vi "main.vi"() -> ()   [LabVIEW 2015]
uses:
  <userlib>/atmcd32d.llb/Error Code Enum typedef.ctl
  <vilib>/Utility/miscctls.llb/LVPointDoubleTypeDef.ctl
  <userlib>/atmcd32d.llb/OutputAmplifier_type typedef.ctl
  <vilib>/Xenics Infrared Solutions/Xeneth LabVIEW API/VIs/Controls/Camara.ctl
  <vilib>/Platform/TimedLoop/XDataNode/timing_clust.ctl
  <vilib>/Platform/TimedLoop/XDataNode/nitl_modes.ctl
  <vilib>/Platform/TimedLoop/XDataNode/wakeup.ctl
  <userlib>/atmcd32d.llb/HSSpeed_type typedef.ctl
  <userlib>/atmcd32d.llb/ReadMode_mode typedef.ctl
  <vilib>/Utility/file.llb/Read Delimited Spreadsheet (DBL).vi
  <vilib>/Utility/file.llb/Write Delimited Spreadsheet (DBL).vi
  <vilib>/Platform/TimedLoop/XDataNode/XDataNode.xnode
  <vilib>/Platform/TimedLoop/XDataNode/XDNodeRunTimeDep.lvlib
  <vilib>/Xenics Infrared Solutions/Xeneth LabVIEW API/Xeneth.lvlib
panel:
  in  "velleman-power":bool caption="Power Control"
  out "shutdown-complete":bool
  in  "shutdown":bool
  out "laser on":bool
  out "shutdown-active":bool
  in  "view settings":T1(tab)
  in  "abort-acquisition":bool caption="Abort"
  in  "measure":bool
  in  "NKT":bool
  in  "align-mode":bool caption="align mode"
  in  "continuos-save":bool
  in  "refresh display":bool=TRUE caption="refresh"
  in  "autoscale":bool=TRUE
  in  "background":bool=TRUE
  in  "Save current Spectrum":bool
  in  "File Name":string="spectrum"
  in  "BG shutter":T2(radio)=enum."with Open Shutter" caption="Shutter during background measurement"
  in  "select background":enum16{"skip", "single", "multiple"}(ring)=enum."single"
  out "Progress":u8(slide) scale=0.0..100.0
  out "ready":bool
  out "acquiring":bool
  out "background":bool
  out "measurement-finished":bool caption="finished"
  out "Acq Error":errorcluster
  out "next action":T3(ring)
  in  "Spectra":enum32{"Spectrum", "Image"}(tab)
  out "Data Plot":cluster{"wavelength array":sgl[], "array":i32[]}(graph)
  out "Detected Image":i32[][](graph)
  in  "Main Panel":T4(tab)=enum."init"
  in  "config":T5(tab)
  out "lightsource-set":bool
  out "NKT Output":T6 {"UV Wavelength (nm)" format="%.1f"; "Long Wavelength (nm)" format="%.1f"; "Short Wavelength (nm)" format="%.1f"; "Feedback Level" format="%.1f%%"; "Power Level" format="%.1f%%"; "Temp (°C)" format="%.1f"}
  in  "NKT Input":T7={"Emission"=FALSE, "Operation Mode"=FALSE, "Power Level"=5.0, "Feedback Level"=0.0, "Short Wavelength (nm)"=560.0, "Long Wavelength (nm)"=580.0, "UV Wavelength (nm)"=400.0} {"UV Wavelength (nm)" min=350.0 max=480.0 step=1.0 format="%.1f"; "Long Wavelength (nm)" min=400.0 max=850.0 step=0.5 format="%.1f"; "Short Wavelength (nm)" min=400.0 max=850.0 step=0.5 format="%.1f"; "Feedback Level" min=0.0 max=90.0 step=0.1 format="%.1f%%"; "Power Level" min=5.0 max=100.0 step=0.1 format="%.1f%%"}
  out "velleman-power-status":bool
  out "WL Power (nm)":i32 caption="Wavelength (nm)"
  out "Power (µW)":dbl format="%.6f"
  in  "Perform Auto Zero":bool
  in  "lightsource-bp":u16(ring) items=["(6,4)"=590, "(9,1)"=690, "(8,3)"=660, "(6,5)"=570, "(7,5)"=650, "--"=0]
  out "wavelength-limits":T8
  out "spectrograph-status":T9
  out "spectrograph-output":T10={"Slit Width (µm)"=50.0, "Grating"=3, "Central Wavelength (nm)"=1000.0, "Filter"=4, "Shutter"=0} caption="Spectrograph Output" {"Shutter" items=["Closed", "Open"]; "Slit Width (µm)" min=10.0 max=2500.0 step=0.1 format="%.1f"; "Grating" items=["500 blz 300l/mm"=1, "1200 blz 300l/mm"=2, "1250 blz 150l/mm"=3]; "Filter" items=["Empty"=5, "Longpass 900 nm"=4, "Longpass 715 nm"=3, "Longpass 475 nm"=2, "Longpass 320 nm"=1]; "Central Wavelength (nm)" min=200.0 max=2000.0 step=0.1 format="%.2f"}
  in  "spectrograph-input":T10={"Slit Width (µm)"=250.0, "Grating"=2, "Central Wavelength (nm)"=950.0, "Filter"=5, "Shutter"=1} caption="Spectrograph Input" {"Shutter" items=["Close", "Open"]; "Slit Width (µm)" min=10.0 max=2500.0 step=0.1 format="%.1f"; "Grating" items=["500 blz 300l/mm"=1, "1200 blz 300l/mm"=2, "1250 blz 150l/mm"=3]; "Filter" items=["Longpass 320 nm"=1, "Longpass 475 nm"=2, "Longpass 715 nm"=3, "Longpass 900 nm"=4, "Empty"=5]; "Central Wavelength (nm)" min=0.0 max=2000.0 step=0.1 format="%.1f"}
  out "spectrograph-reset-status":T11
  in  "spectrograph-reset-input":cluster{"grating":bool, "slit":bool}={"grating"=TRUE, "slit"=FALSE} caption="Spectrograph Reset Actions"
  in  "Exposure Time":dbl=0.20000000298023224 min=0.009999999776482582 step=0.009999999776482582 format="%.2f"
  out "Exposure Time Read":sgl format="%.2g"
  out "exposure time":bool
  out "detector":bool
  in  "Detector Select":u16(ring) caption="Camera" items=["Newton", "iDus", "Clara", "Xeva"]
  out "Current Detector":string
  in  "camera-settings":enum32{"Andor", "Xenics", "Andor-settings"}(tab)
  out "DLL error code":u32
  in  "iDus Type":T12
  in  "center":u16=102
  in  "height":u16=50 min=1 max=256
  in  "pre-amp 2":u8 caption="pre-amp" max=2 step=1
  in  "HBinning":u16(ring)=1 items=["1x"=1, "2x"=2, "4x"=4, "8x"=8, "16x"=16]
  out "binning":bool
  in  "HSSpeed 2":u8 max=0 step=1
  out "pre-amp 3":bool
  out "pre-amp":dbl caption="x"
  out "HSSpeed 3":bool
  out "HSSpeed":dbl caption="Mhz"
  out "ADchannel 2":bool
  in  "ADchannel":u8 max=0 step=1
  out "xeva-parameters":T13 {"time" format="%#.2f"}
  out "Cooling Read":cluster{"iDus":i32, "Newton":i32, "Clara":i32}={"iDus"=25, "Newton"=25, "Clara"=25}
  in  "detector-warmup":bool=TRUE
  in  "readout mode 2":u16(ring) items=["Full Vertical Binning", "Image", "Vertical Binning"]
  out "readout mode":bool
  out "nanostage moving":bool caption="moving"
  in  "z-stepsize":dbl=0.25 format="%.3f"
  in  "xy stepsize":dbl=0.1 format="%.3f"
  in  "x-axis":dbl=150.0 min=0.0 max=300.0 step=0.1 format="%.3f"
  in  "y-axis":dbl=150.0 min=0.0 max=300.0 step=0.1 format="%.3f"
  in  "z-axis":dbl=150.0 min=0.0 max=300.0 step=0.25 format="%.3f"
  in  "switch U/D":bool=TRUE
  in  "switch L/R":bool=TRUE
  out "stage-error":bool=TRUE
  out "click cursor position":T14
  out "getValues":cluster{"postion":dbl[], "status":bool[]} {"postion" format="%05.1f"}
  in  "stage-autozero":bool=TRUE caption="autozero on init"
  in  "laser-freeze":bool caption="glue scaling\nto image"
  in  "image-laser-position":T15={"laser-x-position"=520, "laser-y-position"=696}
  in  "magnification":dbl=83.3333333 caption="x" min=1.0 max=200.0 step=0.0001
  out "pixel scaling":bool
  out "Pixel Scaling":T16
  in  "laser-offset":bool caption="laser-is-zero"
  in  "magnification":bool
  in  "timed-shutdown":bool caption="shutdown"
  in  "timed-counter-stop":u32=1
  out "timed-counter":u32
  in  "timed-type":enum16{"spectrum", "AutoStage", "PLE"}(ring) caption="measurment type"
  out "waiting":u8(slide) scale=0.0..100.0
  in  "timed-start":bool caption="start"
  out "timed-timestamp":timestamp
  in  "timed-wait":dbl caption="wait / s"
  in  "cycle-save-coordinates":bool caption="save"
  in  "cycle-load-coordinates":bool caption="load"
  out "Coordinate Graph":dbl[][](graph)
  out "cycle-time":i32 caption="time/min"
  in  "cycle-iterator":i32 caption="iterator"
  out "cycle-num":i32 caption="total"
  out "Slide":u8(slide) scale=0.0..100.0
  in  "Cycle Cluster":T17={"cycle-x-mod"=151, "cycle-x-range-min"=0.0, "cycle-x-range-max"=300.0, "cycle-x-step"=4.0, "cycle-y-mod"=1, "cycle-y-range-min"=0.0, "cycle-y-range-max"=300.0, "cycle-y-step"=2.0, "cycle-z-mod"=0, "cycle-z-range-min"=150.0, "cycle-z-range-max"=0.0, "cycle-z-step"=0.0}
  in  "autostage-start":bool caption="start"
  in  "cycle-save-data":bool=TRUE caption="save"
  out "coordinates":dbl[][](array[numeric])
  in  "stage-timed-type":enum16{"spectrum", "PLE"}(ring) caption="measurment type"
  out "excitation":dbl[][](array[numeric])
  in  "PLE VIS/UV Panel":enum32{"SuperK Varia (VIS)"}(tab)
  in  "PLE Wavelength":T18={"WL Stepsize (nm)"=10, "WL Bandpass (nm)"=25, "Max WL VIS (nm)"=750, "Min WL VIS (nm)"=550} {"Min WL VIS (nm)" min=450 max=699 step=1; "Max WL VIS (nm)" min=501 max=850 step=1; "WL Bandpass (nm)" items=["5"=5, "10"=10, "25"=25, "50"=50, "75"=75, "100"=100]; "WL Stepsize (nm)" items=["5"=5, "10"=10, "25"=25, "50"=50, "75"=75, "100"=100]}
  out "PLE Acquisition\nfinished?":bool
  in  "Start PLE Scan":bool
  in  "PLE File Name":string="map" caption="File Name"
  out "Present Scan":string
  in  "STOP PLE":bool
  out "Acquisition Status PLE":T19=enum."DRV_NOT_INITIALIZED" caption="Acquisition Status"
  out "Elapsed Time (s)":dbl caption="elapsed time [s]" format="%.2f"
  out "Progress":dbl format="%.1f%%"
  out "Number of Scans":i32
  out "PLE-Map":i32[][](graph)
  out "PLE loop count":i32
  out "xeva init":bool caption="xeva"
  out "ANDOR init":bool caption="ANDOR"
  out "velleman init":bool caption="velleman"
  out "cameras init":bool caption="cameras"
  out "nanostage init":bool caption="nanostage"
  out "lightsource":bool
  out "powermeter init":bool caption="powermeter"
  out "spectrograph":bool
  in  "init xeva":bool caption="xeva"
  in  "init cameras":bool caption="cameras"
  in  "init spectrograph":bool caption="spectrograph"
  in  "init powermeter":bool caption="powermeter"
  in  "init nanostage":bool caption="nanostage"
  in  "init lightsource":bool caption="lightsource"
  in  "Cooling Set":T20={"iDus"=FALSE, "idus-temp"=-90, "Newton"=FALSE, "newton-temp"=-70, "Clara"=FALSE, "clara-temp"=-55, "Xeva"=FALSE, "xeva-temp"=-70} {"xeva-temp" min=-70 max=20 step=5; "clara-temp" min=-55 max=20 step=5; "newton-temp" min=-90 max=20 step=5; "idus-temp" min=-90 max=20 step=5}
  out "general-camera-status":T21
  in  "Tab Control":T22(tab)
  out "xeva-camref":T23
  in  "lightsource-visa":refnum<visa-resource-name>="COM3"
  in  "powermeter visa":refnum<visa-resource-name>="USB0::0x1313::0x8079::P1000487::INSTR"
  out "CCD Handle":i32
  out "InGaAs Handle":i32
  out "All conn. axes":string[](array[string])
  out "Handle":cluster{"iDus":i32, "Newton":i32, "Clara":i32} caption="Handle Cluster"
  out "Background Array":i32[](array[numeric])
  out "Raw Signal Array":i32[](array[numeric])
  out "Background Array PLE":i32[](array[numeric])
  out "Raw Signal Array PLE":i32[](array[numeric])
  out "Power during measurement":dbl format="%#_13g"
  out "y-scale array":sgl[](array[numeric])
  out "x-scale array":sgl[](array[numeric])
  out "stage error message":string
  out "error out":errorcluster
  out "xenics-status-cluster":T24
  out "andor-status-cluster":T25={"Newton Init"=FALSE, "Newton Cooling"=FALSE, "Newton Parameters "=FALSE, "iDus Init"=FALSE, "iDus Cooling"=FALSE, "iDus Parameters"=FALSE, "Clara Init"=FALSE, "Clara Cooling"=FALSE, "Clara Parameters"=FALSE, "Newton Cooler StatusCode"=enum."DRV_TEMPERATURE_NOT_SUPPORTED", "iDus Cooler StatusCode"=enum."DRV_TEMPERATURE_NOT_SUPPORTED", "Clara Cooler StatusCode"=enum."DRV_TEMPERATURE_NOT_SUPPORTED"} caption="Cooling Status"
  # "Powermeter Status"
  # "spectrograph reset"
  # "Cycle"
  # "step\n[µm]"
  # "cycle mod"
  # "range\n[µm]"
  # "x-axis"
  # "y-axis"
  # "z-axis"
  # "Central Wavelength (nm)"
  # "Init"
  # "Cooling"
  # "Parameters"
  # "Newton"
  # "iDus"
  # "Clara"
  # "Xeva"
  # "Init"
  # "Cooling"
  # "Parameters"
  # "Xeva"
  # "Init"
  # "Cooling"
  # "Parameters"
  # "Newton"
  # "iDus"
  # "Clara"
  # "Clara"
  # "iDus"
  # "Newton"
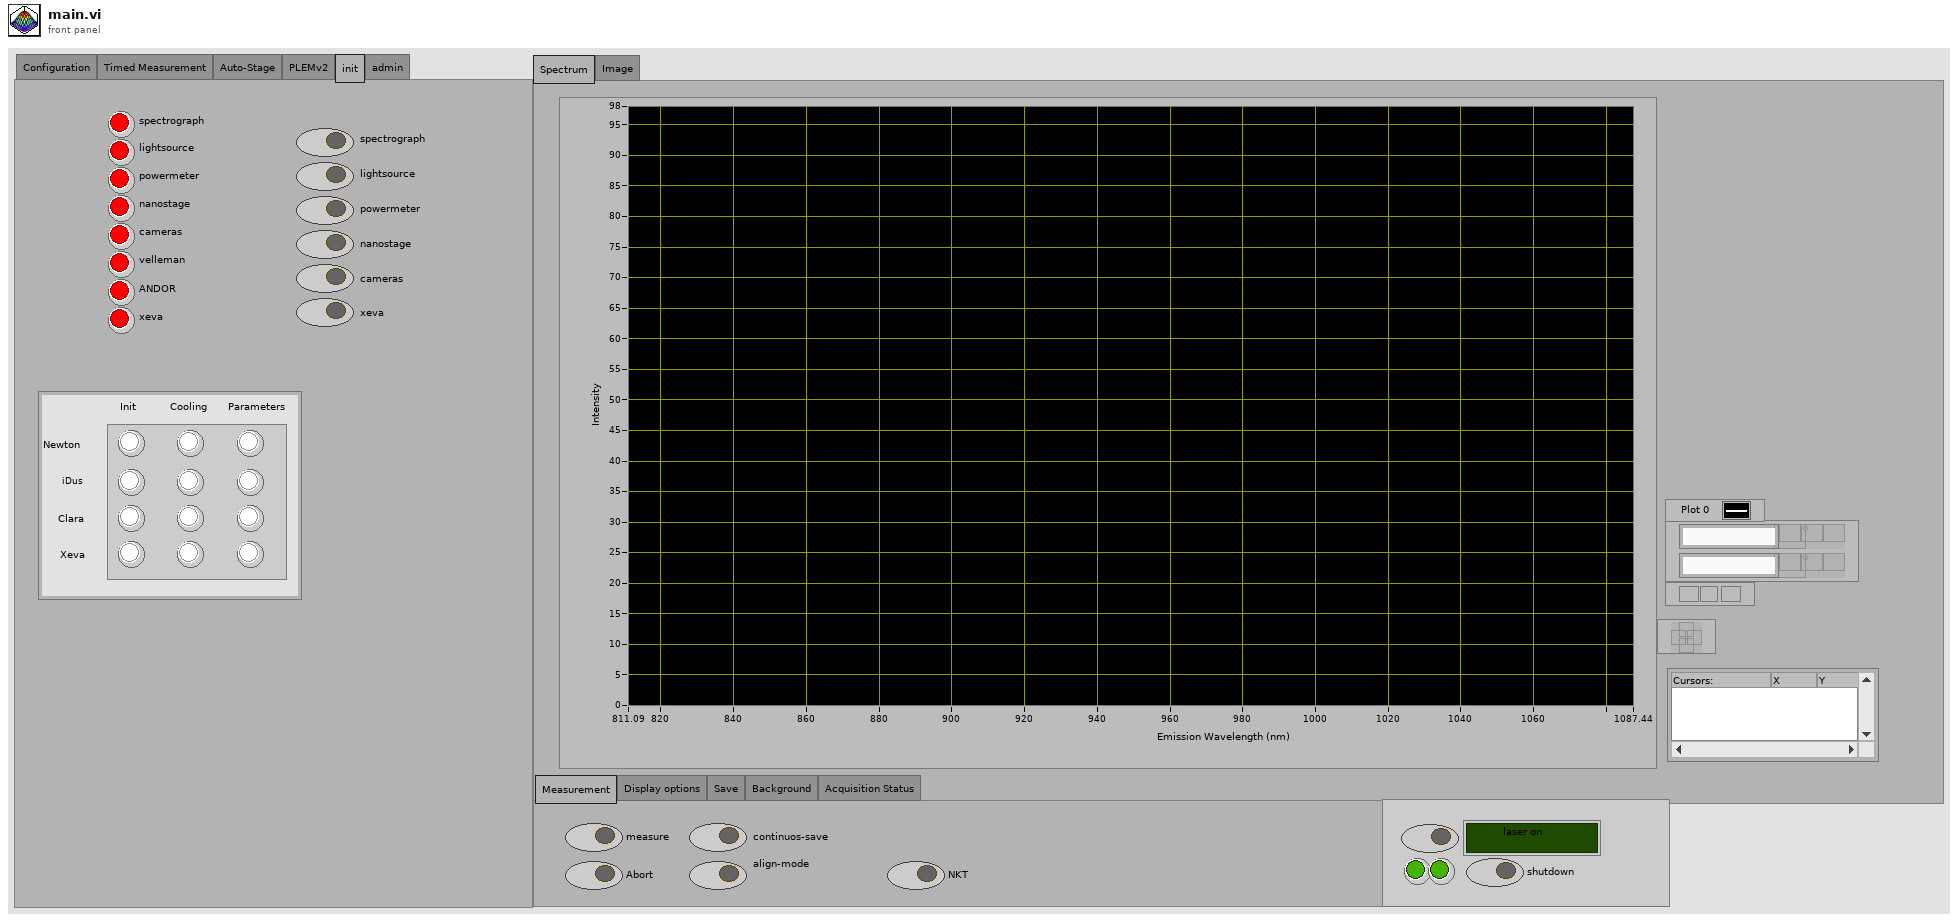
[diagram p1: front panel]
types:
  T1 = enum32{"Measurement", "Display options", "Save", "Background", "Acquisition Status"}
  T2 = enum32{"with Closed Shutter", "with Open Shutter"}
  T3 = enum16{"noop", "set background", "set measurement", "start acquisition", "abort", "get Data", "check progress", "restart acquisition", "start", "acquisition finished", "measurement finished", "wait to continue"}
  T4 = enum32{"Configuration", "Timed Measurement", "Auto-Stage", "PLEMv2", "init", "admin"}
  T5 = enum32{"Lightsource", "Spectrograph", "Camera", "Nanostage", "image"}
  T6 = cluster{"Emission":bool, "Operation Mode":string, "Power Level":dbl, "Feedback Level":dbl, "Short Wavelength (nm)":dbl, "Long Wavelength (nm)":dbl, "UV Wavelength (nm)":dbl, "Temp (°C)":dbl}
  T7 = cluster{"Emission":bool, "Operation Mode":bool, "Power Level":dbl, "Feedback Level":dbl, "Short Wavelength (nm)":dbl, "Long Wavelength (nm)":dbl, "UV Wavelength (nm)":dbl}
  T8 = cluster{"wl-start":dbl, "wl-step":dbl, "wl-end":dbl}
  T9 = cluster{"Slit":bool, "Diffraction Grating":bool, "Central Wavelength":bool, "Filter":bool, "Shutter":bool}
  T10 = cluster{"Slit Width (µm)":dbl, "Grating":u16, "Central Wavelength (nm)":dbl, "Filter":u16, "Shutter":u16}
  T11 = cluster{"Wavelength Reset OK":bool, "Slit Reset OK":bool}
  T12 = typedef "OutputAmplifier_type typedef.ctl" = enum16{"Standard EMCCD gain register", "Conventional CCD register"}
  T13 = cluster{"width":u32, "height":u32, "time":dbl, "temperature":dbl, "temperature-setpoint":dbl}
  T14 = typedef "LVPointDoubleTypeDef.ctl" = cluster{"X":dbl, "Y":dbl}
  T15 = cluster{"laser-x-position":u16, "laser-y-position":u16}
  T16 = cluster{"first x":sgl, "size x":u16, "deltax":dbl, "first y":sgl, "size y":u16, "deltay":dbl, "unit":string}
  T17 = cluster{"cycle-x-mod":i32, "cycle-x-range-min":dbl, "cycle-x-range-max":dbl, "cycle-x-step":dbl, "cycle-y-mod":i32, "cycle-y-range-min":dbl, "cycle-y-range-max":dbl, "cycle-y-step":dbl, "cycle-z-mod":i32, "cycle-z-range-min":dbl, "cycle-z-range-max":dbl, "cycle-z-step":dbl}
  T18 = cluster{"WL Stepsize (nm)":i32, "WL Bandpass (nm)":u16, "Max WL VIS (nm)":i32, "Min WL VIS (nm)":i32}
  T19 = typedef "Error Code Enum typedef.ctl" = enum32{"N/A (0)", "DRV_ERROR_CODES", "DRV_SUCCESS", "DRV_VXDNOTINSTALLED", "DRV_ERROR_SCAN", "DRV_ERROR_CHECK_SUM", "DRV_ERROR_FILELOAD", "DRV_UNKNOWN_FUNC", "DRV_ERROR_VXD_INIT", "DRV_ERROR_ADDRESS", "DRV_ERROR_PAGELOCK", "DRV_ERROR_PAGEUNLOCK", "DRV_ERROR_BOARDTEST", "DRV_ERROR_ACK", "DRV_ERROR_UP_FIFO", "DRV_ERROR_PATTERN", "N/A (16)", "DRV_ACQUISITION_ERRORS", "DRV_ACQ_BUFFER", "DRV_ACQ_DOWNFIFO_FULL", "DRV_PROC_UNKONWN_INSTRUCTION", "DRV_ILLEGAL_OP_CODE", "DRV_KINETIC_TIME_NOT_MET", "DRV_ACCUM_TIME_NOT_MET", "DRV_NO_NEW_DATA", "N/A (25)", "DRV_SPOOLERROR", "N/A (27)", "N/A (28)", "N/A (29)", "N/A (30)", "N/A (31)", "N/A (32)", "DRV_TEMPERATURE_CODES", "DRV_TEMPERATURE_OFF", "DRV_TEMPERATURE_NOT_STABILIZED", "DRV_TEMPERATURE_STABILIZED", "DRV_TEMPERATURE_NOT_REACHED", "DRV_TEMPERATURE_OUT_RANGE", "DRV_TEMPERATURE_NOT_SUPPORTED", "DRV_TEMPERATURE_DRIFT", "N/A (41)", "N/A (42)", "N/A (43)", "N/A (44)", "N/A (45)", "N/A (46)", "N/A (47)", "N/A (48)", "DRV_GENERAL_ERRORS", "DRV_INVALID_AUX", "DRV_COF_NOTLOADED", "DRV_FPGAPROG", "DRV_FLEXERROR", "DRV_GPIBERROR", "N/A (55)", "N/A (56)", "N/A (57)", "N/A (58)", "N/A (59)", "N/A (60)", "N/A (61)", "N/A (62)", "N/A (63)", "DRV_DATATYPE", "DRV_DRIVER_ERRORS", "DRV_P1INVALID", "DRV_P2INVALID", "DRV_P3INVALID", "DRV_P4INVALID", "DRV_INIERROR", "DRV_COFERROR", "DRV_ACQUIRING", "DRV_IDLE", "DRV_TEMPCYCLE", "DRV_NOT_INITIALIZED", "DRV_P5INVALID", "DRV_P6INVALID", "DRV_INVALID_MODE", "DRV_INVALID_FILTER", "DRV_I2CERRORS", "DRV_I2CDEVNOTFOUND", "DRV_I2CTIMEOUT", "DRV_P7INVALID", "N/A (84)", "N/A (85)", "N/A (86)", "N/A (87)", "N/A (88)", "N/A (89)", "DRV_IOCERROR", "DRV_VRMVERSIONERROR"}
  T20 = cluster{"iDus":bool, "idus-temp":i32, "Newton":bool, "newton-temp":i32, "Clara":bool, "clara-temp":i32, "Xeva":bool, "xeva-temp":i32}
  T21 = cluster{"Newton Init":bool, "Newton Cooling":bool, "Newton Parameters ":bool, "iDus Init":bool, "iDus Cooling":bool, "iDus Parameters":bool, "Clara Init":bool, "Clara Cooling":bool, "Clara Parameters":bool, "Xeva-init":bool, "xeva-cooling":bool, "xeva-parameters":bool}
  T22 = enum32{"ref/visa", "variables", "data", "status"}
  T23 = typedef "Xeneth.lvlib/Camara.ctl" = refnum<k1>
  T24 = cluster{"Xeva-init":bool, "xeva-cooling":bool, "xeva-parameters":bool, "xeva-error":string}
  T25 = cluster{"Newton Init":bool, "Newton Cooling":bool, "Newton Parameters ":bool, "iDus Init":bool, "iDus Cooling":bool, "iDus Parameters":bool, "Clara Init":bool, "Clara Cooling":bool, "Clara Parameters":bool, "Newton Cooler StatusCode":T19, "iDus Cooler StatusCode":T19, "Clara Cooler StatusCode":T19}
  T26 = typedef "XDNodeRunTimeDep.lvlib/timing_clust.ctl" = cluster{"Expected End [f-1]":u64, "Actual End [f-1]":u64, "Finished Late? [f-1]":bool, "Expected End [i-1]":u64, "Actual End [i-1]":u64, "Finished Late? [i-1]":bool, "Expected Start [i]":u64, "Actual Start [i]":u64, "Expected Start [f]":u64, "Actual Start [f]":u64, "Source Name":string, "Structure Name":string, "Period":i64, "Deadline":i64, "Offset":i64, "Start":i64, "Priority":i32, "Timeout":i32, "Mode":T27, "Wakeup Reason":T28, "Error":errorcluster, "Source Type":string, "Secondary Source Type":string, "Global End Time":u64, "Global Start Time":u64, "Frame Duration":u64, "Iteration Duration":u64, "Assigned CPU":i32, "I/O Scan Engine Mode":u32}
  T27 = typedef "XDNodeRunTimeDep.lvlib/nitl_modes.ctl" = enum32{"No Change", "Process missed periods, maintain original phase", "Discard missed periods, maintain original phase", "Process missed periods, ignore original phase", "Discard missed periods, ignore original phase"}
  T28 = typedef "XDNodeRunTimeDep.lvlib/wakeup.ctl" = enum32{"Normal", "Aborted", "Asynchronous wakeup", "Timing source error", "Timed loop error", "Timeout"}
  T29 = cluster{"Wavelength Reset":bool, "Slit Reset":bool}
  T30 = typedef "HSSpeed_type typedef.ctl" = enum16{"EM Amp", "Conventional Amp"}
  T31 = enum8{"Enabled", "Disabled", "Disabled and Grayed Out"}
  T32 = typedef "ReadMode_mode typedef.ctl" = enum16{"Full Vertical Binning", "Multi-Track", "Random-Track", "Single-Track", "Image"}
  T33 = cluster{"Slit Width (µm)":dbl, "Diffraction Grating":u16, "Central Wavelength (nm)":dbl, "Filter":u16, "Shutter":u16}
  T34 = cluster{"Slit":bool, "Diffraction Grating":bool, "Filter":bool, "Central Wavelength":bool, "Shutter":bool}
  T35 = cluster{"Emission On/Off external":bool, "Feedback Level external":dbl, "Power/Feedback Mode external":bool, "Power Level external":dbl}
  T36 = cluster{"Emission On/Off external":bool, "Feedback Level external":bool, "Power/Feedback Mode external":bool, "Power Level external":bool}
  T37 = cluster{"Slit Width (µm)":bool, "Grating":bool, "Central Wavelength (nm)":bool, "Filter":bool, "Shutter":bool}
  T38 = cluster{bool, bool, bool, "Filter":bool, "Shutter":bool}
  T39 = enum32{"Lightsource", "Spectrograph", "Detectors", "Nanostage", "image"}
  T40 = cluster{"Newton Init":bool, "Newton Cooling":bool, "Newton Parameters ":bool, "iDus Init":bool, "iDus Cooling":bool, "iDus Parameters":bool, "Clara Init":bool, "Clara Cooling":bool, "Clara Parameters":bool, "Newton Cooler StatusCode":bool, "iDus Cooler StatusCode":bool, "Clara Cooler StatusCode":bool}
  T41 = cluster{"Xeva-init":bool, "xeva-cooling":bool, "xeva-parameters":bool, "xeva-error":bool}
  T42 = typedef "LVPoint32TypeDef.ctl" = cluster{"Horizontal":i32, "Vertical":i32}
  T43 = cluster{"acquiring out":bool, "Progress":u8, "background":bool, "timer":u32, "finished":bool}
  T44 = enum16{"noop", "set background", "set measurement", "start acquisition", "abort", "get Data", "check progress", "restart acquisition", "start", "finished"}
  T45 = cluster{"detector":u16, "HBinning":u16, "readout mode":u16, "ready":bool, "Exposure Time Read":sgl, "select background":enum16{"skip", "single", "multiple"}, "xeva-camref":T23}
  T46 = enum16{"noop", "set background", "set measurement", "start acquisition", "abort", "get Data", "check progress", "restart acquisition", "start"}
  T47 = enum16{"noop", "set background", "set measurement", "start acquisition", "abort", "get Data", "check progress", "restart acquisition", "start", "acquisition finished", "start next measurement", "wait to continue"}
  T48 = cluster{"laser-x-position":bool, "laser-y-position":bool}
  T49 = cluster{"x-axis":dbl, "y-axis":dbl, "z-axis":dbl}
  T50 = cluster{"x-axis":bool, "y-axis":bool, "z-axis":bool}
  T51 = cluster{"Emission":bool, "Operation Mode":bool, "Power Level":bool, "Feedback Level":bool, "Short Wavelength (nm)":bool, "Long Wavelength (nm)":bool, "UV Wavelength (nm)":bool}
  T52 = cluster{"x-scale array":sgl[], "Raw Signal Array":i32[]}
  T53 = cluster{"cycle-x-mod":bool, "cycle-x-range-min":bool, "cycle-x-range-max":bool, "cycle-x-step":bool, "cycle-y-mod":bool, "cycle-y-range-min":bool, "cycle-y-range-max":bool, "cycle-y-step":bool, "cycle-z-mod":bool, "cycle-z-range-min":bool, "cycle-z-range-max":bool, "cycle-z-step":bool}
  T54 = cluster{"image-laser-position":cluster{"laser-x-position":u16, "laser-y-position":u16}, "magnification":dbl}
  T55 = cluster{"x-axis":dbl, "y-axis":dbl, "z-axis":dbl, "switch U/D":bool, "switch L/R":bool}
  T56 = cluster{"Current Detector":string, "readout mode":u16, "Hbinning":u16, "Exposure Time":sgl, "Cooling Read":cluster{"iDus":i32, "Newton":i32, "Clara":i32}, "pre-amp":dbl, "HSSpeed":dbl}
  T57 = cluster{"BG shutter":enum32{"with Closed Shutter", "with Open Shutter"}, "select background":enum16{"skip", "single", "multiple"}}
  T58 = cluster{"Loop Indicator":i32, "Number of Scans":i32, "True Step Size (nm) ":i32, "Wavelength Bandpass (nm)":i32, "Min Central Wavelength (nm)":i32}
  T59 = cluster{"Calibration Mode":bool, "File Name":string, "User Name":string, "Aborted?":bool, "NKT System":enum32{"SuperK Varia (VIS)", "Extend-UV"}}
  T60 = cluster{"Min WL VIS (nm)":i32, "Max WL VIS (nm)":i32, "WL Bandpass (nm)":i32, "WL Stepsize (nm)":i32}
  T61 = cluster{"Min Central Wavelength (nm)":i32, "Wavelength Bandpass (nm)":i32, "True Step Size (nm) ":i32, "Number of Scans":i32}
  T62 = cluster{"wavelength array":sgl[], "Data To Plot Array":i32[], "Raw Signal Array PLE":i32[], "Background Array PLE":i32[]}
  T63 = cluster{"WL Stepsize (nm)":i32, "Max WL VIS (nm)":i32, "Max WL VIS (nm)":i32, "Min WL VIS (nm)":i32}
  T64 = cluster{"WL Stepsize (nm)":bool, bool, "Max WL VIS (nm)":bool, "Min WL VIS (nm)":bool}
  T65 = cluster{"Emission":bool, "Operation Mode":string, "Power Level":dbl, "Feedback Level":dbl, "Short Wavelength (nm)":i32, "Long Wavelength (nm)":i32, "UV Wavelength (nm)":i32, "Temp (°C)":dbl}
  T66 = cluster{"Min Central Wavelength (nm)":i32, "Wavelength Bandpass (nm)":i32, "True Step Size (nm) ":i32, "Number of Scans":i32, i32}
  T67 = cluster{"Min Central Wavelength (nm)":i32, "Wavelength Bandpass (nm)":i32, "True Step Size (nm) ":i32, "Number of Scans":i32, "Loop Indicator":i32}
  T68 = cluster{"UV Wavelength (nm)":i32, "Short Wavelength (nm)":dbl, "Long Wavelength (nm)":dbl}
  T69 = cluster{"x-scale array":sgl[], "Background Array PLE":i32[]}
  T70 = cluster{"wavelength array":sgl[], "Data To Plot Array":i32[]}
  T71 = cluster{"Y Scale.Flipped":bool, "color table":u32[], dbl, dbl, dbl, dbl, sgl, sgl, sgl, dbl, "new picture":picture}
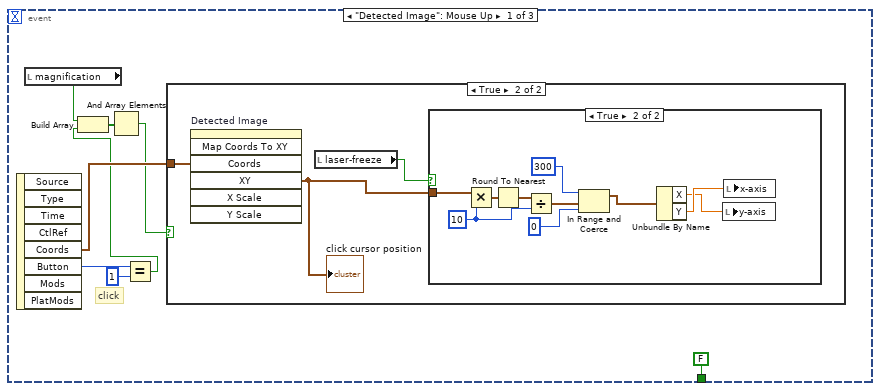
[diagram p2: hidden frame]
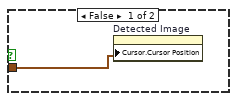
[diagram p4: hidden frame]
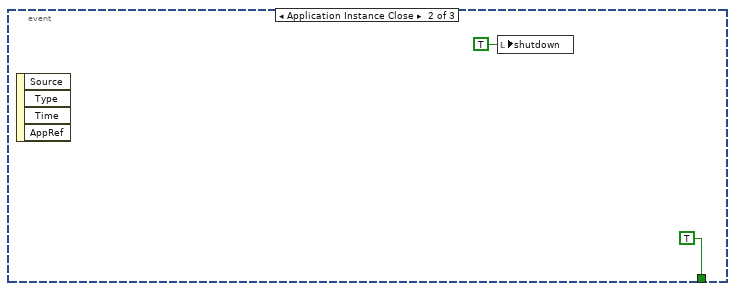
[diagram p5: hidden frame]
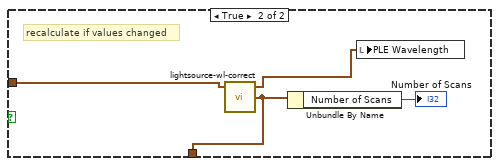
[diagram p7: hidden frame]
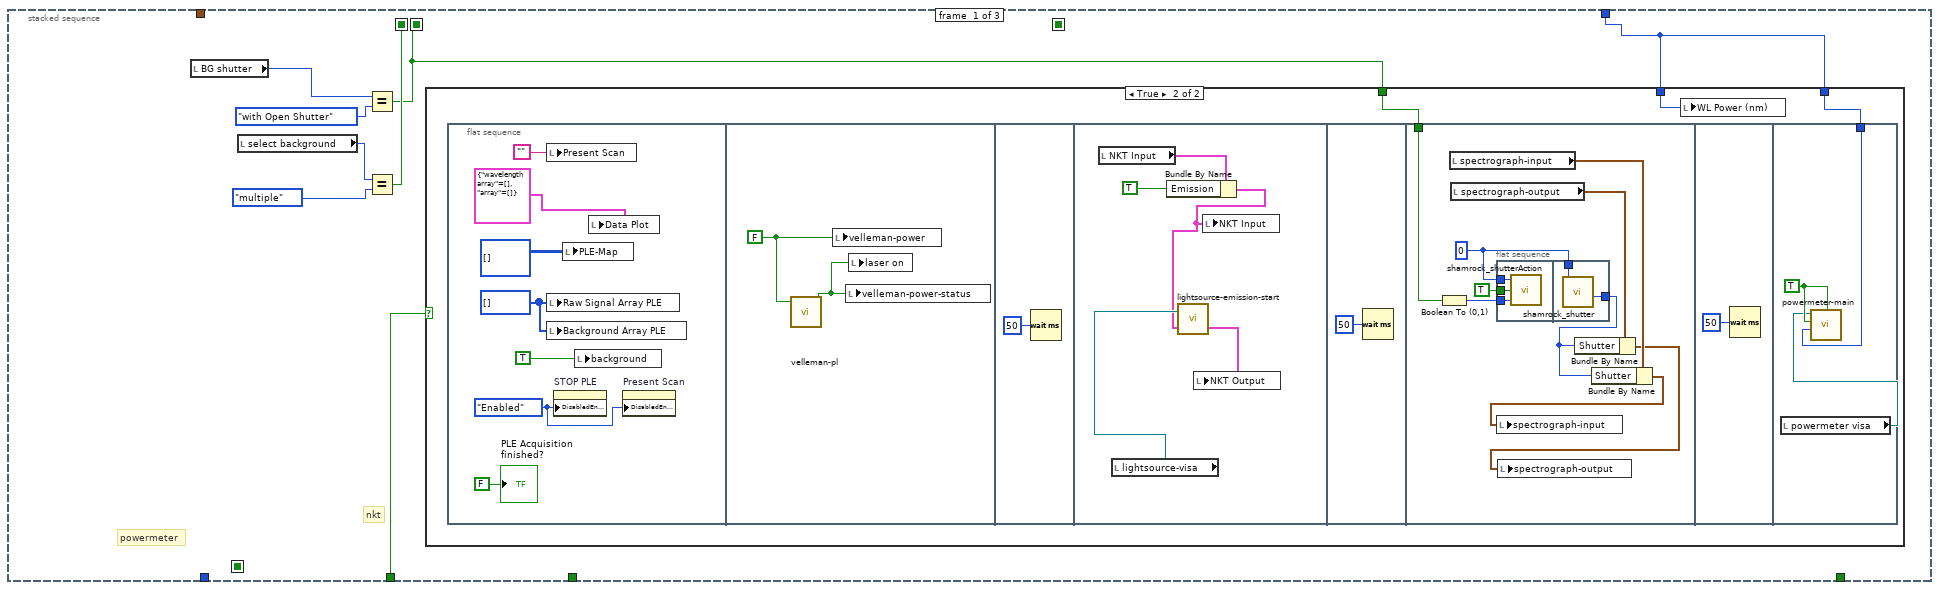
[diagram p9: hidden frame]
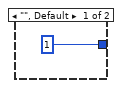
[diagram p11: hidden frame]
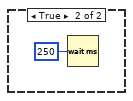
[diagram p12: hidden frame]
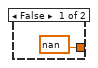
[diagram p13: hidden frame]
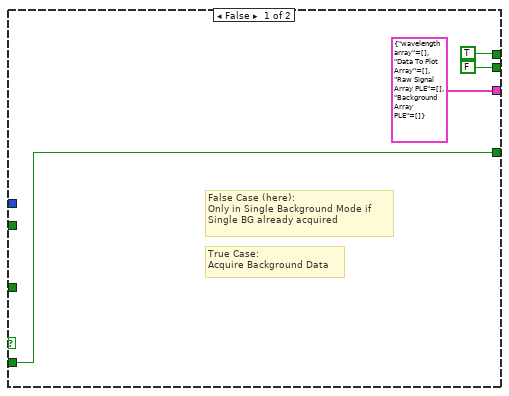
[diagram p14: hidden frame]
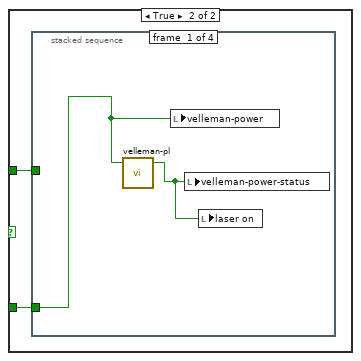
[diagram p16: hidden frame]
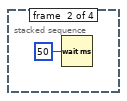
[diagram p17: hidden frame]
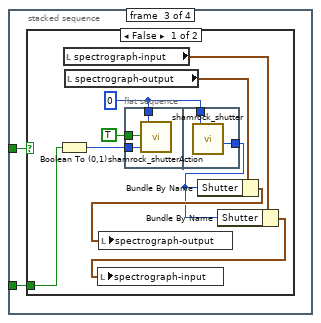
[diagram p18: hidden frame]
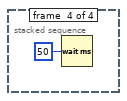
[diagram p20: hidden frame]
diagram:
  # "Events\n* move cursor\n* app close"
  # "Device Control\n* Init\n* Set Parameters\n* Close"
  # "GUI\n* Controls\n* Data Display\n* Events"
  # "Measurement:\n* Data Acquisition\n* Measurement Programs\n* PLE Program"
  n1 = node-c288() -> (w12:T26)  [unwired: 4 in]
  n2 = node-c288(i64 100 ("Period")) -> (w16:T26)  [unwired: 3 in]
  n3 = flat-sequence {
    frame #0 {
      w21 = FALSE ("detectors")
      n4 = local write "cameras init"(w21) -> ()
      n5 = local write "nanostage init"(w21) -> ()
      n6 = local write "powermeter init"(w21) -> ()
      n7 = local write "lightsource"(w21) -> ()
      n8 = local write "spectrograph"(w21) -> ()
      n9 = local write "velleman init"(w21) -> ()
      n10 = local write "xeva init"(w21) -> ()
    }
    frame #1 {
      n11 = node-c288() -> (w23:T26)  [unwired: 4 in]
      n12 = timed-loop {
        timing: w23 -> [_]
        timing-out: [_] -> w22
        stop <- w24 continue-if-true
        # "main loop"
        n13 = flat-sequence {
          tunnel: [w972] -> w24
          frame #0 {
            # "Init All Devices"
            n14 = local read "spectrograph"() -> (w51:bool)
            n15 = local read "nanostage init"() -> (w44:bool)
            n16 = Not(x=w51) -> (.not. x?=w50:bool)
            n17 = Not(x=w44) -> (.not. x?=w45:bool)
            n18 = And(x="init nanostage", y=w45) -> (x .and. y?=w47:bool)
            n19 = And(x="init spectrograph", y=w50) -> (x .and. y?=w48:bool)
            n20 = case shown="False" w47 {
              frame False {
              }
              frame True {
                n21 = while {
                  tunnel: [w133] -> w97
                  tunnel: [w132] -> w98
                  stop <- w128 continue-if-true
                  # "init nanostage\nloop until init has no error"
                  n22 = flat-sequence {
                    tunnel: [w136] -> w131
                    tunnel: [w135] -> w130
                    tunnel: [w139] -> w132
                    tunnel: [w138] -> w133
                    tunnel: w131 -> [w138]
                    tunnel: w130 -> [w139]
                    tunnel: [w137] -> w126
                    frame #0 {
                      n23 = call "nanostage-init.vi"("Perform autozero?"="stage-autozero") -> ("error out"=w136:errorcluster, "All conn. axes"=w135:string[])  [unwired: 3 in]
                    }
                    frame #1 {
                      n24 = Unbundle By Name(w138) -> ("status"=w137:bool)
                      n25 = local write "stage-error"(w137) -> ()
                    }
                  }
                  n26 = local read "init nanostage"() -> (w127:bool)
                  n27 = Build Array(w126, w127) -> (w129:bool[])
                  n28 = And Array Elements(Boolean array=w129) -> (logical AND=w128:bool)
                }
                "All conn. axes" <- w98
                n29 = case shown="No Error" w97 {
                  selector: w97 -> [_ w123]
                  tunnel: w98 -> [w99 w122]
                  frame No Error {
                    n30 = stacked-sequence {
                      tunnel: w99 -> [w101 w111 _]
                      frame #0 {
                        # "set voltages to zero (servo mode is turned off)"
                        n31 = case shown="False" FALSE {
                          selector: FALSE -> [_ w102]
                          tunnel: w101 -> [_ w105]
                          frame False {
                          }
                          frame True {
                            n32 = call "nanostage-reset.vi"("reset stage"=w102, "All conn. axes"=w105) -> ("error out"=w104:errorcluster, "Error Description"=w103:string)  [unwired: 2 in]
                            n33 = case shown="Error" w104 {
                              tunnel: w103 -> [_ w106]
                              frame No Error {
                              }
                              frame Error {
                                n34 = local write "stage error message"(w106) -> ()
                              }
                            }
                          }
                        }
                      }
                      frame #1 {
                        # "init to last position"
                        n35 = call "nanostage-readonly.vi"("Axes to move"=w111) -> ("error out"=w110:errorcluster, "position-z"=w107:dbl, "position-y"=w108:dbl, "position-x"=w109:dbl)  [unwired: 3 in]
                        n36 = case shown="No Error" w110 {
                          tunnel: w109 -> [w118 _]
                          tunnel: w108 -> [w116 _]
                          tunnel: w107 -> [w115 _]
                          frame No Error {
                            n37 = local read "switch U/D"() -> (w119:bool)
                            n38 = local read "switch L/R"() -> (w117:bool)
                            n39 = call "utility-flip-stage.vi"("axis in"=w116, "flip"=w117) -> ("axis out"=w113:dbl)
                            n40 = call "utility-flip-stage.vi"("axis in"=w118, "flip"=w119) -> ("axis out"=w114:dbl)
                            n41 = local write "config"(T5."Nanostage" ("config")) -> ()
                            n42 = local write "z-axis"(w115) -> ()
                            n43 = local write "x-axis"(w114) -> ()
                            n44 = local write "y-axis"(w113) -> ()
                          }
                          frame Error {
                          }
                        }
                      }
                      frame #2 {
                        n45 = local write "nanostage init"(TRUE ("nanostage init")) -> ()
                      }
                    }
                  }
                  frame Error {
                    n46 = call "nanostage-health.vi"("error in"=w123, "All conn. axes"=w122) -> ("error"=w124:bool, "error message"=→"stage error message":string)
                    n47 = Not(x=w124) -> (.not. x?=→"nanostage init":bool)
                    n48 = local write "stage-error"(w124) -> ()
                  }
                }
              }
            }
            n49 = case shown="True" w48 {
              frame False {
              }
              frame True {
                n50 = flat-sequence {
                  tunnel: [w76] -> w75
                  tunnel: w75 -> [w86]
                  tunnel: [w85] -> w73
                  tunnel: [w88] -> w74
                  tunnel: w73 -> [w88]
                  tunnel: w74 -> [w91]
                  frame #0 {
                    # "Initializiation \nShamrock \nSpectrograph"
                    n51 = call <userlib>:"shamrock_initialize.vi"() -> ()  [unwired: 1 in, 3 out]
                  }
                  frame #1 {
                    w78 = "SR1278"  # Serial Number of Shamrock spectrograph
                    w79 = 0  # Device No
                    n52 = call <userlib>:"shamrock_info.vi"("Device No"=w79) -> ("Serial Number"=w77:string)  [unwired: 5 out]
                    n53 = Equal?(x=w78, y=w77) -> (x = y?=w76:bool)
                  }
                  frame #2 {
                    # "maybe this frame can be deleted"
                    n54 = local read "spectrograph-reset-input"() -> (w83:cluster{"grating":bool, "slit":bool})
                    n55 = local read "spectrograph-input"() -> (w84:T10)
                    n56 = call "spectrometer-config.vi"("Spectrograph Input Cluster"=w84, "Initialization Successful?"=w86, "Spectrograph Reset Cluster"=w83) -> ("Reset Control Cluster"=w80:T29, "Spectrograph Output Cluster"=w82:T33, "Configuration Successful?"=w85:bool, "Output Control Cluster"=w81:T34)  [unwired: 1 in]
                    n57 = local write "spectrograph-reset-status"(w80) -> ()
                    n58 = local write "spectrograph-status"(w81) -> ()
                    n59 = local write "spectrograph-output"(w82) -> ()
                  }
                  frame #3 {
                    n60 = local write "pixel scaling"(FALSE ("pixel scaling")) -> ()
                    n61 = local write "spectrograph-reset-input"(T29 {"Wavelength Reset"=FALSE, "Slit Reset"=FALSE} ("Spectrograph Reset Cluster")) -> ()
                    n62 = local write "config"(T5."Spectrograph" ("config")) -> ()
                    "spectrograph" <- w88
                  }
                  frame #4 {
                    n63 = case shown="True" w91 {
                      frame False {
                      }
                      frame True {
                        # "ANDOR\nSystem\nactive"
                        "ANDOR init" <- TRUE ("ANDOR")
                      }
                    }
                  }
                }
              }
            }
            n64 = local read "powermeter init"() -> (w43:bool)
            n65 = local read "lightsource"() -> (w38:bool)
            n66 = local read "cameras init"() -> (w34:bool)
            n67 = local read "xeva init"() -> (w30:bool)
            n68 = Not(x=w34) -> (.not. x?=w35:bool)
            n69 = Not(x=w30) -> (.not. x?=w31:bool)
            n70 = Not(x=w38) -> (.not. x?=w37:bool)
            n71 = And(x="init cameras", y=w35) -> (x .and. y?=w32:bool)
            n72 = Not(x=w43) -> (.not. x?=w42:bool)
            n73 = case shown="True" w32 {
              frame False {
              }
              frame True {
                n74 = flat-sequence {
                  tunnel: [w67] -> w61
                  tunnel: w61 -> [w69]
                  frame #0 {
                    n75 = call "detector-init.vi"("Cooling Set"="Cooling Set") -> ("Status"=→"andor-status-cluster":T25, "cameras initialized"=w67:bool, "Handle Cluster"=w66:cluster{"iDus":i32, "Newton":i32, "Clara":i32}, "Detector Output Values"=→"Cooling Read":cluster{"iDus":i32, "Newton":i32, "Clara":i32})  [unwired: 1 in]
                    "cameras init" <- w67
                    "Handle" <- w66
                    n76 = Unbundle By Name(w66) -> ("iDus"=→"InGaAs Handle":i32, "Newton"=→"CCD Handle":i32)
                  }
                  frame #1 {
                    n77 = case shown="True" w69 {
                      frame False {
                      }
                      frame True {
                        # "ANDOR\nSystem\nactive"
                        n78 = local write "ANDOR init"(TRUE ("ANDOR")) -> ()
                        n79 = local write "config"(T5."Camera" ("config")) -> ()
                      }
                    }
                  }
                  frame #2 {
                    n80 = local write "exposure time"(FALSE ("exposure time")) -> ()
                  }
                }
              }
            }
            n81 = And(x="init xeva", y=w31) -> (x .and. y?=w28:bool)
            n82 = And(x="init powermeter", y=w42) -> (x .and. y?=w40:bool)
            n83 = And(x="init lightsource", y=w37) -> (x .and. y?=w39:bool)
            n84 = case shown="True" w28 {
              frame False {
              }
              frame True {
                n85 = call "xeva-init.vi"() -> ("error out"=w54:errorcluster, "initialized"=w53:bool, "xeva-camref"=w52:T23)  [unwired: 3 in]
                n86 = case shown="No Error" w54 {
                  tunnel: w53 -> [w58 _]
                  tunnel: w52 -> [w59 _]
                  frame No Error {
                    w55 = u16 1 items=["Full Vertical Binning", "Image", "Vertical Binning"] ("readout mode 2")
                    # "combine them wiht andor settings\nfrom first fram in set camera (andro)"
                    n87 = local read "Cooling Set"() -> (w60:T20)
                    n88 = call "xeva-setcooling.vi"("Cooling Set"=w60, "xeva init"=w58, "xeva-camref"=w59) -> ("xenics-status-cluster"=→"xenics-status-cluster":T24)  [unwired: 7 in, 1 out]
                    n89 = local write "exposure time"(FALSE ("exposure time")) -> ()
                    n90 = local write "readout mode 2"(w55) -> ()
                    "xeva init" <- w58
                    "xeva-camref" <- w59
                  }
                  frame Error {
                  }
                }
              }
            }
            n91 = case shown="True" w40 {
              frame False {
              }
              frame True {
                (unwired) refnum<visa-resource-name> "USB0::0x1313::0x8079::P1000487::INSTR" ("powermeter visa in")
                n92 = call "powermeter-init.vi"("VISA in"="powermeter visa") -> ("Powermeter initialization ok?"=w95:bool, "error out"=w94:errorcluster)  [unwired: 1 out]
                n93 = case shown="No Error" w94 {
                  tunnel: w95 -> [w96 _]
                  frame No Error {
                    "powermeter init" <- w96
                  }
                  frame Error {
                  }
                }
              }
            }
            n94 = case shown="True" w39 {
              frame False {
              }
              frame True {
                n95 = flat-sequence {
                  frame #0 {
                    # "init and set velleman"
                    n96 = call "velleman-init.vi"("Power Control"="velleman-power") -> ("isActive"=→"velleman init":bool, "Power Control 2"=→"velleman-power-status":bool)  [unwired: 3 in, 2 out]
                  }
                  frame #1 {
                    # "init lightsource"
                    n97 = call "lightsource-init.vi"("VISA in"="lightsource-visa") -> ("error out"=w145:errorcluster, "initialized"=w144:bool)  [unwired: 2 in, 1 out]
                    n98 = case shown="No Error" w145 {
                      tunnel: w144 -> [w147 _]
                      frame No Error {
                        n99 = local write "config"(T5."Lightsource" ("config")) -> ()
                        "lightsource" <- w147
                      }
                      frame Error {
                      }
                    }
                  }
                }
              }
            }
          }
          frame #1 {
            # "Set/Get Parameters"
            n100 = stacked-sequence {
              frame #0 {
                # "Set Parameters (LightSource)"
                n101 = flat-sequence {
                  tunnel: [w154] -> w151
                  tunnel: [w153] -> w150
                  tunnel: w151 -> [w181]
                  tunnel: w150 -> [w182]
                  tunnel: [w181] -> w149
                  tunnel: [w180] -> w148
                  tunnel: w149 -> [w196]
                  tunnel: w148 -> [w195]
                  frame #0 {
                    n102 = local read "lightsource"() -> (w152:bool)
                    n103 = case shown="False" w152 {
                      tunnel: [FALSE ("Emission On?") w165] -> w154
                      tunnel: [570 w159] -> w153
                      frame False {
                      }
                      frame True {
                        n104 = local read "lightsource-visa"() -> (w157:refnum<visa-resource-name>)
                        n105 = call "lightsource-write.vi"("VISA in"=w157, "set parameters"=TRUE ("Init NKT?"), "NKT Input"="NKT Input") -> ("NKT Output"=w166:T6, "External Control Cluster"=w176:T35)  [unwired: 3 in, 1 out]
                        "NKT Output" <- w166
                        n106 = feedback #1() -> (w177:T35)  [unwired: 1 in]
                        n107 = feedback-in #1(w176) -> ()
                        n108 = Unbundle By Name(w176) -> ("Emission On/Off external"=w175:bool, "Power/Feedback Mode external"=w174:bool, "Power Level external"=w173:dbl, "Feedback Level external"=w172:dbl)
                        n109 = Not Equal?(x=w176, y=w177) -> (x != y?=w171:T36)
                        n110 = Cluster To Array(cluster=w171) -> (array=w170:bool[])
                        n111 = Or Array Elements(Boolean array=w170) -> (logical OR=w169:bool)
                        n112 = Unbundle By Name(w166) -> ("Emission"=w165:bool, "Short Wavelength (nm)"=w162:dbl, "Long Wavelength (nm)"=w161:dbl)
                        n113 = Bundle By Name(cluster="NKT Input", "Emission"=w175, "Operation Mode"=w174, "Power Level"=w173, "Feedback Level"=w172) -> (w168:T7)
                        n114 = Add(x=w162, y=w161) -> (x+y=w163:dbl)
                        n115 = case shown="True" w169 {
                          tunnel: w168 -> [_ w178]
                          frame False {
                          }
                          frame True {
                            n116 = local write "NKT Input"(w178) -> ()
                          }
                        }
                        n117 = Divide(x=w163, y=2) -> (x/y=w160:dbl)
                        n118 = To Long Integer(number=w160) -> (32bit integer=w159:i32)
                      }
                    }
                  }
                  frame #1 {
                    n119 = local read "powermeter init"() -> (w179:bool)
                    n120 = case shown="False" w179 {
                      tunnel: w182 -> [_ w184]
                      tunnel: [TRUE ("Power Control 2") w187] -> w180
                      frame False {
                      }
                      frame True {
                        n121 = local read "powermeter visa"() -> (w185:refnum<visa-resource-name>)
                        n122 = local read "velleman-power"() -> (w190:bool)
                        n123 = local read "velleman init"() -> (w186:bool)
                        n124 = feedback #2() -> (w193:i32)  [unwired: 1 in]
                        n125 = feedback-in #2(w184) -> ()
                        n126 = Not Equal?(x=w193, y=w184) -> (x != y?=w191:bool)
                        n127 = call "powermeter-main.vi"("Perform Powermeter Auto Zero?"="Perform Auto Zero", "input-wavelength"=w184, "Set Wavelength?"=w191, "VISA in"=w185) -> ("output-wavelength"=→"WL Power (nm)":i32, "power (µW)"=→"Power (µW)":dbl)  [unwired: 1 in, 1 out]
                        n128 = call "velleman-pl.vi"("Power Control"=w190, "isActive"=w186) -> ("Power Control 2"=w187:bool)  [unwired: 5 in, 2 out]
                        n129 = local write "velleman-power-status"(w187) -> ()
                      }
                    }
                  }
                  frame #2 {
                    n130 = local write "Perform Auto Zero"(FALSE ("Perform Auto Zero")) -> ()
                    n131 = And(x=w196, y=w195) -> (x .and. y?=→"laser on":bool)
                  }
                }
              }
              frame #1 {
                # "Set Parameters (Spectrograph)"
                n132 = local read "spectrograph"() -> (w198:bool)
                n133 = case shown="False" w198 {
                  frame False {
                  }
                  frame True {
                    # "Write & Read Shamrock and Detector Settings"
                    n134 = local read "spectrograph-status"() -> (w209:T9)
                    n135 = local read "spectrograph-reset-status"() -> (w205:T11)
                    n136 = feedback #3("spectrograph-input") -> (w215:T10)
                    n137 = feedback-in #3("spectrograph-input") -> ()
                    n138 = Not Equal?(x="spectrograph-input", y=w215) -> (x != y?=w208:T37)
                    n139 = Cluster To Array(cluster=w208) -> (array=w210:bool[])
                    n140 = Implies(1:"spectrograph-reset-input", 2:w205) -> (0:w206:cluster{bool, bool})
                    n141 = Implies(1:w208, 2:w209) -> (0:w207:T38)
                    n142 = Not(x=w206) -> (.not. x?=w202:cluster{bool, bool})
                    "spectrograph-reset-status" <- w202
                    n143 = Not(x=w207) -> (.not. x?=w203:T38)
                    "spectrograph-status" <- w203
                    n144 = call "spectrometer-control.vi"("Value Indicators Input"=w203, "Values changed"=w210, "Spectrograph Reset Input"="spectrograph-reset-input", "Reset Indicators after Init/Loop"=w202, "Spectrograph Value Input"="spectrograph-input") -> ("Reset Indicators"=w213:T11, "Value Indicators Output"=w204:T9, "Spectrograph Value Output"=→"spectrograph-output":T33, "Spectrograph Reset Output"=w214:T29)  [unwired: 2 in]
                    n145 = Cluster To Array(cluster="spectrograph-reset-input") -> (array=w212:bool[])
                    n146 = local write "spectrograph-reset-status"(w213) -> ()
                    n147 = Or Array Elements(Boolean array=w212) -> (logical OR=w211:bool)
                    n148 = local write "spectrograph-status"(w204) -> ()
                    n149 = case shown="False" w211 {
                      tunnel: w214 -> [_ w216]
                      frame False {
                      }
                      frame True {
                        n150 = local write "spectrograph-reset-input"(w216) -> ()
                      }
                    }
                  }
                }
              }
              frame #2 {
                # "Set Parameters (Nanostage)"
                n151 = local read "nanostage init"() -> (w217:bool)
                n152 = case shown="True" w217 {
                  frame False {
                  }
                  frame True {
                    n153 = flat-sequence {
                      tunnel: ["z-axis"] -> w229
                      tunnel: ["y-axis"] -> w228
                      tunnel: ["x-axis"] -> w227
                      tunnel: [w239] -> w223
                      tunnel: w229 -> [w239]
                      tunnel: [w233] -> w224
                      tunnel: w228 -> [w234]
                      tunnel: [w236] -> w225
                      tunnel: w227 -> [w237]
                      tunnel: w225 -> [w247]
                      tunnel: w224 -> [w246]
                      tunnel: w223 -> [w245]
                      tunnel: [w244] -> w222
                      tunnel: [w242] -> w220
                      tunnel: [w241] -> w219
                      tunnel: w222 -> [w249]
                      tunnel: [w249] -> w221
                      tunnel: w220 -> [w248]
                      tunnel: w219 -> [w250]
                      tunnel: w221 -> [w259]
                      tunnel: [w255] -> w218
                      tunnel: [w268] -> w226
                      tunnel: w218 -> [w268]
                      tunnel: w226 -> [w286]
                      frame #0 {
                      }
                      frame #1 {
                        # "check if lef/right and top/bottom\nbuttons should have inverse behaviour"
                        n154 = call "utility-flip-stage.vi"("axis in"=w237, "flip"="switch U/D") -> ("axis out"=w236:dbl)
                        n155 = call "utility-flip-stage.vi"("axis in"=w234, "flip"="switch L/R") -> ("axis out"=w233:dbl)
                      }
                      frame #2 {
                        n156 = local read "All conn. axes"() -> (w242:string[])
                        n157 = Build Array(w247, w246, w245) -> (w240:dbl[])
                        n158 = call "nanostage-set.vi"("setValues"=w240, "Axes to move"=w242) -> ("error out"=w241:errorcluster, "moving"=→"nanostage moving":bool, "getValues"=w244:cluster{"postion":dbl[], "status":bool[]})  [unwired: 1 in]
                      }
                      frame #3 {
                        n159 = case shown="No Error" w250 {
                          selector: w250 -> [_ w254]
                          tunnel: w248 -> [_ w253]
                          frame No Error {
                          }
                          frame Error {
                            n160 = call "nanostage-health.vi"("error in"=w254, "All conn. axes"=w253) -> ("error"=→"stage-error":bool, "error message"=w252:string)
                            n161 = local write "stage error message"(w252) -> ()
                          }
                        }
                      }
                      frame #4 {
                        # "Round Values"
                        n162 = Unbundle By Name(w259) -> ("postion"=w258:dbl[], "status"=w261:bool[])
                        n163 = case shown="True" TRUE {
                          tunnel: w258 -> [w262 w264]
                          tunnel: [w262 w263] -> w257
                          frame False {
                          }
                          frame True {
                            w265 = 10
                            n164 = Multiply(x=w264, y=w265) -> (x*y=w267:dbl[])
                            n165 = Round To Nearest(number=w267) -> (nearest integer value=w266:dbl[])
                            n166 = Divide(x=w266, y=w265) -> (x/y=w263:dbl[])
                          }
                        }
                        n167 = Bundle By Name(cluster=cluster{"postion":dbl[], "status":bool[]} {"postion"=[], "status"=[]} ("input cluster"), "postion"=w257, "status"=w261) -> (w255:cluster{"postion":dbl[], "status":bool[]})
                      }
                      frame #5 {
                        # "show stage position on graph"
                        n168 = local read "laser-freeze"() -> (w269:bool)
                        n169 = local read "switch L/R"() -> (w273:bool)
                        n170 = local read "switch U/D"() -> (w274:bool)
                        n171 = Unbundle By Name(w268) -> ("postion"=w277:dbl[])
                        n172 = Index Array(array=w277, index #1=0 ("index"), index #2=1 ("index")) -> (element #1=w275:dbl, element #2=w272:dbl)
                        n173 = call "utility-flip-stage.vi"("axis in"=w275, "flip"=w274) -> ("axis out"=w271:dbl)
                        n174 = call "utility-flip-stage.vi"("axis in"=w272, "flip"=w273) -> ("axis out"=w270:dbl)
                        n175 = case shown="False" w269 {
                          tunnel: w270 -> [_ w283]
                          tunnel: w271 -> [_ w282]
                          tunnel: [cluster{"y-axis":dbl, "x-axis":dbl} {"y-axis"=0.0, "x-axis"=0.0} w281] -> w276
                          frame False {
                          }
                          frame True {
                            n176 = Bundle("axis out"=w283, "axis out"=w282) -> (w281:cluster{"axis out":dbl, "axis out":dbl})  [unwired: 1 in]
                          }
                        }
                        n177 = stacked-sequence {
                          tunnel: w276 -> [_ w285]
                          frame #0 {
                            n178 = property on="Detected Image" class="IntGraph (strict)"("Active Cursor"=u32 1) -> ()  [unwired: 2 in, 2 out]
                          }
                          frame #1 {
                            n179 = property on="Detected Image" class="IntGraph (strict)"("Cursor.Cursor Position"=w285) -> ()  [unwired: 2 in, 2 out]
                          }
                        }
                      }
                      frame #6 {
                        n180 = property on="z-axis" class="DigNum (strict)"("Increment"="z-stepsize") -> ()  [unwired: 2 in, 2 out]
                        n181 = property on="x-axis" class="DigNum (strict)"("Increment"="xy stepsize") -> ()  [unwired: 2 in, 2 out]
                        n182 = property on="y-axis" class="DigNum (strict)"("Increment"="xy stepsize") -> ()  [unwired: 2 in, 2 out]
                        "getValues" <- w286
                      }
                    }
                  }
                }
              }
              frame #3 {
                n183 = local read "cameras init"() -> (w289:bool)
                n184 = case shown="True" w289 {
                  frame False {
                  }
                  frame True {
                    # "Set Parameters (Camera)"
                    n185 = local read "Detector Select"() -> (w291:u16)
                    n186 = call "detector-andor-xenics-switch.vi"("Detector"=w291) -> ("Manufacturer"=w290:enum16{"Andor", "Xenics", "unknown"})
                    n187 = case shown="\"Andor\"" w290 {
                      frame Default {
                      }
                      frame "Andor" {
                        n188 = stacked-sequence {
                          frame #0 {
                            # "Init Camera"
                            n189 = local read "detector"() -> (w292:bool)
                            n190 = case shown="True" w292 {
                              frame False {
                                n191 = flat-sequence {
                                tunnel: [w295] -> w293
                                tunnel: w293 -> [w316]
                                frame #0 {
                                n192 = local read "Detector Select"() -> (w299:u16)
                                n193 = local read "andor-status-cluster"() -> (w294:T25)
                                n194 = local read "Handle"() -> (w298:cluster{"iDus":i32, "Newton":i32, "Clara":i32})
                                n195 = call "detector-select.vi"("Detector Select"=w299, "Cooling Status"=w294, "Handle"=w298) -> ("Current Detector"=w296:string, "Detector Status"=w297:bool)  [unwired: 1 out]
                                "detector" <- w297
                                n196 = case shown="True" w297 {
                                tunnel: w296 -> [_ w301]
                                tunnel: ["" ("Current Detector") w301] -> w295
                                frame False {
                                }
                                frame True {
                                }
                                }
                                "Current Detector" <- w295
                                }
                                frame #1 {
                                n197 = case shown="\"Clara\"" w316 {
                                tunnel: [w347 T31."Disabled and Grayed Out" ("Disabled") w367 w373] -> w303
                                tunnel: [w347 w358 w367 w374] -> w320
                                tunnel: [1 ("number") w365 1 ("number") w379] -> w319
                                tunnel: [w351 w364 1 ("number") 1 ("number")] -> w313
                                tunnel: [w350 w361 1 ("number") w378] -> w312
                                tunnel: [w348 T31."Enabled" ("Disabled") w367 T31."Disabled and Grayed Out" ("Disabled")] -> w309
                                tunnel: [1.0 ("Data Entry Limits:Maximum") 1024.0 ("Data Entry Limits:Maximum") 1.0 ("Data Entry Limits:Maximum") 256.0 ("Data Entry Limits:Maximum")] -> w308
                                tunnel: [w348 w358 w367 w374] -> w304
                                tunnel: [w347 T31."Enabled" ("Disabled") w367 w373] -> w302
                                frame "InGaAs", "iDus" {
                                w348 = T31."Enabled" ("Disabled")
                                w347 = T31."Disabled and Grayed Out" ("Disabled")
                                # "1 = High Dynamic Range (Conventional CCD register)"
                                # "0 = High Sensitivity (Standard EMCCD gain register)"
                                n198 = call <userlib>:"GetNumberHSSpeeds.vi"("type"=HSSpeed_type_typedef."Conventional Amp", "channel"=0) -> ("error out"=w346:errorcluster, "number"=w351:i32)  [unwired: 1 in, 1 out]
                                n199 = call <userlib>:"GetNumberADChannels.vi"("error in (no error)"=w346) -> ("error out"=w344:errorcluster, "number"=w350:i32)  [unwired: 2 in, 1 out]
                                n200 = call <userlib>:"SetOutputAmplifier.vi"("error in (no error)"=w344, "type"="iDus Type") -> ("DLL error code"=→"DLL error code":u32)  [unwired: 1 out]
                                }
                                frame "Clara" {
                                w358 = T31."Enabled" ("Disabled")
                                n201 = call <userlib>:"GetNumberPreAmpGains.vi"() -> ("error out"=w356:errorcluster, "number"=w365:i32)  [unwired: 3 in, 1 out]
                                n202 = call <userlib>:"GetNumberHSSpeeds.vi"("error in (no error)"=w356, "type"=HSSpeed_type_typedef."Conventional Amp", "channel"=0) -> ("error out"=w355:errorcluster, "number"=w364:i32)  [unwired: 1 out]
                                n203 = call <userlib>:"GetNumberADChannels.vi"("error in (no error)"=w355) -> ("number"=w361:i32)  [unwired: 2 in, 2 out]
                                }
                                frame "", Default {
                                w367 = T31."Disabled and Grayed Out" ("Disabled")
                                }
                                frame "CCD", "Newton" {
                                w374 = T31."Enabled" ("Disabled")
                                w373 = T31."Enabled" ("Disabled")
                                n204 = call <userlib>:"GetNumberPreAmpGains.vi"() -> ("error out"=w372:errorcluster, "number"=w379:i32)  [unwired: 3 in, 1 out]
                                n205 = call <userlib>:"GetNumberADChannels.vi"("error in (no error)"=w372) -> ("number"=w378:i32)  [unwired: 2 in, 2 out]
                                }
                                }
                                n206 = property on="pre-amp 2" class="DigNum (strict)"("DisabledEnum"=w320) -> ()  [unwired: 2 in, 2 out]
                                n207 = property on="HBinning" class="Ring (strict)"("DisabledEnum"=w302) -> ()  [unwired: 2 in, 2 out]
                                n208 = Decrement(x=w319) -> (x-1=w306:i32)
                                n209 = property on="height" class="DigNum (strict)"("DisabledEnum"=w303) -> ()  [unwired: 2 in, 2 out]
                                n210 = Decrement(x=w313) -> (x-1=w307:i32)
                                n211 = Decrement(x=w312) -> (x-1=w305:i32)
                                n212 = property on="Exposure Time" class="DigNum (strict)"("DisabledEnum"=w304) -> ()  [unwired: 2 in, 2 out]
                                n213 = property on="ADchannel" class="DigNum (strict)"("DisabledEnum"=w304) -> ()  [unwired: 2 in, 2 out]
                                n214 = property on="readout mode 2" class="Ring (strict)"("DisabledEnum"=w304) -> ()  [unwired: 2 in, 2 out]
                                n215 = property on="HSSpeed 2" class="DigNum (strict)"("Maximum"=w307) -> ()  [unwired: 2 in, 2 out]
                                n216 = property on="height" class="DigNum (strict)"("Maximum"=w308) -> ()  [unwired: 2 in, 2 out]
                                n217 = property on="pre-amp 2" class="DigNum (strict)"("Maximum"=w306) -> ()  [unwired: 2 in, 2 out]
                                n218 = property on="ADchannel" class="DigNum (strict)"("Maximum"=w305) -> ()  [unwired: 2 in, 2 out]
                                n219 = property on="binning" class="Bool (strict)"("DisabledEnum"=w302) -> ()  [unwired: 2 in, 2 out]
                                n220 = property on="HSSpeed 2" class="DigNum (strict)"("DisabledEnum"=w309) -> ()  [unwired: 2 in, 2 out]
                                n221 = local write "ADchannel"(w305) -> ()
                                n222 = local write "pre-amp 2"(w306) -> ()
                                n223 = local write "HSSpeed 2"(w307) -> ()
                                n224 = case shown="\"Clara\"" w316 {
                                tunnel: [TRUE ("readout mode") FALSE ("readout mode") TRUE ("readout mode") w340] -> w318
                                tunnel: [TRUE ("readout mode") TRUE ("readout mode") TRUE ("readout mode") w340] -> w317
                                tunnel: [TRUE ("readout mode") w330 TRUE ("readout mode") w340] -> w315
                                tunnel: [w323 w331 w336 w342] -> w314
                                tunnel: [FALSE ("readout mode") w330 TRUE ("readout mode") w341] -> w311
                                tunnel: [FALSE ("readout mode") w330 TRUE ("readout mode") w341] -> w310
                                frame "InGaAs", "iDus" {
                                w323 = u16 0 items=["Full Vertical Binning", "Image", "Vertical Binning"] ("readout mode")
                                }
                                frame "Clara" {
                                w331 = u16 1 items=["Full Vertical Binning", "Image", "Vertical Binning"] ("readout mode")
                                w330 = FALSE ("readout mode")
                                n225 = local read "spectrograph-input"() -> (w329:T10)
                                n226 = Bundle By Name(cluster=w329, "Shutter"=u16 0) -> (w328:T10)
                                n227 = local write "spectrograph-input"(w328) -> ()
                                }
                                frame "", Default {
                                w336 = u16 0 items=["Full Vertical Binning", "Image", "Vertical Binning"] ("readout mode")
                                }
                                frame "CCD", "Newton" {
                                w341 = TRUE ("readout mode")
                                w342 = u16 0 items=["Full Vertical Binning", "Image", "Vertical Binning"] ("readout mode")
                                w340 = FALSE ("readout mode")
                                }
                                }
                                n228 = local write "readout mode 2"(w314) -> ()
                                n229 = local write "readout mode"(w318) -> ()
                                n230 = local write "pre-amp 3"(w315) -> ()
                                n231 = local write "ADchannel 2"(w311) -> ()
                                n232 = local write "HSSpeed 3"(w310) -> ()
                                n233 = local write "binning"(w317) -> ()
                                }
                                }
                              }
                              frame True {
                              }
                            }
                          }
                          frame #1 {
                            n234 = stacked-sequence {
                              frame #0 {
                                n235 = local read "exposure time"() -> (w380:bool)
                                n236 = case shown="True" w380 {
                                frame False {
                                n237 = local read "Exposure Time"() -> (w383:dbl)
                                n238 = call "detector-exposuretime-set.vi"("Input Exposure Time"=w383) -> ("exp time ok"=w382:bool, "Output Expsure Time"=w381:sgl)  [unwired: 1 in]
                                "exposure time" <- w382
                                n239 = case shown="False" w382 {
                                tunnel: w381 -> [_ w384]
                                frame False {
                                }
                                frame True {
                                "Exposure Time Read" <- w384
                                }
                                }
                                }
                                frame True {
                                }
                                }
                              }
                            }
                          }
                          frame #2 {
                            n240 = flat-sequence {
                              frame #0 {
                                n241 = local read "binning"() -> (w385:bool)
                                n242 = case shown="True" w385 {
                                frame False {
                                n243 = local read "Current Detector"() -> (w386:string)
                                n244 = local read "HBinning"() -> (w387:u16)
                                n245 = case shown="\"CCD\", \"Clara\", \"Newton\"" w386 {
                                tunnel: [TRUE w391] -> w388
                                tunnel: w387 -> [_ w394]
                                frame "", Default {
                                }
                                frame "CCD", "Clara", "Newton" {
                                n246 = local read "readout mode 2"() -> (w393:u16)
                                n247 = case shown="2" w393 {
                                tunnel: w394 -> [w401 w404 w411]
                                tunnel: [w400 w409 w413] -> w390
                                tunnel: [w399 w408 w412] -> w392
                                frame 0, Default {
                                # "FVB"
                                n248 = call <userlib>:"SetFVBHBin.vi"("bin"=w401) -> ("error out"=w400:errorcluster, "DLL error code"=w399:u32)  [unwired: 1 in]
                                }
                                frame 1 {
                                w407 = 1 ("vstart")
                                # "Image"
                                n249 = call <userlib>:"GetDetector.vi"() -> ("error out"=w406:errorcluster, "ypixels"=w410:i32, "xpixels"=w405:i32)  [unwired: 4 in, 1 out]
                                n250 = Divide(x=w405, y=w404) -> (x/y=w403:dbl)
                                n251 = To Long Integer(number=w403) -> (32bit integer=w402:i32)
                                n252 = call <userlib>:"SetImage.vi"("hbin"=w404, "vbin"=w407, "hstart"=w407, "hend"=w402, "vstart"=w407, "vend"=w410, "error in (no error)"=w406) -> ("DLL error code"=w408:u32, "error out"=w409:errorcluster)  [unwired: 19 in]
                                }
                                frame 2 {
                                n253 = case shown="2, Default" w411 {
                                tunnel: [w416 w424] -> w413
                                tunnel: [w414 w423] -> w412
                                tunnel: w411 -> [_ w422]
                                frame 1 {
                                n254 = call <userlib>:"SetReadMode.vi"("mode"=ReadMode_mode_typedef."Single-Track") -> ("error out"=w416:errorcluster, "DLL error code"=w414:u32)  [unwired: 1 in]
                                n255 = local write "readout mode"(FALSE ("readout mode")) -> ()
                                }
                                frame 2, Default {
                                # "probably unnecessary here to set binning for image\ndelete when in conflict with readout mode"
                                n256 = local read "center"() -> (w433:u16)
                                n257 = local read "height"() -> (w421:u16)
                                n258 = call <userlib>:"SetReadMode.vi"("mode"=ReadMode_mode_typedef."Image") -> ("error out"=w419:errorcluster)  [unwired: 1 in, 1 out]
                                n259 = Divide(x=w421, y=u16 2) -> (x/y=w427:dbl)
                                n260 = To Unsigned Word Integer(number=w427) -> (unsigned 16bit integer=w426:u16)
                                n261 = Subtract(x=w421, y=w426) -> (x-y=w428:u16)
                                n262 = call <userlib>:"GetDetector.vi"("error in (no error)"=w419) -> ("error out"=w431:errorcluster, "xpixels"=w429:i32)  [unwired: 3 in, 2 out]
                                n263 = Add(x=w428, y=w433) -> (x+y=w434:u16)
                                n264 = Subtract(x=w433, y=w426) -> (x-y=w425:u16)
                                n265 = Divide(x=w429, y=w422) -> (x/y=w436:dbl)
                                n266 = local write "readout mode"(TRUE ("readout mode")) -> ()
                                n267 = To Long Integer(number=w436) -> (32bit integer=w430:i32)
                                n268 = call <userlib>:"SetImage.vi"("hbin"=w422, "vbin"=w421, "hstart"=1 ("vstart"), "hend"=w430, "vstart"=w425, "vend"=w434, "error in (no error)"=w431) -> ("DLL error code"=w423:u32, "error out"=w424:errorcluster)  [unwired: 19 in]
                                }
                                }
                                }
                                }
                                n269 = case shown="No Error" w390 {
                                tunnel: w392 -> [w396 _]
                                tunnel: [w395 FALSE] -> w391
                                frame No Error {
                                n270 = Equal?(x=w396, y=20002) -> (x = y?=w395:bool)
                                }
                                frame Error {
                                }
                                }
                                }
                                }
                                "binning" <- w388
                                }
                                frame True {
                                }
                                }
                              }
                            }
                          }
                          frame #3 {
                            n271 = flat-sequence {
                              frame #0 {
                                n272 = local read "ADchannel 2"() -> (w437:bool)
                                n273 = case shown="True" w437 {
                                frame False {
                                n274 = local read "ADchannel"() -> (w446:u8)
                                n275 = flat-sequence {
                                tunnel: w446 -> [w447]
                                tunnel: [w448] -> w445
                                tunnel: [w447] -> w441
                                tunnel: w445 -> [w450]
                                tunnel: [w451] -> w444
                                tunnel: [w449] -> w442
                                tunnel: w441 -> [w449]
                                tunnel: w444 -> [w454]
                                tunnel: [w453] -> w443
                                tunnel: w442 -> [w453]
                                tunnel: w443 -> [w458]
                                tunnel: [w456] -> w440
                                tunnel: [w455] -> w439
                                tunnel: w440 -> [w469]
                                tunnel: w439 -> [w468]
                                tunnel: [w467] -> w438
                                tunnel: w438 -> [w473]
                                frame #0 {
                                n276 = call <userlib>:"SetADChannel.vi"("channel"=w447) -> ("error out"=w448:errorcluster)  [unwired: 1 in, 1 out]
                                }
                                frame #1 {
                                n277 = Unbundle By Name(w450) -> ("status"=w452:bool)
                                n278 = Not(x=w452) -> (.not. x?=w451:bool)
                                }
                                frame #2 {
                                "ADchannel 2" <- w454
                                }
                                frame #3 {
                                # "the following frames\nactually handle HSSpeed"
                                n279 = local read "Current Detector"() -> (w457:string)
                                n280 = case shown="\"\", \"CCD\", \"Newton\", Default" w457 {
                                tunnel: w458 -> [w461 _]
                                tunnel: [w460 0] -> w455
                                tunnel: [w459 errorcluster {"status"=FALSE, "code"=0, "source"="Newton has no HSSpeed"} ("error out")] -> w456
                                frame "Clara", "InGaAs", "iDus" {
                                n281 = call <userlib>:"GetNumberHSSpeeds.vi"("type"=HSSpeed_type_typedef."Conventional Amp", "channel"=w461) -> ("error out"=w459:errorcluster, "number"=w463:i32)  [unwired: 1 in, 1 out]
                                n282 = Decrement(x=w463) -> (x-1=w460:i32)
                                }
                                frame "", "CCD", "Newton", Default {
                                n283 = local write "HSSpeed"(0.0 ("HSSpeed")) -> ()
                                }
                                }
                                }
                                frame #4 {
                                n284 = case shown="No Error" w469 {
                                tunnel: w468 -> [w470 _]
                                tunnel: [w470 0] -> w467
                                frame No Error {
                                w471 = FALSE ("HSSpeed")
                                n285 = local write "HSSpeed 3"(w471) -> ()
                                n286 = local write "pre-amp 3"(w471) -> ()
                                }
                                frame Error {
                                }
                                }
                                }
                                frame #5 {
                                n287 = property on="HSSpeed 2" class="DigNum (strict)"("Maximum"=w473) -> ()  [unwired: 2 in, 2 out]
                                }
                                }
                                }
                                frame True {
                                }
                                }
                              }
                            }
                          }
                          frame #4 {
                            n288 = flat-sequence {
                              frame #0 {
                                n289 = local read "pre-amp 3"() -> (w474:bool)
                                n290 = case shown="True" w474 {
                                frame False {
                                n291 = local read "pre-amp 2"() -> (w479:u8)
                                n292 = flat-sequence {
                                tunnel: w479 -> [w480]
                                tunnel: [w481] -> w478
                                tunnel: [w480] -> w475
                                tunnel: w478 -> [w484]
                                tunnel: [w483] -> w477
                                tunnel: w475 -> [w482]
                                tunnel: w477 -> [w487]
                                tunnel: [w486] -> w476
                                frame #0 {
                                n293 = call <userlib>:"SetPreAmpGain.vi"("index"=w480) -> ("error out"=w481:errorcluster)  [unwired: 1 in, 1 out]
                                }
                                frame #1 {
                                n294 = call <userlib>:"GetPreAmpGain.vi"("error in (no error)"=w484, "index"=w482) -> ("error out"=w483:errorcluster, "gain"=→"pre-amp":sgl)  [unwired: 1 in, 1 out]
                                }
                                frame #2 {
                                n295 = Unbundle By Name(w487) -> ("status"=w488:bool)
                                n296 = Not(x=w488) -> (.not. x?=w486:bool)
                                }
                                }
                                "pre-amp 3" <- w476
                                }
                                frame True {
                                }
                                }
                              }
                            }
                          }
                          frame #5 {
                            n297 = flat-sequence {
                              frame #0 {
                                n298 = local read "HSSpeed 3"() -> (w489:bool)
                                n299 = case shown="True" w489 {
                                frame False {
                                n300 = local read "Current Detector"() -> (w491:string)
                                n301 = case shown="\"\", Default" w491 {
                                tunnel: [TRUE w497] -> w492
                                tunnel: [sgl 0.0 ("speed") w495] -> w490
                                frame "CCD", "Newton" {
                                }
                                frame "", Default {
                                n302 = flat-sequence {
                                tunnel: [HSSpeed_type_typedef."Conventional Amp" ("type")] -> w502
                                tunnel: [w506] -> w501
                                tunnel: [w505] -> w500
                                tunnel: w502 -> [w504]
                                tunnel: [w504] -> w499
                                tunnel: w501 -> [w511]
                                tunnel: [w512] -> w498
                                tunnel: w500 -> [w510]
                                tunnel: w499 -> [w509]
                                tunnel: [w507] -> w496
                                tunnel: w498 -> [w515]
                                tunnel: [w514] -> w497
                                tunnel: w496 -> [w513]
                                tunnel: [w513] -> w495
                                frame #0 {
                                # "@Clara\nconventional=extended NIR"
                                }
                                frame #1 {
                                n303 = local read "HSSpeed 2"() -> (w505:u8)
                                n304 = call <userlib>:"SetHSSpeed.vi"("index"=w505, "type"=w504) -> ("error out"=w506:errorcluster)  [unwired: 2 in, 1 out]
                                }
                                frame #2 {
                                n305 = local read "ADchannel"() -> (w508:u8)
                                n306 = call <userlib>:"GetHSSpeed.vi"("error in (no error)"=w511, "index"=w510, "type"=w509, "channel"=w508) -> ("error out"=w512:errorcluster, "speed"=w507:sgl)  [unwired: 1 in, 1 out]
                                }
                                frame #3 {
                                n307 = Unbundle By Name(w515) -> ("status"=w516:bool)
                                n308 = Not(x=w516) -> (.not. x?=w514:bool)
                                }
                                }
                                }
                                }
                                "HSSpeed 3" <- w492
                                "HSSpeed" <- w490
                                }
                                frame True {
                                }
                                }
                              }
                            }
                          }
                          frame #6 {
                            # "detector-specific tasks"
                            n309 = local read "Current Detector"() -> (w518:string)
                            n310 = local read "Cooling Read"() -> (w517:cluster{"iDus":i32, "Newton":i32, "Clara":i32})
                            n311 = local read "andor-status-cluster"() -> (w519:T25)
                            n312 = case shown="\"Clara\"" w518 {
                              tunnel: w517 -> [w523 w536 _ w565]
                              tunnel: w519 -> [w522 w535 _ w563]
                              frame "InGaAs", "iDus" {
                                n313 = call <userlib>:"GetTemperature.vi"() -> ("error out"=w520:errorcluster, "status"=w521:T19, "temperature"=w524:i32)  [unwired: 4 in, 1 out]
                                n314 = case shown="No Error" w520 {
                                tunnel: w524 -> [w530 _]
                                tunnel: w523 -> [w529 _]
                                tunnel: w522 -> [w528 _]
                                tunnel: w521 -> [w527 _]
                                frame No Error {
                                n315 = Bundle By Name(cluster=w528, "iDus Cooler StatusCode"=w527) -> (w526:T25)
                                n316 = Bundle By Name(cluster=w529, "iDus"=w530) -> (w525:cluster{"iDus":i32, "Newton":i32, "Clara":i32})
                                n317 = local write "andor-status-cluster"(w526) -> ()
                                n318 = local write "Cooling Read"(w525) -> ()
                                }
                                frame Error {
                                }
                                }
                              }
                              frame "Clara" {
                                n319 = local read "readout mode"() -> (w531:bool)
                                n320 = call <userlib>:"GetTemperature.vi"() -> ("status"=w534:T19, "temperature"=w537:i32)  [unwired: 4 in, 2 out]
                                n321 = case shown="True" w531 {
                                frame False {
                                n322 = flat-sequence {
                                tunnel: [w540] -> w538
                                tunnel: w538 -> [w557]
                                frame #0 {
                                n323 = local read "readout mode 2"() -> (w539:u16)
                                n324 = case shown="1, Default" w539 {
                                tunnel: [w541 w547] -> w540
                                frame 0 {
                                n325 = stacked-sequence {
                                seq-local: [w542 _] -> [_ w545]
                                tunnel: [_ w544] -> w541
                                frame #0 {
                                n326 = call <userlib>:"SetReadMode.vi"("mode"=ReadMode_mode_typedef."Full Vertical Binning") -> ("error out"=w542:errorcluster)  [unwired: 1 in, 1 out]
                                }
                                frame #1 {
                                n327 = call <userlib>:"SetFVBHBin.vi"("error in (no error)"=w545, "bin"=1) -> ("error out"=w544:errorcluster)  [unwired: 1 out]
                                }
                                }
                                }
                                frame 1, Default {
                                n328 = stacked-sequence {
                                seq-local: [w548 _] -> [_ w550]
                                tunnel: [_ w551] -> w547
                                frame #0 {
                                n329 = call <userlib>:"SetReadMode.vi"("mode"=ReadMode_mode_typedef."Image") -> ("error out"=w548:errorcluster)  [unwired: 1 in, 1 out]
                                }
                                frame #1 {
                                w553 = 1 ("hbin")
                                n330 = call <userlib>:"GetDetector.vi"("error in (no error)"=w550) -> ("error out"=w552:errorcluster, "ypixels"=w555:i32, "xpixels"=w554:i32)  [unwired: 3 in, 1 out]
                                n331 = call <userlib>:"SetImage.vi"("hbin"=w553, "vbin"=w553, "hstart"=w553, "hend"=w554, "vstart"=w553, "vend"=w555, "error in (no error)"=w552) -> ("error out"=w551:errorcluster)  [unwired: 19 in, 1 out]
                                }
                                }
                                }
                                }
                                }
                                frame #1 {
                                n332 = Unbundle By Name(w557) -> ("status"=w558:bool)
                                n333 = Not(x=w558) -> (.not. x?=w556:bool)
                                n334 = local write "readout mode"(w556) -> ()
                                }
                                }
                                }
                                frame True {
                                }
                                }
                                n335 = Bundle By Name(cluster=w535, "Clara Cooler StatusCode"=w534) -> (w533:T25)
                                n336 = Bundle By Name(cluster=w536, "Clara"=w537) -> (w532:cluster{"iDus":i32, "Newton":i32, "Clara":i32})
                                n337 = local write "andor-status-cluster"(w533) -> ()
                                n338 = local write "Cooling Read"(w532) -> ()
                              }
                              frame "", Default {
                              }
                              frame "CCD", "Newton" {
                                n339 = local read "readout mode 2"() -> (w560:u16)
                                n340 = local read "readout mode"() -> (w559:bool)
                                n341 = call <userlib>:"GetTemperature.vi"() -> ("status"=w562:T19, "temperature"=w566:i32)  [unwired: 4 in, 2 out]
                                n342 = case shown="False" w559 {
                                tunnel: w560 -> [w572 _]
                                frame False {
                                n343 = case shown="1" w572 {
                                tunnel: [w577 w588 w605] -> w571
                                tunnel: [T31."Disabled and Grayed Out" ("Disabled") T31."Disabled and Grayed Out" ("Disabled") T31."Enabled" ("Disabled")] -> w568
                                tunnel: [enum32{"Spectrum", "Image"}."Spectrum" ("Spectra") enum32{"Spectrum", "Image"}."Image" ("Spectra") enum32{"Spectrum", "Image"}."Spectrum" ("Spectra")] -> w567
                                frame 0, Default {
                                (unwired) T39."Spectrograph" ("PLE VIS/UV Panel 2")
                                n344 = stacked-sequence {
                                seq-local: [w578 _ _] -> [_ w581 _]
                                seq-local: [_ w580 _] -> [_ _ w583]
                                tunnel: [_ _ w584] -> w577
                                frame #0 {
                                n345 = call <userlib>:"SetReadMode.vi"("mode"=ReadMode_mode_typedef."Full Vertical Binning") -> ("error out"=w578:errorcluster)  [unwired: 1 in, 1 out]
                                }
                                frame #1 {
                                n346 = call <userlib>:"SetFVBHBin.vi"("error in (no error)"=w581, "bin"=1) -> ("error out"=w580:errorcluster)  [unwired: 1 out]
                                }
                                frame #2 {
                                n347 = call <userlib>:"SetVSSpeed.vi"("error in (no error)"=w583, "index"=1) -> ("error out"=w584:errorcluster)  [unwired: 1 out]
                                }
                                }
                                }
                                frame 1 {
                                n348 = stacked-sequence {
                                seq-local: [w589 _ _ _] -> [_ _ w593 _]
                                seq-local: [_ _ w591 _] -> [_ _ _ w598]
                                tunnel: [_ _ _ w597] -> w588
                                frame #0 {
                                n349 = call <userlib>:"SetReadMode.vi"("mode"=ReadMode_mode_typedef."Image") -> ("error out"=w589:errorcluster)  [unwired: 1 in, 1 out]
                                }
                                frame #1 {
                                }
                                frame #2 {
                                n350 = call <userlib>:"GetNumberVSSpeeds.vi"("error in (no error)"=w593) -> ("error out"=w592:errorcluster, "number"=w594:i32)  [unwired: 2 in, 1 out]
                                n351 = Subtract(x=w594, y=1) -> (x-y=w596:i32)
                                n352 = call <userlib>:"SetVSSpeed.vi"("error in (no error)"=w592, "index"=w596) -> ("error out"=w591:errorcluster)  [unwired: 1 out]
                                }
                                frame #3 {
                                w600 = 1 ("hbin")
                                n353 = call <userlib>:"GetDetector.vi"("error in (no error)"=w598) -> ("error out"=w599:errorcluster, "ypixels"=w602:i32, "xpixels"=w601:i32)  [unwired: 3 in, 1 out]
                                n354 = call <userlib>:"SetImage.vi"("hbin"=w600, "vbin"=w600, "hstart"=w600, "hend"=w601, "vstart"=w600, "vend"=w602, "error in (no error)"=w599) -> ("error out"=w597:errorcluster)  [unwired: 19 in, 1 out]
                                }
                                }
                                }
                                frame 2 {
                                (unwired) T39."Spectrograph" ("PLE VIS/UV Panel 2")
                                # "single track"
                                n355 = stacked-sequence {
                                seq-local: [w606 _] -> [_ w610]
                                tunnel: [_ w611] -> w605
                                frame #0 {
                                n356 = call <userlib>:"SetReadMode.vi"("mode"=ReadMode_mode_typedef."Single-Track") -> ("error out"=w606:errorcluster)  [unwired: 1 in, 1 out]
                                }
                                frame #1 {
                                n357 = local read "center"() -> (w608:u16)
                                n358 = local read "height"() -> (w609:u16)
                                n359 = call <userlib>:"SetSingleTrack.vi"("error in (no error)"=w610, "height"=w609, "centre"=w608) -> ("error out"=w611:errorcluster)  [unwired: 1 in, 1 out]
                                }
                                }
                                }
                                }
                                n360 = Unbundle By Name(w571) -> ("status"=w570:bool)
                                n361 = Not(x=w570) -> (.not. x?=w569:bool)
                                "readout mode" <- w569
                                n362 = case shown="True" w569 {
                                tunnel: w568 -> [_ w574]
                                tunnel: w567 -> [_ w573]
                                frame False {
                                }
                                frame True {
                                (unwired) FALSE
                                n363 = property on="height" class="DigNum (strict)"("DisabledEnum"=w574) -> ()  [unwired: 2 in, 2 out]
                                n364 = local write "Spectra"(w573) -> ()
                                }
                                }
                                }
                                frame True {
                                }
                                }
                                n365 = Bundle By Name(cluster=w563, "Newton Cooler StatusCode"=w562) -> (w561:T25)
                                n366 = Bundle By Name(cluster=w565, "Newton"=w566) -> (w564:cluster{"iDus":i32, "Newton":i32, "Clara":i32})
                                n367 = local write "andor-status-cluster"(w561) -> ()
                                n368 = local write "Cooling Read"(w564) -> ()
                              }
                            }
                          }
                          frame #7 {
                            # "Get Parameters: pixel scaling (Camera: x-Axis) Wavelength vs Image magnification"
                            n369 = local read "pixel scaling"() -> (w612:bool)
                            n370 = case shown="False" w612 {
                              frame False {
                                n371 = flat-sequence {
                                frame #0 {
                                n372 = local read "Current Detector"() -> (w627:string)
                                n373 = local read "HBinning"() -> (w618:u16)
                                n374 = call <userlib>:"GetDetector.vi"() -> ("ypixels"=w624:i32, "xpixels"=w628:i32)  [unwired: 4 in, 2 out]
                                n375 = call <userlib>:"GetPixelSize.vi"() -> ("ysize"=w625:sgl, "xsize"=w629:sgl)  [unwired: 4 in, 2 out]
                                n376 = case shown="\"CCD\", \"InGaAs\", \"Newton\", \"iDus\", Default" w627 {
                                tunnel: [w633 w709] -> w621
                                tunnel: [w631 w704] -> w622
                                tunnel: [w632 w710] -> w623
                                tunnel: [w642 "nm"] -> w620
                                tunnel: w629 -> [w643 w721]
                                tunnel: w628 -> [w631 w706]
                                tunnel: w618 -> [_ w719]
                                tunnel: [w641 w716] -> w615
                                tunnel: w625 -> [w640 w703]
                                tunnel: [w639 w717] -> w614
                                tunnel: w624 -> [w630 w714]
                                tunnel: [w630 w715] -> w613
                                tunnel: [w634 w713] -> w617
                                frame "Clara" {
                                w636 = 0 ("xpixels")
                                n377 = case shown="False" "laser-offset" {
                                tunnel: w636 -> [w646 w651]
                                tunnel: [w646 w652] -> w637
                                tunnel: w636 -> [w645 w650]
                                tunnel: [w645 w653] -> w635
                                frame False {
                                }
                                frame True {
                                n378 = local read "image-laser-position"() -> (w649:T15)
                                n379 = Unbundle By Name(w649) -> ("laser-x-position"=w647:u16, "laser-y-position"=w648:u16)
                                n380 = Subtract(x=w651, y=w647) -> (x-y=w652:i32)
                                n381 = Subtract(x=w650, y=w648) -> (x-y=w653:i32)
                                }
                                }
                                n382 = case shown="False" "magnification" {
                                tunnel: w643 -> [_ w664]
                                tunnel: [sgl 1.0 ("xsize") w669] -> w632
                                tunnel: [sgl 0.0 ("x*y") w672] -> w633
                                tunnel: ["px" "µm"] -> w642
                                tunnel: [sgl 0.0 ("x*y") w671] -> w641
                                tunnel: [sgl 1.0 ("ysize") w667] -> w639
                                tunnel: w640 -> [_ w673]
                                tunnel: w637 -> [_ w666]
                                tunnel: w635 -> [_ w665]
                                frame False {
                                }
                                frame True {
                                n383 = local read "nanostage init"() -> (w662:bool)
                                n384 = Not(x="laser-freeze") -> (.not. x?=w659:bool)
                                n385 = Divide(x=w664, y="magnification") -> (x/y=w670:dbl)
                                n386 = Divide(x=w673, y="magnification") -> (x/y=w668:dbl)
                                n387 = And(x=w659, y=w662) -> (x .and. y?=w661:bool)
                                n388 = case shown="True" w661 {
                                tunnel: [w675 w693] -> w672
                                tunnel: [w676 w694] -> w671
                                tunnel: w670 -> [w680 w690]
                                tunnel: [w680 w686] -> w669
                                tunnel: w668 -> [w679 w687]
                                tunnel: [w679 w681] -> w667
                                tunnel: w666 -> [w678 w685]
                                tunnel: w665 -> [w677 w683]
                                frame False {
                                n389 = Multiply(x=w680, y=w678) -> (x*y=w675:dbl)
                                n390 = Multiply(x=w679, y=w677) -> (x*y=w676:dbl)
                                }
                                frame True {
                                n391 = local read "switch L/R"() -> (w691:bool)
                                n392 = local read "switch U/D"() -> (w688:bool)
                                n393 = case shown="True" w691 {
                                tunnel: w690 -> [w698 w700]
                                tunnel: [w699 w700] -> w686
                                frame False {
                                n394 = Negate(x=w698) -> (-x=w699:dbl)
                                }
                                frame True {
                                }
                                }
                                n395 = case shown="False" w688 {
                                tunnel: [w695 w697] -> w681
                                tunnel: w687 -> [w695 w696]
                                frame False {
                                }
                                frame True {
                                n396 = Negate(x=w696) -> (-x=w697:dbl)
                                }
                                }
                                n397 = Multiply(x=w686, y=w685) -> (x*y=w684:dbl)
                                n398 = local read "y-axis"() -> (w689:dbl)
                                n399 = local read "x-axis"() -> (w692:dbl)
                                n400 = Multiply(x=w681, y=w683) -> (x*y=w682:dbl)
                                n401 = Add(x=w684, y=w689) -> (x+y=w693:dbl)
                                n402 = Add(x=w682, y=w692) -> (x+y=w694:dbl)
                                }
                                }
                                }
                                }
                                n403 = call "camera-build-pixel-array.vi"("size"=w631, "step"=w632, "start"=w633) -> ("construction"=w634:dbl[])
                                }
                                frame "CCD", "InGaAs", "Newton", "iDus", Default {
                                n404 = local read "readout mode 2"() -> (w718:u16)
                                n405 = case shown="False" FALSE {
                                tunnel: w703 -> [_ w726]
                                tunnel: [sgl 1.0 ("ysize") w726] -> w702
                                frame False {
                                # "y-pixel-size to 1 for all detector"
                                }
                                frame True {
                                }
                                }
                                n406 = case shown="0, Default" w718 {
                                tunnel: w702 -> [w731 w734 w737]
                                tunnel: w714 -> [w730 w732 _]
                                tunnel: [w729 w734 w738] -> w717
                                tunnel: [sgl 0.0 ("x*y") sgl 0.0 ("x*y") sgl 0.0 ("x*y")] -> w716
                                tunnel: [u16 1 ("x*y") w732 w735] -> w715
                                frame 0, Default {
                                # "deltay"
                                # "firsty"
                                # "sizey"
                                # "FVB"
                                n407 = Multiply(x=w731, y=w730) -> (x*y=w729:sgl)
                                }
                                frame 1 {
                                # "image mode"
                                }
                                frame 2 {
                                # "vert binning"
                                n408 = local read "height"() -> (w735:u16)
                                n409 = Multiply(x=w737, y=w735) -> (x*y=w738:sgl)
                                }
                                }
                                n410 = Multiply(x=w721, y=w719) -> (x*y=w720:sgl)
                                n411 = Divide(x=w706, y=w719) -> (x/y=w705:dbl)
                                n412 = Round Toward +Infinity(x=w705) -> (ceil(x): smallest int >= x=w707:dbl)
                                n413 = To Unsigned Word Integer(number=w707) -> (unsigned 16bit integer=w704:u16)
                                n414 = call "output-wavelength.vi"("set pixel width"=w720, "Set Number Pixels"=w704) -> ("wavelength array"=w713:sgl[], "Wavelength Last Pixel"=w708:sgl, "Wavelength First Pixel"=w709:sgl)  [unwired: 4 in, 2 out]
                                n415 = Subtract(x=w708, y=w709) -> (x-y=w722:sgl)
                                n416 = Decrement(x=w704) -> (x-1=w723:u16)
                                n417 = Divide(x=w722, y=w723) -> (x/y=w710:sgl)
                                n418 = local read "wavelength-limits"() -> (w711:T8)
                                n419 = Bundle By Name(cluster=w711, "wl-start"=w709, "wl-step"=w710, "wl-end"=w708) -> (→"wavelength-limits":T8)
                                }
                                }
                                "x-scale array" <- w617
                                n420 = local read "Pixel Scaling"() -> (w626:T16)
                                n421 = Bundle By Name(cluster=w626, "deltax"=w623, "deltay"=w614, "size x"=w622, "size y"=w613, "first x"=w621, "first y"=w615, "unit"=w620) -> (→"Pixel Scaling":T16)
                                n422 = call "camera-build-pixel-array.vi"("size"=w613, "step"=w614, "start"=w615) -> ("construction"=→"y-scale array":dbl[])
                                }
                                frame #1 {
                                w739 = TRUE ("pixel scaling")
                                n423 = local write "refresh display"(w739) -> ()
                                "pixel scaling" <- w739
                                }
                                }
                              }
                              frame True {
                              }
                            }
                          }
                        }
                      }
                    }
                  }
                }
              }
              frame #4 {
                # "Set/Get Parameters XEVA"
                n424 = local read "xeva init"() -> (w740:bool)
                n425 = case shown="False" w740 {
                  frame False {
                  }
                  frame True {
                    n426 = local read "Detector Select"() -> (w741:u16)
                    n427 = call "detector-andor-xenics-switch.vi"("Detector"=w741) -> ("Manufacturer"=w742:enum16{"Andor", "Xenics", "unknown"})
                    n428 = case shown="\"Xenics\"" w742 {
                      frame Default {
                      }
                      frame "Xenics" {
                        w746 = u16 1 items=["Full Vertical Binning", "Image", "Vertical Binning"] ("readout mode 2")
                        # "set exposure time"
                        n429 = local read "xeva-camref"() -> (w749:T23)
                        n430 = local read "Exposure Time"() -> (w752:dbl)
                        n431 = local read "exposure time"() -> (w753:bool)
                        n432 = local write "detector"(TRUE ("detector")) -> ()
                        n433 = local write "readout mode"(TRUE ("readout mode")) -> ()
                        n434 = local write "detector"(TRUE ("detector")) -> ()
                        n435 = local write "readout mode 2"(w746) -> ()
                        n436 = case shown="False" w753 {
                          tunnel: w749 -> [w767 _]
                          tunnel: w752 -> [w765 _]
                          tunnel: [w764 errorcluster {"status"=FALSE, "code"=0, "source"=""} ("error out")] -> w751
                          frame False {
                            n437 = call "xeva-setTime.vi"("xeva-time"=w765, "xeva-camref"=w767) -> ("error out"=w764:errorcluster, "xeva-time-ok"=w766:bool)  [unwired: 2 in]
                            n438 = local write "exposure time"(w766) -> ()
                          }
                          frame True {
                          }
                        }
                        n439 = call "xeva-getParam.vi"("error in (no error)"=w751, "xeva-camref"=w749) -> ("error out"=w756:errorcluster, "xeva-parameters"=w747:T13)
                        "xeva-parameters" <- w747
                        n440 = local read "pixel scaling"() -> (w750:bool)
                        n441 = local read "xenics-status-cluster"() -> (w754:T24)
                        n442 = Unbundle By Name(w747) -> ("time"=w743:dbl)
                        n443 = case shown="True" w750 {
                          tunnel: w747 -> [w763 _]
                          frame False {
                            # "set pixel dimensions"
                            n444 = Unbundle By Name(w763) -> ("width"=w762:u32, "height"=w759:u32)
                            n445 = Bundle By Name(cluster=T16 {"first x"=0.0, "size x"=0, "deltax"=1.0, "first y"=0.0, "size y"=0, "deltay"=1.0, "unit"=""} ("Pixel Scaling"), "size x"=w762, "size y"=w759, "unit"="px") -> (w760:T16)
                            n446 = local write "Pixel Scaling"(w760) -> ()
                            n447 = local write "pixel scaling"(TRUE ("pixel scaling")) -> ()
                          }
                          frame True {
                          }
                        }
                        n448 = local write "Exposure Time Read"(w743) -> ()
                        n449 = call "xeva-collect-paramter-error.vi"("error"=w756, "xenics-status-cluster-in"=w754) -> ("xenics-status-cluster-out"=w755:T24)  [unwired: 1 in]
                        n450 = local write "xenics-status-cluster"(w755) -> ()
                      }
                    }
                  }
                }
              }
              frame #5 {
                # "set Gui Controls"
                n451 = local read "xenics-status-cluster"() -> (w777:T24)
                n452 = local read "andor-status-cluster"() -> (w769:T25)
                n453 = feedback-in #4(w777) -> ()
                n454 = feedback #4() -> (w778:T24)  [unwired: 1 in]
                n455 = feedback #5() -> (w770:T25)  [unwired: 1 in]
                n456 = feedback-in #5(w769) -> ()
                n457 = Not Equal?(x=w769, y=w770) -> (x != y?=w775:T40)
                n458 = Not Equal?(x=w777, y=w778) -> (x != y?=w776:T41)
                n459 = Cluster To Array(cluster=w776) -> (array=w774:bool[])
                n460 = Cluster To Array(cluster=w775) -> (array=w773:bool[])
                n461 = Build Array(w774, w773) -> (w772:bool[][])
                n462 = Or Array Elements(Boolean array=w772) -> (logical OR=w771:bool)
                n463 = case shown="True" w771 {
                  tunnel: w769 -> [_ w785]
                  tunnel: w777 -> [_ w784]
                  frame False {
                  }
                  frame True {
                    n464 = call "gui-camera-status-converter.vi"("xenics-status-cluster"=w784, "andor-status-cluster"=w785) -> ("general-camera-status"=w783:T21)
                    "general-camera-status" <- w783
                    n465 = call "gui-camera-disabled-array.vi"("general-camera-status"=w783) -> ("enabled detectors"=w781:i32[], "disabled detectors"=w780:i32[])
                    n466 = property on="Detector Select" class="Ring (strict)"("Disabled Items []"=w780) -> ()  [unwired: 2 in, 2 out]
                    n467 = local read "Detector Select"() -> (w782:u16)
                    n468 = call "gui-is-detector-possible.vi"("disabled detectors"=w780, "detector-in"=w782, "enabled detectors"=w781) -> ("detector-out"=w779:u16)
                    n469 = local write "Detector Select"(w779) -> ()
                  }
                }
              }
            }
          }
          frame #2 {
            # "Close All Devices"
            n470 = flat-sequence {
              frame #0 {
                n471 = local read "init spectrograph"() -> (w796:bool)
                n472 = local read "spectrograph"() -> (w797:bool)
                n473 = local read "init cameras"() -> (w789:bool)
                n474 = local read "xeva init"() -> (w787:bool)
                n475 = local read "cameras init"() -> (w791:bool)
                n476 = local read "init xeva"() -> (w788:bool)
                n477 = Exclusive Or(1:w787, 2:w788) -> (0:w786:bool)
                n478 = Exclusive Or(1:w797, 2:w796) -> (0:w795:bool)
                n479 = Exclusive Or(1:w789, 2:w791) -> (0:w790:bool)
                n480 = case shown="True" w786 {
                  frame False {
                  }
                  frame True {
                    n481 = local read "xeva-camref"() -> (w799:T23)
                    n482 = call "xeva-close.vi"("xeva-camref"=w799) -> ("error out"=w798:errorcluster)  [unwired: 4 in]
                    n483 = case shown="No Error" w798 {
                      frame No Error {
                        n484 = local write "xenics-status-cluster"(T24 {"Xeva-init"=FALSE, "xeva-cooling"=FALSE, "xeva-parameters"=FALSE, "xeva-error"=""} ("xenics-status-cluster")) -> ()
                        n485 = local write "xeva init"(FALSE ("xeva init")) -> ()
                      }
                      frame Error {
                      }
                    }
                  }
                }
                n486 = case shown="False" w795 {
                  frame False {
                  }
                  frame True {
                    n487 = flat-sequence {
                      frame #0 {
                        w816 = u16 0 items=["Close", "Open"] ("Shutter")
                        n488 = call <userlib>:"shamrock_shutterAction.vi"("Mode"=w816, "SetShutter"=TRUE, "Device No"=0) -> ()  [unwired: 1 out]
                      }
                      frame #1 {
                        n489 = local write "spectrograph"(FALSE ("spectrograph")) -> ()
                      }
                    }
                  }
                }
                n490 = case shown="False" w790 {
                  frame False {
                  }
                  frame True {
                    # "Switch off Coolers and Close Detectors"
                    n491 = flat-sequence {
                      frame #0 {
                        # "Switch off Cooling"
                        n492 = stacked-sequence {
                          tunnel: [w832 _ _] -> w827
                          tunnel: [_ w849 _] -> w824
                          tunnel: [_ _ w866] -> w823
                          frame #0 {
                            n493 = local read "andor-status-cluster"() -> (w831:T25)
                            n494 = Unbundle By Name(w831) -> ("iDus Init"=w829:bool, "iDus Cooling"=w830:bool)
                            n495 = And(x=w829, y=w830) -> (x .and. y?=w828:bool)
                            n496 = case shown="True" w828 {
                              tunnel: [FALSE w835] -> w832
                              frame False {
                              }
                              frame True {
                                n497 = local read "Handle"() -> (w834:cluster{"iDus":i32, "Newton":i32, "Clara":i32})
                                n498 = Unbundle By Name(w834) -> ("iDus"=w842:i32)
                                n499 = call <userlib>:"SetCurrentCamera.vi"("cameraHandle"=w842) -> ("error out"=w843:errorcluster)  [unwired: 1 in, 1 out]
                                n500 = call <userlib>:"CoolerOFF.vi"("error in (no error)"=w843) -> ("error out"=w844:errorcluster, "DLL error code"=w839:u32)  [unwired: 1 in]
                                n501 = Unbundle By Name(w844) -> ("status"=w841:bool)
                                n502 = Equal?(x=w839, y=u32 20202 ("DLL error code")) -> (x = y?=w837:bool)
                                n503 = Not(x=w841) -> (.not. x?=w838:bool)
                                n504 = And(x=w837, y=w838) -> (x .and. y?=w836:bool)
                                n505 = Not(x=w836) -> (.not. x?=w835:bool)
                              }
                            }
                          }
                          frame #1 {
                            n506 = local read "andor-status-cluster"() -> (w848:T25)
                            n507 = Unbundle By Name(w848) -> ("Newton Cooling"=w847:bool, "Newton Init"=w846:bool)
                            n508 = And(x=w847, y=w846) -> (x .and. y?=w845:bool)
                            n509 = case shown="True" w845 {
                              tunnel: [FALSE w852] -> w849
                              frame False {
                              }
                              frame True {
                                n510 = local read "Handle"() -> (w851:cluster{"iDus":i32, "Newton":i32, "Clara":i32})
                                n511 = Unbundle By Name(w851) -> ("Newton"=w859:i32)
                                n512 = call <userlib>:"SetCurrentCamera.vi"("cameraHandle"=w859) -> ("error out"=w860:errorcluster)  [unwired: 1 in, 1 out]
                                n513 = call <userlib>:"CoolerOFF.vi"("error in (no error)"=w860) -> ("error out"=w861:errorcluster, "DLL error code"=w856:u32)  [unwired: 1 in]
                                n514 = Unbundle By Name(w861) -> ("status"=w858:bool)
                                n515 = Equal?(x=w856, y=u32 20202 ("DLL error code")) -> (x = y?=w854:bool)
                                n516 = Not(x=w858) -> (.not. x?=w855:bool)
                                n517 = And(x=w854, y=w855) -> (x .and. y?=w853:bool)
                                n518 = Not(x=w853) -> (.not. x?=w852:bool)
                              }
                            }
                          }
                          frame #2 {
                            n519 = local read "andor-status-cluster"() -> (w865:T25)
                            n520 = Unbundle By Name(w865) -> ("Clara Init"=w863:bool, "Clara Cooling"=w864:bool)
                            n521 = And(x=w863, y=w864) -> (x .and. y?=w862:bool)
                            n522 = case shown="True" w862 {
                              tunnel: [FALSE w869] -> w866
                              frame False {
                              }
                              frame True {
                                n523 = local read "Handle"() -> (w868:cluster{"iDus":i32, "Newton":i32, "Clara":i32})
                                n524 = Unbundle By Name(w868) -> ("Clara"=w876:i32)
                                n525 = call <userlib>:"SetCurrentCamera.vi"("cameraHandle"=w876) -> ("error out"=w877:errorcluster)  [unwired: 1 in, 1 out]
                                n526 = call <userlib>:"CoolerOFF.vi"("error in (no error)"=w877) -> ("error out"=w878:errorcluster, "DLL error code"=w873:u32)  [unwired: 1 in]
                                n527 = Unbundle By Name(w878) -> ("status"=w875:bool)
                                n528 = Equal?(x=w873, y=u32 20202 ("DLL error code")) -> (x = y?=w871:bool)
                                n529 = Not(x=w875) -> (.not. x?=w872:bool)
                                n530 = And(x=w871, y=w872) -> (x .and. y?=w870:bool)
                                n531 = Not(x=w870) -> (.not. x?=w869:bool)
                              }
                            }
                          }
                        }
                        n532 = local read "andor-status-cluster"() -> (w825:T25)
                        n533 = Bundle By Name(cluster=w825, "iDus Cooling"=w827, "Newton Cooling"=w824, "Clara Init"=w823) -> (w826:T25)
                        n534 = local write "andor-status-cluster"(w826) -> ()
                      }
                      frame #1 {
                        # "Check Temperature Status and Close Inactive Detector"
                        n535 = node-c288() -> (w880:T26)  [unwired: 10 in]
                        n536 = timed-loop {
                          timing: w880 -> [_]
                          timing-out: [_] -> w879
                          stop <- w882 continue-if-true
                          # "\"init\" could be\n mis-understandable"
                          n537 = node-c288() -> (w911:errorcluster)  [unwired: 1 in]
                          n538 = local read "andor-status-cluster"() -> (w890:T25)
                          n539 = local read "Handle"() -> (w896:cluster{"iDus":i32, "Newton":i32, "Clara":i32})
                          n540 = Unbundle By Name(w890) -> ("iDus Init"=w889:bool, "Newton Init"=w888:bool, "Clara Init"=w887:bool)
                          n541 = Unbundle By Name(w896) -> ("iDus"=w895:i32, "Newton"=w894:i32, "Clara"=w893:i32)
                          n542 = case shown="False" w889 {
                            tunnel: [w931 w938] -> w912
                            tunnel: w911 -> [w931 w937]
                            tunnel: [0 ("temperature") w936] -> w907
                            tunnel: [Error_Code_Enum_typedef."DRV_SUCCESS" ("status") w935] -> w897
                            tunnel: w895 -> [_ w934]
                            frame False {
                            }
                            frame True {
                              n543 = call <userlib>:"SetCurrentCamera.vi"("error in (no error)"=w937, "cameraHandle"=w934) -> ("error out"=w939:errorcluster)  [unwired: 1 out]
                              n544 = call <userlib>:"GetTemperature.vi"("error in (no error)"=w939) -> ("error out"=w938:errorcluster, "status"=w935:T19, "temperature"=w936:i32)  [unwired: 3 in, 1 out]
                            }
                          }
                          n545 = case shown="False" w888 {
                            tunnel: w912 -> [w924 w930]
                            tunnel: [0 ("temperature") w928] -> w908
                            tunnel: [w924 w927] -> w902
                            tunnel: [Error_Code_Enum_typedef."DRV_SUCCESS" ("status") w926] -> w898
                            tunnel: w894 -> [_ w925]
                            frame False {
                            }
                            frame True {
                              n546 = call <userlib>:"SetCurrentCamera.vi"("error in (no error)"=w930, "cameraHandle"=w925) -> ("error out"=w929:errorcluster)  [unwired: 1 out]
                              n547 = call <userlib>:"GetTemperature.vi"("error in (no error)"=w929) -> ("error out"=w927:errorcluster, "status"=w926:T19, "temperature"=w928:i32)  [unwired: 3 in, 1 out]
                            }
                          }
                          n548 = case shown="True" w887 {
                            tunnel: [w915 w921] -> w903
                            tunnel: w902 -> [w915 w920]
                            tunnel: [0 ("temperature") w918] -> w901
                            tunnel: [Error_Code_Enum_typedef."DRV_SUCCESS" ("status") w917] -> w899
                            tunnel: w893 -> [_ w916]
                            frame False {
                            }
                            frame True {
                              n549 = call <userlib>:"SetCurrentCamera.vi"("error in (no error)"=w920, "cameraHandle"=w916) -> ("error out"=w919:errorcluster)  [unwired: 1 out]
                              n550 = call <userlib>:"GetTemperature.vi"("error in (no error)"=w919) -> ("error out"=w921:errorcluster, "status"=w917:T19, "temperature"=w918:i32)  [unwired: 3 in, 1 out]
                            }
                          }
                          n551 = Less Than 0?(x=w908) -> (x < 0?=w900:bool)
                          n552 = Less Than 0?(x=w907) -> (x < 0?=w891:bool)
                          n553 = Less Than 0?(x=w901) -> (x < 0?=w892:bool)
                          n554 = local read "Cooling Read"() -> (w910:cluster{"iDus":i32, "Newton":i32, "Clara":i32})
                          n555 = local read "andor-status-cluster"() -> (w906:T25)
                          n556 = Bundle By Name(cluster=w910, "iDus"=w907, "Newton"=w908, "Clara"=w901) -> (w909:cluster{"iDus":i32, "Newton":i32, "Clara":i32})
                          n557 = Bundle By Name(cluster=w906, "iDus Init"=w891, "Newton Init"=w900, "Clara Init"=w892, "iDus Cooler StatusCode"=w897, "Newton Cooler StatusCode"=w898, "Clara Cooler StatusCode"=w899) -> (w905:T25)
                          n558 = Build Array(w892, w900, w891) -> (w904:bool[])
                          n559 = Or Array Elements(Boolean array=w904) -> (logical OR=w885:bool)
                          n560 = local read "init cameras"() -> (w886:bool)
                          n561 = local write "Cooling Read"(w909) -> ()
                          n562 = local write "andor-status-cluster"(w905) -> ()
                          n563 = Not(x=w886) -> (.not. x?=w884:bool)
                          n564 = Build Array(w885, w884, "detector-warmup") -> (w883:bool[])
                          n565 = And Array Elements(Boolean array=w883) -> (logical AND=w882:bool)
                          n566 = node-c288(w903) -> ()  [unwired: 1 out]
                        }
                        n567 = node-c288(w879) -> ()  [unwired: 1 out]
                      }
                      frame #2 {
                        # "error checking disabled"
                        n568 = local read "andor-status-cluster"() -> (w951:T25)
                        n569 = Bundle By Name(cluster=w951, "iDus Parameters"=FALSE, "Newton Parameters"=FALSE, "Clara Parameters"=FALSE) -> (w950:T25)
                        n570 = local write "andor-status-cluster"(w950) -> ()
                        n571 = local write "cameras init"(FALSE ("detectors")) -> ()
                      }
                    }
                  }
                }
                n572 = local read "init lightsource"() -> (w793:bool)
                n573 = local read "lightsource"() -> (w792:bool)
                n574 = Exclusive Or(1:w792, 2:w793) -> (0:w794:bool)
                n575 = case shown="False" w794 {
                  frame False {
                  }
                  frame True {
                    n576 = local read "lightsource-visa"() -> (w820:refnum<visa-resource-name>)
                    n577 = local read "NKT Input"() -> (w822:T7)
                    n578 = local read "velleman init"() -> (w821:bool)
                    n579 = call "lightsource-emission-kill.vi"("NKT Input"=w822, "VISA in"=w820) -> ("lightsource init"=w818:bool)
                    n580 = call "velleman-close.vi"("isActive"=w821) -> ("error"=w819:bool)
                    n581 = local write "lightsource"(w818) -> ()
                    n582 = local write "velleman init"(w819) -> ()
                  }
                }
                n583 = flat-sequence {
                  frame #0 {
                    n584 = local read "init powermeter"() -> (w802:bool)
                    n585 = local read "powermeter init"() -> (w803:bool)
                    n586 = Exclusive Or(1:w803, 2:w802) -> (0:w804:bool)
                    n587 = case shown="False" w804 {
                      frame False {
                      }
                      frame True {
                        n588 = local read "powermeter visa"() -> (w806:refnum<visa-resource-name>)
                        n589 = call "powermeter-close.vi"("VISA resource name"=w806) -> ("error out"=w805:errorcluster)  [unwired: 2 in]
                        n590 = case shown="No Error" w805 {
                          frame No Error {
                            n591 = local write "powermeter init"(FALSE ("powermeter")) -> ()
                          }
                          frame Error {
                          }
                        }
                      }
                    }
                  }
                }
                n592 = flat-sequence {
                  frame #0 {
                    n593 = local read "init nanostage"() -> (w810:bool)
                    n594 = local read "nanostage init"() -> (w809:bool)
                    n595 = Exclusive Or(1:w809, 2:w810) -> (0:w808:bool)
                    n596 = case shown="False" w808 {
                      frame False {
                      }
                      frame True {
                        n597 = local read "All conn. axes"() -> (w811:string[])
                        n598 = call "nanostage-close.vi"("All conn. axes"=w811) -> ("error out"=w812:errorcluster)
                        n599 = case shown="No Error" w812 {
                          frame No Error {
                            # "do nothing"
                          }
                          frame Error {
                          }
                        }
                        n600 = local write "nanostage init"(FALSE ("nanostage")) -> ()
                      }
                    }
                  }
                }
              }
              frame #1 {
                # "shutdown andor system only if \nnothing from andor is active"
                n601 = local read "spectrograph"() -> (w958:bool)
                n602 = local read "cameras init"() -> (w957:bool)
                n603 = Build Array(w958, w957) -> (w956:bool[])
                n604 = Equal?(x=FALSE, y=w956) -> (x = y?=w954:bool[])
                n605 = And Array Elements(Boolean array=w954) -> (logical AND=w953:bool)
                n606 = case shown="True" w953 {
                  frame False {
                  }
                  frame True {
                    n607 = local read "ANDOR init"() -> (w959:bool)
                    n608 = case shown="True" w959 {
                      frame False {
                      }
                      frame True {
                        n609 = flat-sequence {
                          tunnel: [TRUE] -> w960
                          tunnel: [TRUE] -> w961
                          frame #0 {
                            n610 = call <userlib>:"shamrock_close.vi"() -> ()  [unwired: 1 out]
                          }
                          frame #1 {
                            n611 = call <userlib>:"ShutDown.vi"() -> ("error out"=w967:errorcluster)  [unwired: 2 in, 1 out]
                            n612 = case shown="No Error" w967 {
                              frame No Error {
                              }
                              frame Error {
                              }
                            }
                          }
                        }
                        n613 = Build Array(w961, w960) -> (w965:bool[])
                        n614 = Equal?(x=w965, y=TRUE) -> (x = y?=w964:bool[])
                        n615 = And Array Elements(Boolean array=w964) -> (logical AND=w963:bool)
                        n616 = case shown="True" w963 {
                          frame False {
                          }
                          frame True {
                            n617 = local write "ANDOR init"(FALSE ("ANDOR")) -> ()
                          }
                        }
                      }
                    }
                  }
                }
              }
            }
          }
          frame #3 {
            # "exit main loop if everything is deinitialized"
            n618 = local read "shutdown-active"() -> (w971:bool)
            n619 = local read "powermeter init"() -> (w978:bool)
            n620 = local read "spectrograph"() -> (w976:bool)
            n621 = local read "nanostage init"() -> (w979:bool)
            n622 = local read "lightsource"() -> (w977:bool)
            n623 = local read "cameras init"() -> (w980:bool)
            n624 = local read "measure"() -> (w973:bool)
            n625 = local read "xeva init"() -> (w970:bool)
            n626 = Not(x=w971) -> (.not. x?=w975:bool)
            n627 = Build Array(w980, w979, w978, w977, w976, w975, w973, w970) -> (w974:bool[])
            n628 = Or Array Elements(Boolean array=w974) -> (logical OR=w972:bool)
          }
        }
        n629 = node-c288() -> ()  [unwired: 1 in, 1 out]
        n630 = Not(x=w24) -> (.not. x?=→"shutdown-complete":bool)
        n631 = node-c288() -> ()  [unwired: 1 in, 1 out]
      }
      n632 = node-c288(w22) -> ()  [unwired: 1 out]
    }
  }
  n633 = while {
    stop <- w983 stop-if-true
    n634 = event shown="[2] \"shutdown-active\": Value Change" {
      selector: _ -> [_ _ _]
      dyn-events: _ -> [_ _ _]
      timeout: _ -> [_ _ _]
      tunnel: [FALSE TRUE w1008] -> w983
      event "Detected Image": Mouse Up {
        # "click"
        n635 = event-data() -> ("Coords"=w989:T42, "Button"=w990:u16)  [unwired: 1 in, 6 out]
        n636 = local read "magnification"() -> (w986:bool)
        n637 = Equal?(x=w990, y=u16 1) -> (x = y?=w987:bool)
        n638 = Build Array(w986, w987) -> (w985:bool[])
        n639 = And Array Elements(Boolean array=w985) -> (logical AND=w988:bool)
        n640 = case shown="True" w988 {
          tunnel: w989 -> [_ w994]
          frame False {
          }
          frame True {
            n641 = invoke on="Detected Image" class="IntGraph (strict)" method="Map Coords To XY"("Coords"=w994) -> ("XY"=w992:cluster{"X":dbl, "Y":dbl})  [unwired: 6 in, 6 out]
            "click cursor position" <- w992
            n642 = local read "laser-freeze"() -> (w993:bool)
            n643 = case shown="True" w993 {
              tunnel: w992 -> [w995 w1000]
              frame False {
                n644 = property on="Detected Image" class="IntGraph (strict)"("Cursor.Cursor Position"=w995) -> ()  [unwired: 2 in, 2 out]
              }
              frame True {
                w1003 = 10
                n645 = Multiply(x=w1000, y=w1003) -> (x*y=w1001:cluster{"X":dbl, "Y":dbl})
                n646 = Round To Nearest(number=w1001) -> (nearest integer value=w1002:cluster{"X":dbl, "Y":dbl})
                n647 = Divide(x=w1002, y=w1003) -> (x/y=w999:cluster{"X":dbl, "Y":dbl})
                n648 = In Range and Coerce(upper limit=300, x=w999, lower limit=0) -> (coerced(x)=w998:cluster{"X":dbl, "Y":dbl})  [unwired: 1 out]
                n649 = Unbundle By Name(w998) -> ("X"=w1004:dbl, "Y"=w1005:dbl)
                n650 = local write "y-axis"(w1004) -> ()
                n651 = local write "x-axis"(w1005) -> ()
              }
            }
          }
        }
      }
      event Application Instance Close {
        n652 = event-data() -> ()  [unwired: 1 in, 4 out]
        n653 = local write "shutdown"(TRUE ("shutdown")) -> ()
      }
      event "shutdown-active": Value Change {
        n654 = event-data() -> ("NewVal"=w1008:bool)  [unwired: 1 in, 5 out]
      }
    }
  }
  n655 = timed-loop {
    timing: w12 -> [_]
    timing-out: [_] -> w11
    stop <- w1013 stop-if-true
    # "Data Acqu."
    n656 = node-c288() -> ()  [unwired: 1 in, 1 out]
    n657 = local read "cameras init"() -> (w1012:bool)
    n658 = local read "xeva init"() -> (w1011:bool)
    n659 = Build Array(w1011, w1012) -> (w1010:bool[])
    n660 = Or Array Elements(Boolean array=w1010) -> (logical OR=w1009:bool)
    n661 = case shown="False" w1009 {
      frame False {
      }
      frame True {
        n662 = node-c288(i64 10 ("Period")) -> (w1016:T26)  [unwired: 3 in]
        n663 = timed-loop {
          shift-right: [w1021] -> _
          shift-left: T44."noop" ("next action") -> [w1048]
          shift-right: [w1043] -> _
          shift-left: cluster{"Measurement":i32[], "Background":i32[]} {"Measurement"=[], "Background"=[]} ("Data Out") -> [w1045]
          shift-right: [w1039] -> _
          shift-left: T43 {"acquiring out"=FALSE, "Progress"=0, "background"=FALSE, "timer"=0, "finished"=FALSE} ("Progress Out") -> [w1044]
          shift-right: [w1023] -> _
          shift-left: errorcluster {"status"=FALSE, "code"=0, "source"=""} ("error out") -> [w1024]
          timing: w1016 -> [_]
          timing-out: [_] -> w1015
          stop <- w1027 continue-if-true
          n664 = node-c288() -> ()  [unwired: 1 in, 1 out]
          n665 = local read "Exposure Time Read"() -> (w1040:sgl)
          n666 = local read "select background"() -> (w1031:enum16{"skip", "single", "multiple"})
          n667 = local read "readout mode 2"() -> (w1034:u16)
          n668 = local read "Detector Select"() -> (w1036:u16)
          n669 = local read "xeva-camref"() -> (w1032:T23)
          n670 = local read "HBinning"() -> (w1035:u16)
          n671 = local read "ready"() -> (w1033:bool)
          n672 = Bundle By Name(cluster=T45 {"detector"=0, "HBinning"=1, "readout mode"=0, "ready"=FALSE, "Exposure Time Read"=0.0, "select background"=enum."single", "xeva-camref"=refnum} ("acquisition-input-cluster"), "detector"=w1036, "HBinning"=w1035, "readout mode"=w1034, "ready"=w1033, "Exposure Time Read"=w1040, "select background"=w1031, "xeva-camref"=w1032) -> (w1047:T45)
          n673 = call "acquisition-main.vi"("acquisition-input-cluster"=w1047, "error in"=w1024, "Progress In"=w1044, "Data In"=w1045, "input action"=w1048) -> ("error out"=w1023:errorcluster, "Progress Out"=w1039:T43, "Data Out"=w1043:cluster{"Measurement":i32[], "Background":i32[]}, "next action"=w1049:T47)  [unwired: 3 in]
          "Acq Error" <- w1023
          n674 = case shown="\"wait to continue\"" w1049 {
            selector: w1049 -> [w1054 w1056 w1064 w1082 w1092 w1099 w1103 _ w1114]
            tunnel: [w1054 w1058 w1066 w1082 w1092 w1100 w1103 w1105 w1114] -> w1021
            tunnel: "measure" -> [_ w1057 w1065 _ _ _ _ _ _]
            tunnel: "abort-acquisition" -> [_ w1055 w1063 _ _ w1098 _ _ _]
            frame Default {
            }
            frame "noop" {
              n675 = case shown="True" w1055 {
                frame False {
                }
                frame True {
                  n676 = local write "abort-acquisition"(FALSE ("abort-acquisition")) -> ()
                  n677 = local write "measure"(FALSE ("measure")) -> ()
                }
              }
              n678 = case shown="True" w1057 {
                tunnel: [w1061 T46."start" ("next action")] -> w1058
                tunnel: w1056 -> [w1061 _]
                frame False {
                }
                frame True {
                }
              }
            }
            frame "wait to continue" {
              n679 = case shown="False" w1063 {
                tunnel: [w1070 T3."noop" ("next action")] -> w1066
                tunnel: w1065 -> [w1069 _]
                tunnel: w1064 -> [w1068 _]
                frame False {
                  n680 = local read "Save current Spectrum"() -> (w1067:bool)
                  n681 = case shown="False" w1067 {
                    tunnel: [w1074 w1079] -> w1070
                    tunnel: w1069 -> [w1073 _]
                    tunnel: w1068 -> [w1072 w1079]
                    frame False {
                      n682 = case shown="True" w1073 {
                        tunnel: [w1076 T47."start next measurement" ("next action")] -> w1074
                        tunnel: w1072 -> [w1076 _]
                        tunnel: [TRUE ("measurement-finished") FALSE ("measurement-finished")] -> w1071
                        frame False {
                        }
                        frame True {
                        }
                      }
                      "measurement-finished" <- w1071
                    }
                    frame True {
                      # "wait if save is in progress"
                    }
                  }
                }
                frame True {
                  # "go into noop mode\nif abort was pressed"
                }
              }
            }
            frame "set background" {
              n683 = local read "BG shutter"() -> (w1084:T2)
              n684 = local read "spectrograph-input"() -> (w1083:T10)
              n685 = Equal?(x=w1084, y=T2."with Open Shutter") -> (x = y?=w1087:bool)
              n686 = local write "velleman-power"(FALSE ("velleman-power")) -> ()
              n687 = Boolean To (0,1)(Boolean=w1087) -> (0, 1=w1088:i16)
              n688 = Bundle By Name(cluster=w1083, "Shutter"=w1088) -> (w1081:T10)
              n689 = local write "spectrograph-input"(w1081) -> ()
            }
            frame "set measurement" {
              w1093 = u16 1 items=["Close", "Open"] ("Shutter")
              n690 = local read "spectrograph-input"() -> (w1090:T10)
              n691 = local write "velleman-power"(TRUE ("velleman-power")) -> ()
              n692 = Bundle By Name(cluster=w1090, "Shutter"=w1093) -> (w1089:T10)
              n693 = case shown="True" "NKT" {
                frame False {
                }
                frame True {
                  n694 = local read "NKT Input"() -> (w1097:T7)
                  n695 = Bundle By Name(cluster=w1097, "Emission"=TRUE) -> (w1096:T7)
                  n696 = local write "NKT Input"(w1096) -> ()
                }
              }
              n697 = local write "spectrograph-input"(w1089) -> ()
            }
            frame "check progress" {
              n698 = case shown="True" w1098 {
                tunnel: [w1101 T44."abort" ("next action")] -> w1100
                tunnel: w1099 -> [w1101 _]
                frame False {
                }
                frame True {
                }
              }
            }
            frame "get Data" {
              n699 = local read "Power (µW)"() -> (→"Power during measurement":dbl)
            }
            frame "start next measurement" {
              n700 = case shown="False" "align-mode" {
                selector: "align-mode" -> [w1107 w1112]
                tunnel: [T3."wait to continue" ("next action") T47."start next measurement" ("next action")] -> w1105
                frame False {
                  n701 = local write "measure"(w1107) -> ()
                  n702 = case shown="True" "continuos-save" {
                    selector: "continuos-save" -> [_ w1110]
                    frame False {
                    }
                    frame True {
                      # "trigger save at the end of\nthe current measurement"
                      n703 = local write "Save current Spectrum"(w1110) -> ()
                    }
                  }
                }
                frame True {
                  # "do not wait for anything in\nalign mode"
                  n704 = local write "measure"(w1112) -> ()
                }
              }
            }
            frame "abort" {
              n705 = local write "measure"(FALSE ("measure")) -> ()
            }
          }
          "next action" <- w1021
          n706 = Unbundle By Name(w1043) -> ("Measurement"=→"Raw Signal Array":i32[], "Background"=→"Background Array":i32[])
          n707 = Unbundle By Name(w1039) -> ("Progress"=→"Progress":u8, "acquiring out"=→"acquiring":bool, "background"=→"background":bool)
          n708 = local read "cameras init"() -> (w1025:bool)
          n709 = local read "xeva init"() -> (w1026:bool)
          n710 = Build Array(w1026, w1025) -> (w1028:bool[])
          n711 = Or Array Elements(Boolean array=w1028) -> (logical OR=w1027:bool)
          n712 = node-c288(w1023) -> ()  [unwired: 1 out]
        }
        n713 = node-c288(w1015) -> ()  [unwired: 1 out]
      }
    }
    n714 = local read "shutdown-active"() -> (w1013:bool)
    n715 = node-c288() -> ()  [unwired: 1 in, 1 out]
  }
  n716 = timed-loop {
    timing: w16 -> [_]
    timing-out: [_] -> w15
    stop <- w1121 stop-if-true
    # "check GUI controls"
    n717 = node-c288() -> ()  [unwired: 1 in, 1 out]
    n718 = stacked-sequence {
      frame #0 {
        # "Camera Controls 1"
        n719 = stacked-sequence {
          frame #0 {
            n720 = feedback #6(u16 0 ("Horizontal Binning")) -> (w1143:u16)
            n721 = feedback-in #6("HBinning") -> ()
            n722 = Not Equal?(x="HBinning", y=w1143) -> (x != y?=w1140:bool)
            n723 = case shown="True" w1140 {
              frame False {
              }
              frame True {
                w1145 = FALSE ("Binning ok?")
                n724 = local write "abort-acquisition"(TRUE ("abort-acquisition")) -> ()
                n725 = local write "pixel scaling"(w1145) -> ()
                n726 = local write "binning"(w1145) -> ()
              }
            }
          }
        }
        n727 = flat-sequence {
          frame #0 {
            n728 = feedback #7(u16 0 ("Detector Select")) -> (w1131:u16)
            n729 = feedback-in #7("HSSpeed 2") -> ()
            n730 = Not Equal?(x="HSSpeed 2", y=w1131) -> (x != y?=w1129:bool)
            n731 = case shown="True" w1129 {
              frame False {
              }
              frame True {
                n732 = local write "abort-acquisition"(TRUE ("abort-acquisition")) -> ()
                n733 = local write "HSSpeed 3"(FALSE ("pre-amp")) -> ()
              }
            }
          }
        }
        n734 = flat-sequence {
          frame #0 {
            n735 = feedback #8(u16 0 ("Detector Select")) -> (w1154:u16)
            n736 = feedback-in #8("pre-amp 2") -> ()
            n737 = Not Equal?(x="pre-amp 2", y=w1154) -> (x != y?=w1152:bool)
            n738 = case shown="True" w1152 {
              frame False {
              }
              frame True {
                n739 = local write "abort-acquisition"(TRUE ("abort-acquisition")) -> ()
                n740 = local write "pre-amp 3"(FALSE ("pre-amp")) -> ()
              }
            }
          }
        }
        n741 = flat-sequence {
          frame #0 {
            n742 = feedback #9(0.2 ("Set Exposure Time (s)")) -> (w1137:dbl)
            n743 = feedback-in #9("Exposure Time") -> ()
            n744 = Not Equal?(x="Exposure Time", y=w1137) -> (x != y?=w1134:bool)
            n745 = case shown="True" w1134 {
              frame False {
              }
              frame True {
                n746 = local write "abort-acquisition"(TRUE ("abort-acquisition")) -> ()
                n747 = local write "exposure time"(FALSE ("Exposure Time ok?")) -> ()
              }
            }
          }
        }
        n748 = flat-sequence {
          frame #0 {
            n749 = feedback #10(u16 100 ("Detector Select")) -> (w1148:u16)
            n750 = feedback-in #10("readout mode 2") -> ()
            n751 = Not Equal?(x="readout mode 2", y=w1148) -> (x != y?=w1146:bool)
            n752 = case shown="True" w1146 {
              frame False {
              }
              frame True {
                n753 = local write "abort-acquisition"(TRUE ("abort-acquisition")) -> ()
                n754 = local write "readout mode"(FALSE ("readout mode")) -> ()
              }
            }
          }
        }
        n755 = flat-sequence {
          frame #0 {
            n756 = feedback #11(u16 0 ("Detector Select")) -> (w1125:u16)
            n757 = feedback-in #11("ADchannel") -> ()
            n758 = Not Equal?(x="ADchannel", y=w1125) -> (x != y?=w1123:bool)
            n759 = case shown="False" w1123 {
              frame False {
              }
              frame True {
                n760 = local write "ADchannel 2"(FALSE ("pre-amp")) -> ()
                n761 = local write "abort-acquisition"(TRUE ("abort-acquisition")) -> ()
              }
            }
          }
        }
      }
      frame #1 {
        # "Camera Controls 2"
        n762 = flat-sequence {
          frame #0 {
            w1160 = u16 2 items=["Full Vertical Binning", "Image", "Vertical Binning"] ("readout mode")
            n763 = local read "readout mode 2"() -> (w1159:u16)
            n764 = Equal?(x=w1159, y=w1160) -> (x = y?=w1158:bool)
            n765 = case shown="True" w1158 {
              frame False {
              }
              frame True {
                n766 = feedback #12("center") -> (w1163:u16)
                n767 = feedback-in #12("center") -> ()
                n768 = Not Equal?(x="center", y=w1163) -> (x != y?=w1162:bool)
                n769 = case shown="True" w1162 {
                  frame False {
                  }
                  frame True {
                    n770 = local write "abort-acquisition"(TRUE ("abort-acquisition")) -> ()
                    n771 = local write "readout mode"(FALSE ("readout mode")) -> ()
                  }
                }
              }
            }
          }
        }
        n772 = flat-sequence {
          frame #0 {
            w1168 = u16 2 items=["Full Vertical Binning", "Image", "Vertical Binning"] ("readout mode")
            n773 = local read "readout mode 2"() -> (w1167:u16)
            n774 = Equal?(x=w1167, y=w1168) -> (x = y?=w1166:bool)
            n775 = case shown="True" w1166 {
              frame False {
              }
              frame True {
                n776 = feedback #13("height") -> (w1171:u16)
                n777 = feedback-in #13("height") -> ()
                n778 = Not Equal?(x="height", y=w1171) -> (x != y?=w1170:bool)
                n779 = case shown="True" w1170 {
                  frame False {
                  }
                  frame True {
                    n780 = local write "readout mode"(FALSE ("readout mode")) -> ()
                    n781 = local write "abort-acquisition"(TRUE ("abort-acquisition")) -> ()
                  }
                }
              }
            }
          }
        }
        n782 = flat-sequence {
          frame #0 {
            n783 = feedback #14(u16 1 ("Detector Select")) -> (w1177:u16)
            n784 = feedback-in #14("Detector Select") -> ()
            n785 = Not Equal?(x="Detector Select", y=w1177) -> (x != y?=w1174:bool)
            n786 = case shown="True" w1174 {
              frame False {
              }
              frame True {
                n787 = local write "abort-acquisition"(TRUE ("abort-acquisition")) -> ()
                n788 = local write "exposure time"(FALSE ("Exposure Time ok?")) -> ()
                n789 = local write "pixel scaling"(FALSE ("Wavelength")) -> ()
                n790 = local write "detector"(FALSE ("Flipper Status")) -> ()
              }
            }
          }
        }
      }
      frame #2 {
        # "x-wave scaling Controls"
        n791 = stacked-sequence {
          tunnel: [w1243 _] -> w1183
          frame #0 {
            n792 = stacked-sequence {
              seq-local: [w1257 _] -> [_ w1261]
              tunnel: [_ w1262] -> w1245
              tunnel: [_ w1260] -> w1244
              frame #0 {
                n793 = property on="Detected Image" class="IntGraph (strict)"(error in=errorcluster {"status"=FALSE, "code"=0, "source"=""} ("error in (no error)"), "Active Cursor"=u32 0) -> (error out=w1257:errorcluster)  [unwired: 1 in, 1 out]
              }
              frame #1 {
                n794 = property on="Detected Image" class="IntGraph (strict)"(error in=w1261) -> (error out=w1260:errorcluster, "Cursor.Cursor Position"=w1262:T14)  [unwired: 1 in, 1 out]
              }
            }
            n795 = local read "magnification"() -> (w1250:bool)
            n796 = feedback #15(FALSE ("magnification")) -> (w1251:bool)
            n797 = feedback-in #15(w1250) -> ()
            n798 = Not Equal?(x=w1250, y=w1251) -> (x != y?=w1249:bool)
            n799 = feedback #16(T14 {"X"=0.0, "Y"=0.0}) -> (w1256:T14)
            n800 = feedback-in #16(w1245) -> ()
            n801 = Not Equal?(x=w1245, y=w1256) -> (x != y?=w1255:cluster{bool, bool})
            n802 = Cluster To Array(cluster=w1255) -> (array=w1248:bool[])
            n803 = Insert Into Array(array=w1248, index=0, new element=w1249) -> (w1247:bool[])
            n804 = Or Array Elements(Boolean array=w1247) -> (logical OR=w1254:bool)
            n805 = case shown="True" w1254 {
              tunnel: w1245 -> [_ w1278]
              tunnel: w1244 -> [w1263 w1265]
              tunnel: [w1263 w1264] -> w1243
              frame False {
              }
              frame True {
                n806 = property on="Detected Image" class="IntGraph (strict)"(error in=w1265) -> (error out=w1264:errorcluster, "XScale.Offset"=w1276:dbl, "XScale.Multiplier"=w1274:dbl, "YScale.Offset"=w1272:dbl, "YScale.Multiplier"=w1270:dbl)  [unwired: 1 in, 1 out]
                n807 = Unbundle By Name(w1278) -> ("Cursor X"=w1277:dbl, "Cursor Y"=w1273:dbl)
                n808 = Subtract(x=w1277, y=w1276) -> (x-y=w1275:dbl)
                n809 = Subtract(x=w1273, y=w1272) -> (x-y=w1271:dbl)
                n810 = Divide(x=w1275, y=w1274) -> (x/y=w1269:dbl)
                n811 = Divide(x=w1271, y=w1270) -> (x/y=w1268:dbl)
                n812 = Round To Nearest(number=w1268) -> (nearest integer value=w1266:dbl)
                n813 = Round To Nearest(number=w1269) -> (nearest integer value=w1267:dbl)
                n814 = local read "image-laser-position"() -> (w1280:T15)
                n815 = Bundle By Name(cluster=w1280, "laser-x-position"=w1267, "laser-y-position"=w1266) -> (w1279:T15)
                n816 = local write "image-laser-position"(w1279) -> ()
              }
            }
          }
          frame #1 {
            # "check if cursor position changed"
            n817 = feedback #17(T15 {"laser-x-position"=0, "laser-y-position"=0} ("image-laser-position")) -> (w1286:T15)
            n818 = feedback-in #17("image-laser-position") -> ()
            n819 = Not Equal?(x="image-laser-position", y=w1286) -> (x != y?=w1284:T48)
            n820 = Cluster To Array(cluster=w1284) -> (array=w1283:bool[])
            n821 = Or Array Elements(Boolean array=w1283) -> (logical OR=w1282:bool)
            n822 = case shown="True" w1282 {
              tunnel: "image-laser-position" -> [_ w1287]
              frame False {
              }
              frame True {
                # "extend for Vertical Binning"
                n823 = Unbundle By Name(w1287) -> ()  [unwired: 1 out]
                n824 = local write "pixel scaling"(FALSE ("Wavelength")) -> ()
              }
            }
          }
        }
        n825 = flat-sequence {
          frame #0 {
            n826 = local read "spectrograph-output"() -> (w1292:T10)
            n827 = Unbundle By Name(w1292) -> ("Central Wavelength (nm)"=w1291:dbl)
            n828 = feedback #18(0.0 ("Central Wavelength (nm)")) -> (w1293:dbl)
            n829 = feedback-in #18(w1291) -> ()
            n830 = Not Equal?(x=w1291, y=w1293) -> (x != y?=w1289:bool)
            n831 = case shown="True" w1289 {
              frame False {
              }
              frame True {
                n832 = local write "pixel scaling"(FALSE ("Wavelength")) -> ()
              }
            }
          }
        }
        n833 = flat-sequence {
          tunnel: [w1205] -> w1182
          tunnel: w1183 -> [w1204]
          frame #0 {
            n834 = local read "laser-offset"() -> (w1206:bool)
            n835 = feedback #19(FALSE ("laser-offset")) -> (w1209:bool)
            n836 = feedback-in #19(w1206) -> ()
            n837 = Not Equal?(x=w1206, y=w1209) -> (x != y?=w1207:bool)
            n838 = case shown="False" w1207 {
              tunnel: [w1210 w1213] -> w1205
              tunnel: w1204 -> [w1210 w1212]
              frame False {
              }
              frame True {
                n839 = local read "laser-freeze"() -> (w1211:bool)
                n840 = stacked-sequence {
                  seq-local: [w1216 _] -> [_ w1218]
                  tunnel: w1211 -> [_ w1220]
                  tunnel: [_ w1221] -> w1213
                  tunnel: w1212 -> [w1215 _]
                  frame #0 {
                    n841 = property on="Detected Image" class="IntGraph (strict)"(error in=w1215, "Active Cursor"=u32 0) -> (error out=w1216:errorcluster)  [unwired: 1 in, 1 out]
                  }
                  frame #1 {
                    n842 = Not(x=w1220) -> (.not. x?=w1219:bool)
                    n843 = property on="Detected Image" class="IntGraph (strict)"(error in=w1218, "Cursor.Visible"=w1219) -> (error out=w1221:errorcluster)  [unwired: 1 in, 1 out]
                  }
                }
                n844 = local write "pixel scaling"(FALSE ("Wavelength")) -> ()
              }
            }
          }
        }
        n845 = flat-sequence {
          frame #0 {
            n846 = local read "magnification"() -> (w1230:dbl)
            n847 = local read "magnification"() -> (w1222:bool)
            n848 = feedback #20(FALSE ("magnification")) -> (w1225:bool)
            n849 = feedback-in #20(w1222) -> ()
            n850 = feedback #21(0.0 ("Central Wavelength (nm)")) -> (w1229:dbl)
            n851 = feedback-in #21(w1230) -> ()
            n852 = Not Equal?(x=w1222, y=w1225) -> (x != y?=w1224:bool)
            n853 = Not Equal?(x=w1230, y=w1229) -> (x != y?=w1227:bool)
            n854 = Or(x=w1224, y=w1227) -> (x .or. y?=w1226:bool)
            n855 = case shown="True" w1226 {
              frame False {
              }
              frame True {
                n856 = stacked-sequence {
                  seq-local: [w1232 _ _ _] -> [_ w1236 _ _]
                  seq-local: [_ w1235 _ _] -> [_ _ w1238 _]
                  seq-local: [_ _ w1237 _] -> [_ _ _ w1242]
                  tunnel: [_ _ _ w1241] -> _
                  frame #0 {
                    n857 = property on="Detected Image" class="IntGraph (strict)"("Active Cursor"=u32 1) -> (error out=w1232:errorcluster)  [unwired: 2 in, 1 out]
                  }
                  frame #1 {
                    n858 = property on="Detected Image" class="IntGraph (strict)"(error in=w1236, "Cursor.Visible"=FALSE) -> (error out=w1235:errorcluster)  [unwired: 1 in, 1 out]
                  }
                  frame #2 {
                    n859 = property on="Detected Image" class="IntGraph (strict)"(error in=w1238, "Active Cursor"=u32 0) -> (error out=w1237:errorcluster)  [unwired: 1 in, 1 out]
                  }
                  frame #3 {
                    n860 = property on="Detected Image" class="IntGraph (strict)"(error in=w1242, "Cursor.Visible"=FALSE) -> (error out=w1241:errorcluster)  [unwired: 1 in, 1 out]
                  }
                }
                n861 = local write "pixel scaling"(FALSE ("Wavelength")) -> ()
              }
            }
          }
        }
        n862 = flat-sequence {
          tunnel: w1182 -> [w1184]
          frame #0 {
            n863 = local read "laser-freeze"() -> (w1185:bool)
            n864 = feedback #22(FALSE ("laser-offset")) -> (w1188:bool)
            n865 = feedback-in #22(w1185) -> ()
            n866 = Not Equal?(x=w1185, y=w1188) -> (x != y?=w1186:bool)
            n867 = case shown="True" w1186 {
              tunnel: w1185 -> [_ w1189]
              tunnel: w1184 -> [_ w1190]
              frame False {
              }
              frame True {
                # "some\nmagic\nhere"
                n868 = stacked-sequence {
                  seq-local: [w1192 _ _ _] -> [_ w1195 _ _]
                  seq-local: [_ w1194 _ _] -> [_ _ w1198 _]
                  seq-local: [_ _ w1197 _] -> [_ _ _ w1203]
                  tunnel: w1189 -> [_ w1196 _ w1201]
                  tunnel: w1190 -> [w1191 _ _ _]
                  tunnel: [_ _ _ w1202] -> _
                  frame #0 {
                    n869 = property on="Detected Image" class="IntGraph (strict)"(error in=w1191, "Active Cursor"=u32 1) -> (error out=w1192:errorcluster)  [unwired: 1 in, 1 out]
                  }
                  frame #1 {
                    n870 = property on="Detected Image" class="IntGraph (strict)"(error in=w1195, "Cursor.Visible"=w1196) -> (error out=w1194:errorcluster)  [unwired: 1 in, 1 out]
                  }
                  frame #2 {
                    n871 = property on="Detected Image" class="IntGraph (strict)"(error in=w1198, "Active Cursor"=u32 0) -> (error out=w1197:errorcluster)  [unwired: 1 in, 1 out]
                  }
                  frame #3 {
                    n872 = Not(x=w1201) -> (.not. x?=w1200:bool)
                    n873 = property on="Detected Image" class="IntGraph (strict)"(error in=w1203, "Cursor.Visible"=w1200) -> (error out=w1202:errorcluster)  [unwired: 1 in, 1 out]
                  }
                }
                n874 = local write "measure"(w1189) -> ()
              }
            }
          }
        }
      }
      frame #3 {
        # "check if switch buttons were pressed\ncorrect once displayed values"
        # "Check Nanostage Controls"
        n875 = stacked-sequence {
          frame #0 {
            n876 = local read "init nanostage"() -> (w1309:bool)
            n877 = case shown="True" w1309 {
              frame False {
              }
              frame True {
                n878 = local read "z-axis"() -> (w1315:dbl)
                n879 = local read "x-axis"() -> (w1317:dbl)
                n880 = local read "y-axis"() -> (w1316:dbl)
                n881 = Bundle("x-axis"=w1317, "y-axis"=w1316, "z-axis"=w1315) -> (w1313:T49)  [unwired: 1 in]
                n882 = feedback #23() -> (w1314:T49)  [unwired: 1 in]
                n883 = feedback-in #23(w1313) -> ()
                n884 = Not Equal?(x=w1313, y=w1314) -> (x != y?=w1312:T50)
                n885 = Cluster To Array(cluster=w1312) -> (array=w1311:bool[])
                n886 = Or Array Elements(Boolean array=w1311) -> (logical OR=w1310:bool)
                n887 = case shown="True" w1310 {
                  frame False {
                  }
                  frame True {
                    # "deprecated?"
                    n888 = local read "laser-freeze"() -> (w1318:bool)
                    n889 = local write "pixel scaling"(w1318) -> ()
                  }
                }
              }
            }
          }
        }
        n890 = flat-sequence {
          frame #0 {
            n891 = local read "switch U/D"() -> (w1304:bool)
            n892 = feedback #24(FALSE ("switch U/D")) -> (w1305:bool)
            n893 = feedback-in #24(w1304) -> ()
            n894 = Not Equal?(x=w1304, y=w1305) -> (x != y?=w1303:bool)
            n895 = case shown="True" w1303 {
              selector: w1303 -> [_ w1306]
              frame False {
              }
              frame True {
                n896 = local read "x-axis"() -> (w1308:dbl)
                n897 = call "utility-flip-stage.vi"("axis in"=w1308, "flip"=w1306) -> ("axis out"=w1307:dbl)
                n898 = local write "x-axis"(w1307) -> ()
              }
            }
          }
        }
        n899 = flat-sequence {
          frame #0 {
            n900 = local read "switch L/R"() -> (w1297:bool)
            n901 = feedback #25(FALSE ("switch L/R")) -> (w1296:bool)
            n902 = feedback-in #25(w1297) -> ()
            n903 = Not Equal?(x=w1297, y=w1296) -> (x != y?=w1298:bool)
            n904 = case shown="True" w1298 {
              selector: w1298 -> [_ w1300]
              frame False {
              }
              frame True {
                n905 = local read "y-axis"() -> (w1301:dbl)
                n906 = call "utility-flip-stage.vi"("axis in"=w1301, "flip"=w1300) -> ("axis out"=w1299:dbl)
                n907 = local write "y-axis"(w1299) -> ()
              }
            }
          }
        }
      }
      frame #4 {
        # "check lightsource"
        n908 = flat-sequence {
          frame #0 {
            n909 = local read "lightsource"() -> (w1319:bool)
            n910 = case shown="True" w1319 {
              tunnel: [FALSE w1322] -> w1320
              frame False {
              }
              frame True {
                n911 = local read "NKT Input"() -> (w1325:T7)
                n912 = feedback #26(w1325) -> (w1326:T7)
                n913 = feedback-in #26(w1325) -> ()
                n914 = Not Equal?(x=w1325, y=w1326) -> (x != y?=w1324:T51)
                n915 = Cluster To Array(cluster=w1324) -> (array=w1323:bool[])
                n916 = Or Array Elements(Boolean array=w1323) -> (logical OR=w1322:bool)
              }
            }
            "lightsource-set" <- w1320
          }
        }
      }
      frame #5 {
        # "check if Display has to be updated"
        n917 = flat-sequence {
          frame #0 {
            n918 = local read "Raw Signal Array"() -> (w1340:i32[])
            n919 = feedback #27() -> (w1339:i32[])  [unwired: 1 in]
            n920 = feedback-in #27(w1340) -> ()
            n921 = Not Equal?(x=w1339, y=w1340) -> (x != y?=w1338:bool[])
            n922 = Or Array Elements(Boolean array=w1338) -> (logical OR=w1337:bool)
            n923 = case shown="True" w1337 {
              frame False {
              }
              frame True {
                n924 = local write "refresh display"(TRUE ("refresh display")) -> ()
              }
            }
          }
        }
        n925 = flat-sequence {
          frame #0 {
            n926 = feedback #28(FALSE ("background 2")) -> (w1335:bool)
            n927 = feedback-in #28("background") -> ()
            n928 = Not Equal?(x="background", y=w1335) -> (x != y?=w1332:bool)
            n929 = case shown="True" w1332 {
              frame False {
              }
              frame True {
                n930 = local write "refresh display"(TRUE ("refresh display")) -> ()
              }
            }
          }
        }
        n931 = flat-sequence {
          frame #0 {
            n932 = feedback #29(FALSE ("autoscale")) -> (w1329:bool)
            n933 = feedback-in #29("autoscale") -> ()
            n934 = Not Equal?(x="autoscale", y=w1329) -> (x != y?=w1327:bool)
            n935 = case shown="True" w1327 {
              frame False {
              }
              frame True {
                n936 = local write "refresh display"(TRUE ("refresh display")) -> ()
              }
            }
          }
        }
      }
      frame #6 {
        # "check if ready"
        n937 = local read "init spectrograph"() -> (w1345:bool)
        n938 = local read "nanostage init"() -> (w1346:bool)
        n939 = local read "init cameras"() -> (w1347:bool)
        n940 = case shown="True" w1345 {
          tunnel: [TRUE w1362] -> w1343
          frame False {
          }
          frame True {
            # "check spectrograph"
            n941 = local read "spectrograph-status"() -> (w1361:T9)
            n942 = local read "detector"() -> (w1365:bool)
            n943 = Cluster To Array(cluster=w1361) -> (array=w1363:bool[])
            n944 = Build Array (concatenate)(w1363, w1365) -> (w1364:bool[])
            n945 = And Array Elements(Boolean array=w1364) -> (logical AND=w1362:bool)
          }
        }
        n946 = case shown="True" w1346 {
          tunnel: [TRUE w1356] -> w1348
          frame False {
          }
          frame True {
            n947 = local read "getValues"() -> (w1359:cluster{"postion":dbl[], "status":bool[]})
            n948 = Unbundle By Name(w1359) -> ("status"=w1358:bool[])
            n949 = Not(x=w1358) -> (.not. x?=w1357:bool[])
            n950 = And Array Elements(Boolean array=w1357) -> (logical AND=w1356:bool)
          }
        }
        n951 = case shown="True" w1347 {
          tunnel: [TRUE w1351] -> w1349
          frame False {
          }
          frame True {
            # "maybe also add the other properties"
            # "check detector"
            n952 = local read "exposure time"() -> (w1353:bool)
            n953 = local read "detector"() -> (w1354:bool)
            n954 = Build Array(w1354, w1353) -> (w1352:bool[])
            n955 = And Array Elements(Boolean array=w1352) -> (logical AND=w1351:bool)
          }
        }
        n956 = Build Array(w1343, w1348, w1349) -> (w1342:bool[])
        n957 = And Array Elements(Boolean array=w1342) -> (logical AND=→"ready":bool)
      }
      frame #7 {
        # "deinitialize devices"
        n958 = local read "shutdown-active"() -> (w1366:bool)
        n959 = case shown="False" w1366 {
          frame False {
          }
          frame True {
            w1368 = FALSE
            n960 = local write "abort-acquisition"(TRUE ("abort-acquisition")) -> ()
            n961 = local write "init nanostage"(w1368) -> ()
            n962 = local write "init powermeter"(w1368) -> ()
            n963 = local write "init spectrograph"(w1368) -> ()
            n964 = local write "init cameras"(w1368) -> ()
            n965 = local write "init lightsource"(w1368) -> ()
            n966 = local write "measure"(w1368) -> ()
            n967 = local write "init xeva"(w1368) -> ()
          }
        }
      }
    }
    n968 = local read "shutdown-active"() -> (w1121:bool)
    n969 = node-c288() -> ()  [unwired: 1 in, 1 out]
  }
  n970 = node-c288() -> (w2:T26)  [unwired: 4 in]
  n971 = node-c288(w15) -> ()  [unwired: 1 out]
  n972 = timed-loop {
    timing: w2 -> [_]
    timing-out: [_] -> w1
    stop <- "shutdown" stop-if-true
    n973 = node-c288() -> ()  [unwired: 1 in, 1 out]
    n974 = case shown="True" "shutdown" {
      selector: "shutdown" -> [_ w1372]
      frame False {
      }
      frame True {
        w1373 = T31."Enabled" ("Disabled")
        # "signal event"
        # "makes sense??"
        n975 = property on="shutdown-active" class="Bool (strict)"("Val(Sgnl)"=w1372) -> ()  [unwired: 2 in, 2 out]
        n976 = property on="Save current Spectrum" class="Bool (strict)"("DisabledEnum"=w1373) -> ()  [unwired: 2 in, 2 out]
        n977 = property on="STOP PLE" class="Bool (strict)"("DisabledEnum"=w1373) -> ()  [unwired: 2 in, 2 out]
        n978 = property on="HBinning" class="Ring (strict)"("DisabledEnum"=w1373) -> ()  [unwired: 2 in, 2 out]
        n979 = property on="binning" class="Bool (strict)"("DisabledEnum"=w1373) -> ()  [unwired: 2 in, 2 out]
        "shutdown-active" <- w1372
      }
    }
    n980 = node-c288() -> ()  [unwired: 1 in, 1 out]
  }
  n981 = node-c288(i64 50 ("Period")) -> (w18:T26)  [unwired: 3 in]
  n982 = timed-loop {
    timing: w18 -> [_]
    timing-out: [_] -> w17
    stop <- w1376 stop-if-true
    # "Display"
    n983 = node-c288() -> ()  [unwired: 1 in, 1 out]
    n984 = case shown="False" "refresh display" {
      frame False {
      }
      frame True {
        n985 = local read "Raw Signal Array"() -> (w1404:i32[])
        n986 = flat-sequence {
          tunnel: [w1407] -> w1391
          tunnel: [w1406] -> w1390
          tunnel: w1391 -> [w1418]
          tunnel: w1390 -> [w1416]
          tunnel: w1389 -> [w1414]
          tunnel: [w1414] -> w1388
          tunnel: w1387 -> [w1419]
          tunnel: [w1419] -> w1386
          tunnel: w1385 -> [w1412]
          tunnel: [w1412] -> w1384
          tunnel: w1383 -> [w1417]
          tunnel: [w1417] -> w1382
          tunnel: w1381 -> [w1420]
          tunnel: [w1420] -> w1380
          tunnel: [w1409] -> w1379
          tunnel: w1388 -> [w1426]
          tunnel: w1386 -> [w1425]
          tunnel: w1384 -> [w1424]
          tunnel: w1382 -> [w1423]
          tunnel: w1380 -> [w1422]
          tunnel: w1379 -> [w1421]
          frame #0 {
            n987 = property on="Detected Image" class="IntGraph (strict)"("Active Cursor"=u32 0) -> ()  [unwired: 2 in, 2 out]
          }
          frame #1 {
            n988 = local read "image-laser-position"() -> (w1408:T15)
            n989 = Unbundle By Name(w1408) -> ("laser-x-position"=w1407:u16, "laser-y-position"=w1406:u16)
          }
          frame #2 {
            n990 = Multiply(x=w1419, y=w1418) -> (x*y=w1415:dbl)
            n991 = Multiply(x=w1416, y=w1417) -> (x*y=w1413:dbl)
            n992 = Add(x=w1414, y=w1415) -> (x+y=w1410:dbl)
            n993 = Add(x=w1413, y=w1412) -> (x+y=w1411:dbl)
            n994 = Bundle(w1410, w1411) -> (w1409:cluster{dbl, dbl})  [unwired: 1 in]
          }
          frame #3 {
            n995 = property on="Detected Image" class="IntGraph (strict)"("XScale.Offset"=w1426, "XScale.Multiplier"=w1425, "YScale.Offset"=w1424, "YScale.Multiplier"=w1423, "YScale.UnitLabel.Text"=w1422, "XScale.UnitLabel.Text"=w1422, "Cursor.Cursor Position"=w1421) -> ()  [unwired: 2 in, 2 out]
          }
        }
        n996 = local read "autoscale"() -> (w1392:bool)
        n997 = local read "background"() -> (w1393:bool)
        n998 = local read "x-scale array"() -> (w1402:sgl[])
        n999 = local read "Pixel Scaling"() -> (w1396:T16)
        n1000 = local write "refresh display"(FALSE ("refresh display")) -> ()
        n1001 = Unbundle By Name(w1396) -> ("size x"=w1394:u16, "size y"=w1395:u16, "first x"=w1389:sgl, "deltax"=w1387:dbl, "first y"=w1385:sgl, "deltay"=w1383:dbl, "unit"=w1381:string)
        n1002 = case shown="False" w1393 {
          tunnel: [w1445 w1446] -> w1401
          tunnel: w1404 -> [w1445 w1447]
          frame False {
          }
          frame True {
            n1003 = local read "Background Array"() -> (w1448:i32[])
            n1004 = Subtract(x=w1447, y=w1448) -> (x-y=w1446:i32[])
          }
        }
        n1005 = local read "readout mode 2"() -> (w1403:u16)
        n1006 = case shown="0, Default" w1403 {
          tunnel: w1402 -> [w1431 w1437]
          tunnel: w1401 -> [w1432 w1441]
          tunnel: w1392 -> [w1430 w1435]
          tunnel: [w1432 w1436] -> w1397
          tunnel: [w1431 w1437] -> w1399
          tunnel: [w1430 w1435] -> w1398
          tunnel: w1395 -> [_ w1434]
          tunnel: w1394 -> [_ w1433]
          frame 0, Default {
          }
          frame 1 {
            # "image mode"
            n1007 = case shown="True" w1435 {
              tunnel: w1441 -> [_ w1444]
              frame False {
              }
              frame True {
                # "autoscale"
                n1008 = Array Max & Min(array=w1444) -> (max value=w1443:i32, min value=w1442:i32)  [unwired: 2 out]
                n1009 = property on="Detected Image" class="IntGraph (strict)"("ZScale.Maximum"=w1443, "ZScale.Minimum"=w1442) -> ()  [unwired: 2 in, 2 out]
              }
            }
            n1010 = property on="Detected Image" class="IntGraph (strict)"() -> ("Cursor.Cursor Y"=w1440:dbl)  [unwired: 2 in, 2 out]
            n1011 = Reshape Array(w1441, w1434, w1433) -> (w1438:i32[][])
            "Detected Image" <- w1438
            n1012 = Round To Nearest(number=w1440) -> (nearest integer value=w1439:dbl)
            n1013 = Index Array(array=w1438, index (row)=w1439) -> (element=w1436:i32[])  [unwired: 1 in]
          }
        }
        n1014 = case shown="True" w1398 {
          tunnel: w1397 -> [_ w1427]
          frame False {
          }
          frame True {
            n1015 = Array Max & Min(array=w1427) -> (max value=w1428:i32, min value=w1429:i32)  [unwired: 2 out]
            n1016 = property on="Data Plot" class="XYGraph (strict)"("YScale.Minimum"=w1429) -> ()  [unwired: 2 in, 2 out]
            n1017 = property on="Data Plot" class="XYGraph (strict)"("YScale.Maximum"=w1428) -> ()  [unwired: 2 in, 2 out]
          }
        }
        n1018 = Bundle("x-scale array"=w1399, "Raw Signal Array"=w1397) -> (→"Data Plot":T52)  [unwired: 1 in]
      }
    }
    n1019 = local read "shutdown-active"() -> (w1376:bool)
    n1020 = node-c288() -> ()  [unwired: 1 in, 1 out]
  }
  n1021 = node-c288(w11) -> ()  [unwired: 1 out]
  n1022 = node-c288(i64 25 ("Offset")) -> (w8:T26)  [unwired: 4 in]
  n1023 = timed-loop {
    timing: w8 -> [_]
    timing-out: [_] -> w7
    stop <- w1451 stop-if-true
    # "Measurement Programs"
    n1024 = node-c288() -> ()  [unwired: 1 in, 1 out]
    n1025 = stacked-sequence {
      frame #0 {
        # "timed Measurement"
        n1026 = stacked-sequence {
          tunnel: "timed-start" -> [w1453 w1470]
          frame #0 {
            n1027 = feedback #30(FALSE ("example-measurement-start")) -> (w1454:bool)
            n1028 = feedback-in #30(w1453) -> ()
            n1029 = Not Equal?(x=w1453, y=w1454) -> (x != y?=w1456:bool)
            n1030 = case shown="True" w1456 {
              tunnel: w1453 -> [_ w1457]
              frame False {
              }
              frame True {
                n1031 = case shown="True" w1457 {
                  frame False {
                    n1032 = local read "NKT Input"() -> (w1460:T7)
                    n1033 = Bundle By Name(cluster=w1460, "Emission"=FALSE) -> (w1459:T7)
                    n1034 = local write "shutdown"("timed-shutdown") -> ()
                    n1035 = local write "NKT Input"(w1459) -> ()
                  }
                  frame True {
                    n1036 = Get Date/Time In Seconds() -> (seconds since 1Jan1904=→"timed-timestamp":timestamp)
                    n1037 = case shown="\"spectrum\", Default" "timed-type" {
                      frame "spectrum", Default {
                        n1038 = local write "measure"(TRUE ("measure")) -> ()
                        n1039 = local write "measurement-finished"(FALSE ("measurement-finished")) -> ()
                      }
                      frame "AutoStage" {
                        n1040 = local write "autostage-start"(TRUE ("autostage-start")) -> ()
                      }
                      frame "PLE" {
                        n1041 = local write "PLE Acquisition\nfinished?"(FALSE ("PLE Acquisition\nfinished?")) -> ()
                        n1042 = local write "Start PLE Scan"(TRUE ("Start PLE Scan")) -> ()
                      }
                    }
                    "timed-counter" <- u32 0 ("timed-counter")
                  }
                }
              }
            }
          }
          frame #1 {
            n1043 = case shown="True" w1470 {
              frame False {
              }
              frame True {
                w1473 = 100.0 ("x")
                n1044 = Get Date/Time In Seconds() -> (seconds since 1Jan1904=w1472:timestamp)
                n1045 = local read "timed-timestamp"() -> (w1478:timestamp)
                n1046 = local read "timed-type"() -> (w1471:enum16{"spectrum", "AutoStage", "PLE"})
                n1047 = Subtract(x=w1472, y=w1478) -> (x-y=w1477:dbl)
                n1048 = Divide(x=w1477, y="timed-wait") -> (x/y=w1475:dbl)
                n1049 = case shown="\"spectrum\", Default" w1471 {
                  tunnel: [w1480 w1481 w1483] -> w1479
                  frame "spectrum", Default {
                    n1050 = local read "measurement-finished"() -> (w1480:bool)
                  }
                  frame "AutoStage" {
                    n1051 = local read "autostage-start"() -> (w1482:bool)
                    n1052 = Not(x=w1482) -> (.not. x?=w1481:bool)
                  }
                  frame "PLE" {
                    n1053 = local read "PLE Acquisition\nfinished?"() -> (w1483:bool)
                  }
                }
                n1054 = Multiply(x=w1473, y=w1475) -> (x*y=w1474:dbl)
                "waiting" <- w1474
                n1055 = case shown="True" w1479 {
                  tunnel: w1474 -> [_ w1486]
                  tunnel: w1473 -> [_ w1485]
                  tunnel: w1472 -> [_ w1484]
                  frame False {
                  }
                  frame True {
                    n1056 = Greater?(x=w1486, y=w1485) -> (0:w1487:bool)
                    n1057 = case shown="True" w1487 {
                      tunnel: w1484 -> [_ w1492]
                      frame False {
                      }
                      frame True {
                        n1058 = local read "timed-counter"() -> (w1491:u32)
                        n1059 = local write "timed-timestamp"(w1492) -> ()
                        n1060 = Increment(x=w1491) -> (x+1=w1490:u32)
                        n1061 = Less?(x=w1490, y="timed-counter-stop") -> (x < y?=w1488:bool)
                        n1062 = case shown="True" w1488 {
                          frame False {
                            n1063 = local write "timed-start"(FALSE ("timed-start")) -> ()
                          }
                          frame True {
                            n1064 = local read "timed-type"() -> (w1494:enum16{"spectrum", "AutoStage", "PLE"})
                            n1065 = case shown="\"PLE\"" w1494 {
                              frame "spectrum", Default {
                                n1066 = local write "measure"(TRUE ("measure")) -> ()
                              }
                              frame "AutoStage" {
                                n1067 = local write "autostage-start"(TRUE ("autostage-start")) -> ()
                              }
                              frame "PLE" {
                                n1068 = local write "PLE Acquisition\nfinished?"(FALSE ("PLE Acquisition\nfinished?")) -> ()
                                n1069 = local write "Start PLE Scan"(TRUE ("Start PLE Scan")) -> ()
                              }
                            }
                          }
                        }
                        n1070 = local write "timed-counter"(w1490) -> ()
                      }
                    }
                  }
                }
              }
            }
          }
        }
      }
      frame #1 {
        # "autostage\ncontrol"
        n1071 = stacked-sequence {
          tunnel: "autostage-start" -> [w1503 w1514 _]
          tunnel: "stage-timed-type" -> [w1501 w1513 _]
          frame #0 {
            # "initialization of autostage"
            n1072 = feedback #31(FALSE ("cycle-trigger")) -> (w1504:bool)
            n1073 = feedback-in #31(w1503) -> ()
            n1074 = Not Equal?(x=w1503, y=w1504) -> (x != y?=w1502:bool)
            n1075 = case shown="True" w1502 {
              tunnel: w1501 -> [_ w1506]
              frame False {
              }
              frame True {
                # "reset on abort"
                n1076 = local write "cycle-iterator"(0 ("cycle-iterator")) -> ()
                n1077 = case shown="\"PLE\"" w1506 {
                  frame "spectrum", Default {
                    # "not measuring but autostage pressed:\ninitially set parameters"
                    n1078 = local read "measure"() -> (w1509:bool)
                    n1079 = case shown="False" w1509 {
                      frame False {
                        # "powermeter auto-zero off"
                        # "fake to set first parameter"
                        n1080 = local write "measurement-finished"(TRUE ("measure")) -> ()
                        n1081 = local write "Perform Auto Zero"(FALSE ("Perform Auto Zero")) -> ()
                      }
                      frame True {
                      }
                    }
                  }
                  frame "PLE" {
                    # "fake finished for first cycle and on abort"
                    n1082 = local write "PLE Acquisition\nfinished?"(TRUE ("PLE Acquisition\nfinished?")) -> ()
                  }
                }
                n1083 = local write "continuos-save"(FALSE ("continuos-save")) -> ()
              }
            }
          }
          frame #1 {
            n1084 = case shown="False" w1514 {
              tunnel: w1513 -> [_ w1576]
              frame False {
                # "this is a little bit hacky but it works. remove for a more lean solution"
                # "calculate coordinates when not measuring"
                n1085 = feedback #32(FALSE ("cycle-load-coordinates")) -> (w1523:bool)
                n1086 = feedback-in #32("cycle-load-coordinates") -> ()
                n1087 = feedback #33(T17 {"cycle-x-mod"=0, "cycle-x-range-min"=0.0, "cycle-x-range-max"=0.0, "cycle-x-step"=0.0, "cycle-y-mod"=0, "cycle-y-range-min"=0.0, "cycle-y-range-max"=0.0, "cycle-y-step"=0.0, "cycle-z-mod"=0, "cycle-z-range-min"=0.0, "cycle-z-range-max"=0.0, "cycle-z-step"=0.0} ("Cluster")) -> (w1534:T17)
                n1088 = feedback-in #33("Cycle Cluster") -> ()
                n1089 = Not Equal?(x="cycle-load-coordinates", y=w1523) -> (x != y?=w1519:bool)
                n1090 = Not(x="cycle-load-coordinates") -> (.not. x?=w1520:bool)
                n1091 = Not Equal?(x=w1534, y="Cycle Cluster") -> (x != y?=w1531:T53)
                n1092 = And(x=w1520, y=w1519) -> (x .and. y?=w1515:bool)
                n1093 = And(x="cycle-load-coordinates", y=w1519) -> (x .and. y?=w1517:bool)
                n1094 = Cluster To Array(cluster=w1531) -> (array=w1530:bool[])
                n1095 = case shown="True" w1517 {
                  tunnel: [dbl[][] [] w1567] -> w1526
                  tunnel: [dbl[][] [] w1560] -> w1516
                  frame False {
                  }
                  frame True {
                    w1564 = 0 ("start of read offset (chars.:0)")
                    n1096 = call-poly <vilib>:"Read Delimited Spreadsheet.vi"("format (%.3f)"="%.2f", "number of rows (all:-1)"=-1, "start of read offset (chars.:0)"=w1564, "max characters/row  (no limit:0)"=w1564, "error in (no error)"=errorcluster {"status"=FALSE, "code"=0, "source"=""}, "transpose? (F)"=TRUE, "delimiter (\\t)"="," ("delimiter (\\t)")) -> ("all rows"=w1561:dbl[][], "error out"=→"error out":errorcluster)  [unwired: 3 in, 4 out]
                    n1097 = Array Subset(array=w1561, index (row)=3 ("index"), length (row)=2 ("length")) -> (w1560:dbl[][])  [unwired: 2 in]
                    n1098 = Array Subset(array=w1561, index (row)=0 ("index"), length (row)=3 ("length")) -> (w1567:dbl[][])  [unwired: 2 in]
                  }
                }
                n1099 = case shown="False" w1519 {
                  tunnel: "cycle-load-coordinates" -> [_ w1535]
                  frame False {
                  }
                  frame True {
                    n1100 = Select(t=T31."Disabled and Grayed Out" ("Disabled"), s=w1535, f=T31."Enabled" ("Disabled")) -> (s? t:f=w1538:T31)
                    n1101 = property on="Cycle Cluster" class="Clust (strict)"("DisabledEnum"=w1538) -> ()  [unwired: 2 in, 2 out]
                  }
                }
                n1102 = Insert Into Array "Insert Into Array"(array=w1530, index=0, new element=w1515) -> (w1528:bool[])
                n1103 = Or Array Elements(Boolean array=w1528) -> (logical OR=w1525:bool)
                n1104 = Or(x=w1525, y=w1517) -> (x .or. y?=w1524:bool)
                n1105 = case shown="True" w1525 {
                  tunnel: "Cycle Cluster" -> [_ w1575]
                  tunnel: [dbl[][] [] ("coordinates") w1573] -> w1527
                  frame False {
                  }
                  frame True {
                    n1106 = call "autostage-buildcoordinates.vi"("inclusive end"=TRUE, "Cluster"=w1575) -> ("coordinates"=w1573:dbl[][])
                  }
                }
                n1107 = Select(t=w1526, s=w1517, f=w1527) -> (s? t:f=w1518:dbl[][])
                n1108 = case shown="True" w1524 {
                  tunnel: w1518 -> [_ w1547]
                  tunnel: w1516 -> [_ w1539]
                  frame False {
                  }
                  frame True {
                    n1109 = call "autostage-coordinates-minmax.vi"("coordinates"=w1547) -> ("x-max"=w1546:u16, "x-min"=w1545:u16, "y-max"=w1544:u16, "y-min"=w1543:u16)
                    n1110 = local read "Exposure Time Read"() -> (w1551:sgl)
                    n1111 = call "autostage-coordinates-to-graph.vi"("coordinates"=w1547) -> ("graph array"=→"Coordinate Graph":dbl[][])
                    n1112 = property on="coordinates" class="Arr (strict)"("Index Values"=u32[] []) -> ()  [unwired: 2 in, 2 out]
                    n1113 = Index Array(array=w1547, index (row)=0) -> (element=w1549:dbl[])  [unwired: 1 in]
                    n1114 = property on="Coordinate Graph" class="IntGraph (strict)"("XScale.Maximum"=w1546, "XScale.Minimum"=w1545, "YScale.Maximum"=w1544, "YScale.Minimum"=w1543) -> ()  [unwired: 2 in, 2 out]
                    n1115 = local read "select background"() -> (w1540:enum16{"skip", "single", "multiple"})
                    n1116 = Array Size(array=w1549) -> (size(s)=w1550:i32)
                    "cycle-num" <- w1550
                    n1117 = Multiply(x=w1550, y=w1551) -> (x*y=w1552:sgl)
                    n1118 = Divide(x=w1552, y=sgl 60.0) -> (x/y=w1542:sgl)
                    n1119 = Multiply(x=w1542, y=w1540) -> (x*y=→"cycle-time":sgl)
                    "coordinates" <- w1547
                    "excitation" <- w1539
                  }
                }
              }
              frame True {
                # "autostage cycle"
                n1120 = case shown="\"spectrum\", Default" w1576 {
                  tunnel: [w1578 w1579] -> w1577
                  frame "spectrum", Default {
                    n1121 = local read "measurement-finished"() -> (w1578:bool)
                  }
                  frame "PLE" {
                    n1122 = local read "PLE Acquisition\nfinished?"() -> (w1579:bool)
                  }
                }
                n1123 = case shown="False" w1577 {
                  tunnel: w1576 -> [_ w1582]
                  frame False {
                  }
                  frame True {
                    n1124 = case shown="\"PLE\"" w1582 {
                      frame "spectrum", Default {
                        n1125 = local write "measurement-finished"(FALSE ("measurement-finished")) -> ()
                      }
                      frame "PLE" {
                        n1126 = local write "PLE Acquisition\nfinished?"(FALSE ("PLE Acquisition\nfinished?")) -> ()
                      }
                    }
                    n1127 = case shown="\"spectrum\", Default" w1582 {
                      tunnel: "cycle-save-data" -> [w1590 _]
                      frame "spectrum", Default {
                        n1128 = local write "continuos-save"(w1590) -> ()
                      }
                      frame "PLE" {
                        # "ple is always saved"
                      }
                    }
                    n1129 = local read "cycle-num"() -> (w1584:i32)
                    n1130 = Less?(x="cycle-iterator", y=w1584) -> (x < y?=w1589:bool)
                    n1131 = case shown="True" w1589 {
                      tunnel: "cycle-iterator" -> [_ w1608]
                      tunnel: [0 w1615] -> w1583
                      tunnel: w1582 -> [_ w1610]
                      tunnel: [i32[] [] w1605] -> w1580
                      frame False {
                        w1594 = FALSE ("measure")
                        # "last cycle"
                        n1132 = local read "NKT"() -> (w1595:bool)
                        n1133 = case shown="True" w1595 {
                          frame False {
                          }
                          frame True {
                            n1134 = local read "NKT Input"() -> (w1599:T7)
                            n1135 = Bundle By Name(cluster=w1599, "Emission"=FALSE ("Emission On/Off")) -> (w1597:T7)
                            n1136 = local write "NKT Input"(w1597) -> ()
                          }
                        }
                        n1137 = local write "measure"(w1594) -> ()
                        n1138 = local write "velleman-power"(w1594) -> ()
                        n1139 = local write "autostage-start"(w1594) -> ()
                      }
                      frame True {
                        n1140 = local read "excitation"() -> (w1609:dbl[][])
                        n1141 = local read "coordinates"() -> (w1614:dbl[][])
                        n1142 = case shown="\"PLE\"" w1610 {
                          frame "spectrum", Default {
                            n1143 = local write "measure"(TRUE ("measure")) -> ()
                          }
                          frame "PLE" {
                            n1144 = local write "Start PLE Scan"(TRUE ("Start PLE Scan")) -> ()
                          }
                        }
                        n1145 = Increment(x=w1608) -> (x+1=w1615:i32)
                        n1146 = Build Array(0 ("element"), w1608) -> (w1605:i32[])
                        n1147 = Index Array(array=w1609, index (row)=0, index (col)=w1608) -> (element=w1604:dbl)
                        n1148 = Index Array(array=w1609, index (row)=1, index (col)=w1608) -> (element=w1603:dbl)
                        n1149 = Build Array(w1604, w1603) -> (w1602:dbl[])
                        n1150 = Not Equal To 0?(x=w1602) -> (x != 0?=w1601:bool[])
                        n1151 = And Array Elements(Boolean array=w1601) -> (logical AND=w1600:bool)
                        n1152 = Index Array(array=w1614, index (row)=0, index (col)=w1608) -> (element=w1613:dbl)
                        n1153 = Index Array(array=w1614, index (row)=1, index (col)=w1608) -> (element=w1612:dbl)
                        n1154 = Index Array(array=w1614, index (row)=2, index (col)=w1608) -> (element=w1611:dbl)
                        n1155 = case shown="True" w1600 {
                          tunnel: w1604 -> [_ w1621]
                          tunnel: w1603 -> [_ w1620]
                          frame False {
                          }
                          frame True {
                            n1156 = local read "NKT Input"() -> (w1623:T7)
                            n1157 = Bundle By Name(cluster=w1623, "Short Wavelength (nm)"=w1621, "Long Wavelength (nm)"=w1620) -> (w1622:T7)
                            n1158 = local write "NKT Input"(w1622) -> ()
                          }
                        }
                        n1159 = local write "z-axis"(w1611) -> ()
                        n1160 = local write "y-axis"(w1612) -> ()
                        n1161 = local write "x-axis"(w1613) -> ()
                      }
                    }
                    n1162 = property on="coordinates" class="Arr (strict)"("Index Values"=w1580) -> ()  [unwired: 2 in, 2 out]
                    n1163 = property on="excitation" class="Arr (strict)"("Index Values"=w1580) -> ()  [unwired: 2 in, 2 out]
                    n1164 = Multiply(x=100 ("cycle-iterator"), y=w1583) -> (x*y=w1588:i32)
                    n1165 = local write "cycle-iterator"(w1583) -> ()
                    n1166 = Divide(x=w1588, y=w1584) -> (x/y=→"Slide":dbl)
                  }
                }
              }
            }
          }
          frame #2 {
            n1167 = case shown="True" "cycle-save-coordinates" {
              frame False {
              }
              frame True {
                n1168 = local read "coordinates"() -> (w1631:dbl[][])
                n1169 = call-poly <vilib>:"Write Delimited Spreadsheet.vi"("format (%.3f)"="%.2f", "2D data"=w1631, "transpose? (F)"=TRUE, "delimiter (\\t)"="," ("delimiter (\\t)")) -> ("error out"=w1627:errorcluster)  [unwired: 10 in, 1 out]
                n1170 = case shown="No Error" w1627 {
                  frame No Error {
                  }
                  frame Error {
                  }
                }
              }
            }
          }
        }
      }
    }
    n1171 = local read "shutdown-active"() -> (w1451:bool)
    n1172 = node-c288() -> ()  [unwired: 1 in, 1 out]
  }
  n1173 = node-c288(w1) -> ()  [unwired: 1 out]
  n1174 = node-c288() -> (w6:T26)  [unwired: 4 in]
  n1175 = timed-loop {
    timing: w6 -> [_]
    timing-out: [_] -> w5
    stop <- w1634 stop-if-true
    n1176 = node-c288() -> ()  [unwired: 1 in, 1 out]
    n1177 = local read "shutdown-complete"() -> (w1635:bool)
    n1178 = case shown="False" w1635 {
      selector: w1635 -> [w1636 w1637]
      tunnel: [w1636 w1637] -> w1634
      frame False {
      }
      frame True {
        # "Reinit Default Values"
        n1179 = control-ref of="This VI"() -> (w1639:refnum<vi>)
        n1180 = invoke class="VI" method="Default Vals.Reinit All"(reference=w1639) -> (reference out=w1638:refnum<vi>)  [unwired: 2 in, 2 out]
        n1181 = Close Reference(reference=w1638) -> ()  [unwired: 1 in, 1 out]
      }
    }
    n1182 = node-c288() -> ()  [unwired: 1 in, 1 out]
  }
  n1183 = node-c288(w5) -> ()  [unwired: 1 out]
  n1184 = node-c288(w17) -> ()  [unwired: 1 out]
  n1185 = node-c288(i64 100 ("Period")) -> (w20:T26)  [unwired: 3 in]
  n1186 = timed-loop {
    timing: w20 -> [_]
    timing-out: [_] -> w19
    stop <- w1642 stop-if-true
    # "save"
    n1187 = node-c288() -> ()  [unwired: 1 in, 1 out]
    n1188 = case shown="False" "Save current Spectrum" {
      frame False {
      }
      frame True {
        w1651 = "the master of microscopy" ("User Name")
        n1189 = local read "select background"() -> (w1660:enum16{"skip", "single", "multiple"})
        n1190 = local read "switch U/D"() -> (w1659:bool)
        n1191 = local read "switch L/R"() -> (w1658:bool)
        n1192 = local read "Exposure Time Read"() -> (w1668:sgl)
        n1193 = local read "Current Detector"() -> (w1664:string)
        n1194 = local write "Save current Spectrum"(FALSE ("Save current Spectrum")) -> ()
        n1195 = local read "readout mode 2"() -> (w1665:u16)
        n1196 = local read "HSSpeed"() -> (w1655:dbl)
        n1197 = local read "y-axis"() -> (w1676:dbl)
        n1198 = local read "z-axis"() -> (w1678:dbl)
        n1199 = local read "pre-amp"() -> (w1654:dbl)
        n1200 = local read "x-axis"() -> (w1677:dbl)
        n1201 = local read "Cooling Read"() -> (w1667:cluster{"iDus":i32, "Newton":i32, "Clara":i32})
        n1202 = local read "spectrograph-output"() -> (w1673:T10)
        n1203 = local read "HBinning"() -> (w1666:u16)
        n1204 = local read "NKT Output"() -> (w1674:T6)
        n1205 = Bundle By Name(cluster=T57 {"BG shutter"=enum."with Open Shutter", "select background"=enum."skip"} ("background"), "BG shutter"="BG shutter", "select background"=w1660) -> (w1661:T57)
        n1206 = Bundle By Name(cluster=T55 {"x-axis"=150.0, "y-axis"=150.0, "z-axis"=150.0, "switch U/D"=TRUE, "switch L/R"=TRUE} ("Nanostage"), "z-axis"=w1678, "x-axis"=w1677, "y-axis"=w1676, "switch U/D"=w1659, "switch L/R"=w1658) -> (w1652:T55)
        n1207 = local read "Pixel Scaling"() -> (w1672:T16)
        n1208 = Bundle By Name(cluster=T56 {"Current Detector"="CCD", "readout mode"=0, "Hbinning"=8, "Exposure Time"=0.2, "Cooling Read"={"iDus"=99, "Newton"=99, "Clara"=99}, "pre-amp"=0.0, "HSSpeed"=0.0} ("Detector"), "pre-amp"=w1654, "HSSpeed"=w1655, "Current Detector"=w1664, "readout mode"=w1665, "Hbinning"=w1666, "Exposure Time"=w1668, "Cooling Read"=w1667) -> (w1656:T56)
        n1209 = local read "image-laser-position"() -> (w1645:T15)
        n1210 = local read "x-scale array"() -> (w1679:sgl[])
        n1211 = local read "Raw Signal Array"() -> (w1681:i32[])
        n1212 = local read "Background Array"() -> (w1680:i32[])
        n1213 = local read "magnification"() -> (w1646:dbl)
        n1214 = local read "Power during measurement"() -> (w1675:dbl)
        n1215 = Bundle By Name(cluster=T59 {"Calibration Mode"=TRUE, "File Name"="File Name:", "User Name"="unknown", "Aborted?"=FALSE, "NKT System"=enum."SuperK Varia (VIS)"} ("general"), "File Name"="File Name", "User Name"=w1651) -> (w1671:T59)
        n1216 = Bundle By Name(cluster=T54 {"image-laser-position"={"laser-x-position"=0, "laser-y-position"=0}, "magnification"=1.0} ("Image Details"), "image-laser-position"=w1645, "magnification"=w1646) -> (w1647:T54)
        n1217 = call "output-save-header.vi"("Image Details"=w1647, "Spectrograph"=w1673, "PLE Excitation Input"=T58 {"Loop Indicator"=0, "Number of Scans"=0, "True Step Size (nm) "=0, "Wavelength Bandpass (nm)"=0, "Min Central Wavelength (nm)"=0}, "Detector"=w1656, "background"=w1661, "Lightsource"=w1674, "Nanostage"=w1652, "Pixel Scaling"=w1672, "general"=w1671) -> ("Header for .txt"=w1684:string, "Header for .ibw"=w1683:string)  [unwired: 1 in]
        n1218 = call "output-save-spectra.vi"("Wavelength Array"=w1679, "Raw Signal Array"=w1681, "Background Array"=w1680, "User Name"=w1651, "NAS Server ok?"=FALSE, "Save?"=TRUE, "Header"=w1684, "Header for .ibw"=w1683, "File Name"="File Name", "Power (µW)"=w1675) -> ()
      }
    }
    n1219 = local read "shutdown-active"() -> (w1642:bool)
    n1220 = node-c288() -> ()  [unwired: 1 in, 1 out]
  }
  n1221 = node-c288(w7) -> ()  [unwired: 1 out]
  n1222 = node-c288() -> (w4:T26)  [unwired: 5 in]
  n1223 = timed-loop {
    timing: w4 -> [_]
    timing-out: [_] -> w3
    stop <- w1691 stop-if-true
    # "PLE only works with the following active"
    # "PLE Measurement"
    # "Adjust NKT Excitation Wavelength Parameters - VIS and UV"
    n1224 = node-c288() -> ()  [unwired: 1 in, 1 out]
    n1225 = local read "powermeter init"() -> (w1687:bool)
    n1226 = local read "lightsource"() -> (w1688:bool)
    n1227 = local read "spectrograph"() -> (w1690:bool)
    n1228 = local read "cameras init"() -> (w1689:bool)
    n1229 = local read "ready"() -> (w1692:bool)
    n1230 = Build Array(w1687, w1688, w1690, w1689, "Start PLE Scan", w1692) -> (w1704:bool[])
    n1231 = And Array Elements(Boolean array=w1704) -> (logical AND=w1702:bool)
    n1232 = Unbundle By Name("PLE Wavelength") -> ("Min WL VIS (nm)"=w1694:i32)
    n1233 = feedback #34(T60 {"Min WL VIS (nm)"=0, "Max WL VIS (nm)"=0, "WL Bandpass (nm)"=0, "WL Stepsize (nm)"=0}) -> (w1699:T63)
    n1234 = feedback-in #34("PLE Wavelength") -> ()
    n1235 = Not Equal?(x="PLE Wavelength", y=w1699) -> (x != y?=w1698:T64)
    n1236 = Cluster To Array(cluster=w1698) -> (array=w1697:bool[])
    n1237 = Or Array Elements(Boolean array=w1697) -> (logical OR=w1696:bool)
    n1238 = case shown="False" w1696 {
      tunnel: [w1710 w1713] -> w1700
      tunnel: "PLE Wavelength" -> [w1711 w1715]
      frame False {
        n1239 = Unbundle By Name(w1711) -> ("Min WL VIS (nm)"=w1708:i32, "WL Bandpass (nm)"=w1706:u16, "WL Stepsize (nm)"=w1705:i32)
        n1240 = local read "Number of Scans"() -> (w1707:i32)
        n1241 = Bundle By Name(cluster=T61 {"Min Central Wavelength (nm)"=500, "Wavelength Bandpass (nm)"=2, "True Step Size (nm) "=2, "Number of Scans"=101} ("Output Cluster for While Loop"), "Min Central Wavelength (nm)"=w1708, "Wavelength Bandpass (nm)"=w1706, "True Step Size (nm)"=w1705, "Number of Scans"=w1707) -> (w1710:T61)
      }
      frame True {
        # "recalculate if values changed"
        n1242 = call "lightsource-wl-correct.vi"("PLE WL Input Cluster"=w1715) -> ("Output Cluster for While Loop"=w1713:T61, "PLE WL Output Cluster"=w1714:T18)  [unwired: 3 in]
        n1243 = Unbundle By Name(w1713) -> ("Number of Scans"=→"Number of Scans":i32)
        n1244 = local write "PLE Wavelength"(w1714) -> ()
      }
    }
    n1245 = case shown="True" w1702 {
      tunnel: w1700 -> [_ w1718]
      tunnel: w1694 -> [_ w1717]
      frame False {
      }
      frame True {
        n1246 = while {
          tunnel: w1718 -> [w1720]
          tunnel: w1717 -> [w1719]
          i -> [w1723]
          stop <- w1722 stop-if-true
          # "Binning Factor"
          # "Bgr with Open Shutter?"
          # "Multiple Bgr?"
          n1247 = Equal To 0?(x=w1723) -> (x = 0?=w1721:bool)
          n1248 = stacked-sequence {
            seq-local: [w1728 _ _] -> [_ w1780 _]
            seq-local: [w1729 _ _] -> [_ w1786 _]
            seq-local: [_ w1779 _] -> [_ _ w2049]
            seq-local: [_ w1778 _] -> [_ _ w2053]
            tunnel: w1720 -> [_ w1787 _]
            tunnel: w1721 -> [w1731 w1785 _]
            tunnel: w1723 -> [_ w1783 _]
            tunnel: [_ _ w2050] -> w1722
            tunnel: w1721 -> [_ w1777 _]
            tunnel: w1719 -> [w1727 _ _]
            frame #0 {
              # "nkt"
              # "powermeter"
              n1249 = local read "BG shutter"() -> (w1726:T2)
              n1250 = local read "select background"() -> (w1724:enum16{"skip", "single", "multiple"})
              n1251 = Equal?(x=w1726, y=T2."with Open Shutter" ("Background Measurement PLE")) -> (x = y?=w1728:bool)
              n1252 = Equal?(x=w1724, y=enum16{"skip", "single", "multiple"}."multiple") -> (x = y?=w1729:bool)
              n1253 = case shown="True" w1731 {
                tunnel: w1728 -> [_ w1734]
                tunnel: w1727 -> [_ w1733]
                tunnel: w1727 -> [_ w1732]
                frame False {
                }
                frame True {
                  n1254 = flat-sequence {
                    tunnel: w1734 -> [w1756]
                    tunnel: w1733 -> [w1766]
                    frame #0 {
                      w1740 = i32[] [] ("Raw Signal Array PLE")
                      w1737 = T31."Enabled" ("Disabled")
                      n1255 = local write "Present Scan"("") -> ()
                      n1256 = local write "Raw Signal Array PLE"(w1740) -> ()
                      n1257 = local write "Background Array PLE"(w1740) -> ()
                      n1258 = property on="STOP PLE" class="Bool (strict)"("DisabledEnum"=w1737) -> ()  [unwired: 2 in, 2 out]
                      n1259 = local write "PLE-Map"(i32[][] [] ("Intensity Graph")) -> ()
                      n1260 = local write "background"(TRUE ("substract background?")) -> ()
                      n1261 = local write "Data Plot"(cluster{"wavelength array":sgl[], "array":i32[]} {"wavelength array"=[], "array"=[]} ("Data Plot")) -> ()
                      n1262 = property on="Present Scan" class="Str"("DisabledEnum"=w1737) -> ()  [unwired: 2 in, 2 out]
                      "PLE Acquisition\nfinished?" <- FALSE ("Acquisition\nPLE finished?")
                    }
                    frame #1 {
                      w1743 = FALSE
                      n1263 = call "velleman-pl.vi"("Power Control"=w1743) -> ("Power Control 2"=w1742:bool)  [unwired: 6 in, 2 out]
                      n1264 = local write "velleman-power"(w1743) -> ()
                      n1265 = local write "velleman-power-status"(w1742) -> ()
                      n1266 = local write "laser on"(w1742) -> ()
                    }
                    frame #2 {
                      n1267 = Wait (ms)(milliseconds to wait=u32 50) -> ()  [unwired: 1 out]
                    }
                    frame #3 {
                      n1268 = local read "NKT Input"() -> (w1748:T7)
                      n1269 = local read "lightsource-visa"() -> (w1746:refnum<visa-resource-name>)
                      n1270 = Bundle By Name(cluster=w1748, "Emission"=TRUE ("Emission On/Off")) -> (w1745:T7)
                      n1271 = call "lightsource-emission-start.vi"("NKT Input"=w1745, "VISA in"=w1746) -> ("NKT Output"=w1749:T65)  [unwired: 1 out]
                      n1272 = local write "NKT Output"(w1749) -> ()
                      n1273 = local write "NKT Input"(w1745) -> ()
                    }
                    frame #4 {
                      n1274 = Wait (ms)(milliseconds to wait=u32 50) -> ()  [unwired: 1 out]
                    }
                    frame #5 {
                      w1759 = 0 ("Device No")
                      n1275 = Boolean To (0,1)(Boolean=w1756) -> (0, 1=w1758:i16)
                      n1276 = local read "spectrograph-input"() -> (w1754:T10)
                      n1277 = local read "spectrograph-output"() -> (w1753:T10)
                      n1278 = flat-sequence {
                        tunnel: w1759 -> [w1762]
                        tunnel: TRUE ("SetShutter") -> [w1761]
                        tunnel: w1758 -> [w1760]
                        tunnel: [w1763] -> _
                        tunnel: w1759 -> [w1764]
                        tunnel: [w1763] -> w1755
                        frame #0 {
                          n1279 = call <userlib>:"shamrock_shutterAction.vi"("Mode"=w1760, "SetShutter"=w1761, "Device No"=w1762) -> ()  [unwired: 1 out]
                        }
                        frame #1 {
                          n1280 = call <userlib>:"shamrock_shutter.vi"("Device No"=w1764) -> ("Shutter"=w1763:i32)  [unwired: 1 in, 5 out]
                        }
                      }
                      n1281 = Bundle By Name(cluster=w1753, "Shutter"=w1755) -> (w1751:T10)
                      n1282 = local write "spectrograph-output"(w1751) -> ()
                      n1283 = Bundle By Name(cluster=w1754, "Shutter"=w1755) -> (w1752:T10)
                      n1284 = local write "spectrograph-input"(w1752) -> ()
                    }
                    frame #6 {
                      n1285 = Wait (ms)(milliseconds to wait=u32 50) -> ()  [unwired: 1 out]
                    }
                    frame #7 {
                      w1768 = TRUE ("Perform Powermeter Auto Zero?")
                      n1286 = local read "powermeter visa"() -> (w1767:refnum<visa-resource-name>)
                      n1287 = call "powermeter-main.vi"("Perform Powermeter Auto Zero?"=w1768, "input-wavelength"=w1766, "Set Wavelength?"=w1768, "VISA in"=w1767) -> ()  [unwired: 1 in, 3 out]
                    }
                  }
                  n1288 = local write "WL Power (nm)"(w1732) -> ()
                }
              }
            }
            frame #1 {
              n1289 = flat-sequence {
                tunnel: [w1797] -> w1779
                tunnel: w1787 -> [w1813]
                tunnel: w1786 -> [w1795]
                tunnel: w1785 -> [w1801]
                tunnel: [w1802] -> w1784
                tunnel: [w1803] -> _
                tunnel: w1783 -> [w1803]
                tunnel: [w1805] -> w1782
                tunnel: [w1806] -> w1781
                tunnel: w1780 -> [w1806]
                tunnel: [w1804] -> w1776
                tunnel: [w1798] -> w1775
                tunnel: [w1799] -> w1774
                tunnel: w1784 -> [w1844]
                tunnel: w1782 -> [w1843]
                tunnel: w1781 -> [w1842]
                tunnel: [w1826] -> w1778
                tunnel: w1777 -> [w1838]
                tunnel: w1776 -> [w1836]
                tunnel: w1775 -> [w1827]
                tunnel: w1774 -> [w1823]
                tunnel: [w1828] -> w1773
                tunnel: [w1827] -> w1772
                tunnel: [w1825] -> w1771
                tunnel: [w1824] -> w1770
                tunnel: [w1822] -> w1769
                tunnel: [w2026] -> _
                tunnel: w1773 -> [w2023]
                tunnel: w1772 -> [w2016]
                tunnel: w1771 -> [w2026]
                tunnel: w1770 -> [w2022]
                tunnel: w1769 -> [w2019]
                frame #0 {
                  n1290 = local read "Current Detector"() -> (w1793:string)
                  n1291 = case shown="\"CCD\", \"Newton\"" w1793 {
                    tunnel: [u16 1 ("f") w1815] -> w1792
                    frame "", Default {
                    }
                    frame "CCD", "Newton" {
                      n1292 = local read "HBinning"() -> (w1815:u16)
                    }
                  }
                  n1293 = Increment(x=w1803) -> (x+1=w1804:i32)
                  n1294 = Unbundle(w1813) -> ("Min Central Wavelength (nm)"=w1812:i32, "Wavelength Bandpass (nm)"=w1811:i32, "True Step Size (nm)"=w1810:i32, "Number of Scans"=w1809:i32)
                  n1295 = local read "NKT Input"() -> (w1791:T7)
                  n1296 = local read "NKT Output"() -> (w1790:T6)
                  n1297 = call <userlib>:"GetDetector.vi"() -> ("xpixels"=w1807:i32)  [unwired: 4 in, 3 out]
                  n1298 = local read "lightsource-visa"() -> (w1794:refnum<visa-resource-name>)
                  n1299 = Bundle("Min Central Wavelength (nm)"=w1812, "Wavelength Bandpass (nm)"=w1811, "True Step Size (nm)"=w1810, "Number of Scans"=w1809, w1803) -> (w1800:T66)  [unwired: 1 in]
                  n1300 = call "lightsource-set.vi"("Excitation Input"=w1800) -> ("PLE Measurment Finished?"=w1797:bool, "Excitation Input"=w1798:T67, "Wavelength Cluster"=w1796:T68, "Powermeter Wavelength (nm)"=w1799:i32)  [unwired: 1 in]
                  n1301 = case shown="False" w1801 {
                    tunnel: w1799 -> [w1816 _]
                    frame False {
                      # "Set Powermeter Wavelength"
                      n1302 = local read "powermeter visa"() -> (w1817:refnum<visa-resource-name>)
                      n1303 = call "powermeter-main.vi"("Perform Powermeter Auto Zero?"=FALSE ("Set Wavelength?"), "input-wavelength"=w1816, "Set Wavelength?"=TRUE ("Perform Powermeter Auto Zero?"), "VISA in"=w1817) -> ("output-wavelength"=w1818:i32)  [unwired: 1 in, 2 out]
                      n1304 = local write "WL Power (nm)"(w1818) -> ()
                    }
                    frame True {
                      n1305 = Wait (ms)(milliseconds to wait=u32 250) -> ()  [unwired: 1 out]
                    }
                  }
                  n1306 = Divide(x=w1807, y=w1792) -> (x/y=w1808:dbl)
                  n1307 = To Unsigned Long Integer(number=w1808) -> (unsigned 32bit integer=w1802:u32)
                  n1308 = call "lightsource-wl-set.vi"("NKT Input Control"=w1791, "Wavelength Cluster"=w1796, "NKT Output Control"=w1790, "VISA in"=w1794, "First Loop?"=w1801) -> ("NKT Input Indicator"=w1789:T7, "NKT Output Indicator"=w1788:T6)  [unwired: 1 in]
                  n1309 = local write "NKT Output"(w1788) -> ()
                  n1310 = local write "NKT Input"(w1789) -> ()
                  n1311 = Or(x=w1795, y=w1801) -> (x .or. y?=w1805:bool)
                }
                frame #1 {
                  n1312 = for {
                    N: 2 -> [w1874]
                    tunnel: w1844 -> [w1885]
                    tunnel: w1836 -> [w1886]
                    tunnel: w1843 -> [w1875]
                    tunnel: [w1882] -> w1841
                    tunnel: w1842 -> [w1881]
                    tunnel: [w1880] -> w1826 mode=indexing
                    tunnel: [w1878] -> w1840 mode=indexing
                    tunnel: w1838 -> [w1877]
                    tunnel: [w1876] -> w1833 mode=indexing
                    i -> [w1884]
                    stop <- w1880 stop-if-true
                    # "i=0: BG\ni=1: Data"
                    n1313 = Not Equal To 0?(x=w1884) -> (x != 0?=w1879:bool)
                    n1314 = Or(x=w1875, y=w1879) -> (x .or. y?=w1883:bool)
                    n1315 = case shown="True" w1883 {
                      tunnel: w1886 -> [_ w1900]
                      tunnel: w1885 -> [_ w1899]
                      tunnel: w1879 -> [w1890 w1898]
                      tunnel: [T62 {"wavelength array"=[], "Data To Plot Array"=[], "Raw Signal Array PLE"=[], "Background Array PLE"=[]} ("Cluster With Stuff 2") w1897] -> w1882
                      tunnel: w1881 -> [_ w1896]
                      tunnel: [FALSE w1895] -> w1880
                      tunnel: w1875 -> [_ w1894]
                      tunnel: [w1890 w1893] -> w1878
                      tunnel: w1877 -> [_ w1892]
                      tunnel: [TRUE w1891] -> w1876
                      frame False {
                        # "True Case:\nAcquire Background Data"
                        # "False Case (here):\nOnly in Single Background Mode if\nSingle BG already acquired"
                      }
                      frame True {
                        n1316 = stacked-sequence {
                          seq-local: [_ _ w1929 _ _] -> [_ _ _ w1966 _]
                          seq-local: [_ _ _ w1970 _] -> [_ _ _ _ w2004]
                          seq-local: [_ _ _ w1969 _] -> [_ _ _ _ w2006]
                          seq-local: [_ _ _ w1968 _] -> [_ _ _ _ w2005]
                          seq-local: [_ _ _ w1964 _] -> [_ _ _ _ w2009]
                          tunnel: w1900 -> [_ _ w1931 w1959 _]
                          tunnel: w1899 -> [_ _ _ w1972 _]
                          tunnel: [_ _ _ _ w2007] -> w1897
                          tunnel: w1898 -> [w1901 _ w1930 w1960 w2008]
                          tunnel: w1896 -> [w1902 _ _ _ _]
                          tunnel: [_ _ _ w1967 _] -> w1895
                          tunnel: w1894 -> [w1903 _ _ _ _]
                          tunnel: [_ _ _ _ w2008] -> w1893
                          tunnel: w1892 -> [_ _ _ w1962 _]
                          tunnel: [_ _ w1929 _ _] -> w1891
                          frame #0 {
                            n1317 = case shown="False" w1903 {
                              tunnel: w1902 -> [_ w1905]
                              tunnel: w1901 -> [_ w1904]
                              frame False {
                              }
                              frame True {
                                n1318 = stacked-sequence {
                                tunnel: w1905 -> [_ _ w1910 _]
                                tunnel: w1904 -> [w1906 _ w1909 _]
                                frame #0 {
                                n1319 = call "velleman-pl.vi"("Power Control"=w1906) -> ("Power Control 2"=w1907:bool)  [unwired: 6 in, 2 out]
                                n1320 = local write "velleman-power"(w1906) -> ()
                                n1321 = local write "velleman-power-status"(w1907) -> ()
                                n1322 = local write "laser on"(w1907) -> ()
                                }
                                frame #1 {
                                n1323 = Wait (ms)(milliseconds to wait=u32 50) -> ()  [unwired: 1 out]
                                }
                                frame #2 {
                                n1324 = case shown="False" w1910 {
                                tunnel: w1909 -> [w1911 _]
                                frame False {
                                w1916 = 0
                                n1325 = Boolean To (0,1)(Boolean=w1911) -> (0, 1=w1914:i16)
                                n1326 = local read "spectrograph-input"() -> (w1919:T10)
                                n1327 = local read "spectrograph-output"() -> (w1917:T10)
                                n1328 = flat-sequence {
                                tunnel: w1914 -> [w1922]
                                tunnel: TRUE ("SetShutter") -> [w1921]
                                tunnel: w1916 -> [w1920]
                                tunnel: [w1924] -> w1912
                                tunnel: w1916 -> [w1923]
                                frame #0 {
                                n1329 = call <userlib>:"shamrock_shutterAction.vi"("Mode"=w1922, "SetShutter"=w1921, "Device No"=w1920) -> ()  [unwired: 1 out]
                                }
                                frame #1 {
                                n1330 = call <userlib>:"shamrock_shutter.vi"("Device No"=w1923) -> ("Shutter"=w1924:i32)  [unwired: 1 in, 5 out]
                                }
                                }
                                n1331 = Bundle By Name(cluster=w1917, "Shutter"=w1912) -> (w1918:T10)
                                n1332 = local write "spectrograph-output"(w1918) -> ()
                                n1333 = Bundle By Name(cluster=w1919, "Shutter"=w1912) -> (w1913:T10)
                                n1334 = local write "spectrograph-input"(w1913) -> ()
                                }
                                frame True {
                                }
                                }
                                }
                                frame #3 {
                                n1335 = Wait (ms)(milliseconds to wait=u32 50) -> ()  [unwired: 1 out]
                                }
                                }
                              }
                            }
                          }
                          frame #1 {
                            # "Start Acquisition"
                            n1336 = call <userlib>:"GetStatus.vi"() -> ("status"=w1926:T19)  [unwired: 3 in, 2 out]
                            "Acquisition Status PLE" <- w1926
                            n1337 = Equal?(x=Error_Code_Enum_typedef."DRV_IDLE" ("Acquisition Status"), y=w1926) -> (x = y?=w1927:bool)
                            n1338 = case shown="True" w1927 {
                              frame False {
                              }
                              frame True {
                                n1339 = call <userlib>:"StartAcquisition.vi"() -> ()  [unwired: 2 in, 2 out]
                              }
                            }
                          }
                          frame #2 {
                            n1340 = while {
                              tunnel: w1931 -> [w1936]
                              tunnel: [w1935] -> w1929
                              tunnel: w1930 -> [w1934]
                              i -> [w1950]
                              stop <- w1947 continue-if-true
                              # "Acquire Data"
                              n1341 = call <userlib>:"GetStatus.vi"() -> ("status"=w1943:T19)  [unwired: 3 in, 2 out]
                              n1342 = Number To Decimal String(number=w1936) -> (decimal integer string=w1941:string)  [unwired: 1 in]
                              n1343 = local write "Acquisition Status PLE"(w1943) -> ()
                              n1344 = local read "Exposure Time Read"() -> (w1946:sgl)
                              n1345 = call <vilib>:"Space Constant.vi"() -> ("String"=w1938:string)
                              n1346 = case shown="True" "STOP PLE" {
                                tunnel: [w1952 w1954] -> w1948
                                tunnel: [w1952 w1954] -> w1935
                                frame False {
                                w1952 = TRUE
                                }
                                frame True {
                                n1347 = call <userlib>:"AbortAcquisition.vi"() -> ("DLL error code"=w1956:u32)  [unwired: 2 in, 1 out]
                                n1348 = local write "STOP PLE"(FALSE ("STOP PLE")) -> ()
                                n1349 = Equal?(x=w1956, y=u32 20002 ("= temperature\naccepted")) -> (x = y?=w1955:bool)
                                n1350 = Not(x=w1955) -> (.not. x?=w1954:bool)
                                }
                              }
                              n1351 = Concatenate Strings(w1938, "bg") -> (w1932:string)
                              n1352 = Equal?(x=Error_Code_Enum_typedef."DRV_ACQUIRING" ("Acquisition Status"), y=w1943) -> (x = y?=w1949:bool)
                              n1353 = Select(t="", s=w1934, f=w1932) -> (s? t:f=w1939:string)
                              n1354 = And(x=w1948, y=w1949) -> (x .and. y?=w1947:bool)
                              n1355 = Concatenate Strings(w1941, w1939) -> (→"Present Scan":string)
                              n1356 = call "detector-exposuretime-read.vi"("Loop Indicator"=w1950, "Exposure Time (s)"=w1946) -> ("Progress"=→"Progress":dbl, "Elapsed Time (s)"=→"Elapsed Time (s)":dbl)
                            }
                          }
                          frame #3 {
                            # "Get Acquired Data"
                            n1357 = call <userlib>:"GetAcquiredData.vi"("size"=w1972) -> ("array"=w1971:i32[])  [unwired: 2 in, 2 out]
                            n1358 = Not(x=w1960) -> (.not. x?=w1965:bool)
                            n1359 = local read "autoscale"() -> (w1958:bool)
                            n1360 = And(x=w1965, y=w1962) -> (x .and. y?=w1964:bool)
                            n1361 = And(x=w1958, y=w1960) -> (x .and. y?=w1963:bool)
                            n1362 = Or(x=w1963, y=w1962) -> (x .or. y?=w1961:bool)
                            n1363 = case shown="True" w1966 {
                              tunnel: [w1973 w1985] -> w1968
                              tunnel: w1971 -> [_ w1984]
                              tunnel: [w1973 w1983] -> w1969
                              tunnel: [w1973 w1982] -> w1970
                              tunnel: w1960 -> [_ w1981]
                              tunnel: w1964 -> [_ w1980]
                              tunnel: w1961 -> [_ w1979]
                              tunnel: w1959 -> [w1976 _]
                              frame False {
                                w1973 = i32[] [] ("Background Array PLE")
                                n1364 = Decrement(x=w1976) -> (x-1=w1975:i32)
                                n1365 = Number To Decimal String(number=w1975) -> (decimal integer string=w1974:string)  [unwired: 1 in]
                                n1366 = local write "Elapsed Time (s)"(0.0 ("Elapsed Time (s)")) -> ()
                                n1367 = local write "Progress"(0.0 ("Progress")) -> ()
                                n1368 = local write "Present Scan"(w1974) -> ()
                              }
                              frame True {
                                n1369 = stacked-sequence {
                                seq-local: [w1988 _] -> [_ w1998]
                                tunnel: [_ w1994] -> w1982
                                tunnel: [_ w1996] -> w1983
                                tunnel: [_ w1995] -> w1985
                                tunnel: w1984 -> [w1987 _]
                                tunnel: w1981 -> [w1986 _]
                                tunnel: w1980 -> [_ w1993]
                                tunnel: w1979 -> [_ w1991]
                                frame #0 {
                                n1370 = case shown="True" w1986 {
                                tunnel: w1987 -> [w1989 w1990]
                                frame False {
                                "Background Array PLE" <- w1989
                                }
                                frame True {
                                "Raw Signal Array PLE" <- w1990
                                }
                                }
                                n1371 = local read "background"() -> (w1988:bool)
                                }
                                frame #1 {
                                n1372 = local read "Raw Signal Array PLE"() -> (w1996:i32[])
                                n1373 = local read "Background Array PLE"() -> (w1995:i32[])
                                n1374 = Subtract(x=w1996, y=w1995) -> (x-y=w1997:i32[])
                                n1375 = Select(t=w1997, s=w1998, f=w1996) -> (s? t:f=w1994:i32[])
                                n1376 = Select(t=w1995, s=w1993, f=w1994) -> (s? t:f=w1992:i32[])
                                n1377 = case shown="True" w1991 {
                                tunnel: w1992 -> [_ w2001]
                                frame False {
                                }
                                frame True {
                                n1378 = Array Max & Min(array=w2001) -> (max value=w2000:i32, min value=w1999:i32)  [unwired: 2 out]
                                n1379 = property on="Data Plot" class="XYGraph (strict)"("YScale.Maximum"=w2000, "YScale.Minimum"=w1999) -> ()  [unwired: 2 in, 2 out]
                                }
                                }
                                }
                                }
                              }
                            }
                            n1380 = Not(x=w1966) -> (.not. x?=w1967:bool)
                          }
                          frame #4 {
                            # "Wavelength Array"
                            # "Data to Plot Array"
                            # "Background Array"
                            # "Raw Signal Array"
                            # "Build Cluster with Acquired Data"
                            n1381 = case shown="False" w2009 {
                              tunnel: w2005 -> [_ w2012]
                              frame False {
                              }
                              frame True {
                                n1382 = local read "x-scale array"() -> (w2011:sgl[])
                                n1383 = Bundle("x-scale array"=w2011, "Background Array PLE"=w2012) -> (w2010:T69)  [unwired: 1 in]
                                n1384 = local write "Data Plot"(w2010) -> ()
                              }
                            }
                            n1385 = local read "x-scale array"() -> (w2002:sgl[])
                            n1386 = Bundle(cluster=T62 {"wavelength array"=[], "Data To Plot Array"=[], "Raw Signal Array PLE"=[], "Background Array PLE"=[]} ("Cluster With Stuff 2"), "wavelength array"=w2002, "Data To Plot Array"=w2004, "Raw Signal Array PLE"=w2006, "Background Array PLE"=w2005) -> (w2007:T62)
                          }
                        }
                      }
                    }
                    "PLE loop count" <- w1874
                  }
                  n1387 = Unbundle(w1841) -> ("wavelength array"=w1831:sgl[], "Data To Plot Array"=w1837:i32[], "Raw Signal Array PLE"=w1828:i32[], "Background Array PLE"=w1824:i32[])
                  n1388 = Or Array Elements(Boolean array=w1826) -> (logical OR=w1825:bool)
                  n1389 = And Array Elements(Boolean array=w1833) -> (logical AND=w1832:bool)
                  n1390 = Index Array(array=w1840, index=1) -> (element=w1834:bool)
                  n1391 = Subtract(x=w1828, y=w1824) -> (x-y=w1830:i32[])
                  n1392 = And(x=w1832, y=w1834) -> (x .and. y?=w1835:bool)
                  n1393 = case shown="True" w1835 {
                    tunnel: w1831 -> [_ w1857]
                    tunnel: w1837 -> [_ w1856]
                    tunnel: w1827 -> [_ w1858]
                    tunnel: w1831 -> [_ w1853]
                    tunnel: w1830 -> [_ w1852]
                    tunnel: w1823 -> [_ w1846]
                    tunnel: [nan w1850] -> w1822
                    frame False {
                    }
                    frame True {
                      w1849 = FALSE ("Set Wavelength?")
                      n1394 = Bundle("wavelength array"=w1857, "Data To Plot Array"=w1856) -> (w1848:T70)  [unwired: 1 in]
                      n1395 = local read "powermeter visa"() -> (w1847:refnum<visa-resource-name>)
                      n1396 = call "ouput-plot-ple.vi"("Input Cluster"=w1858, "Data Array"=w1852, "Wavelength Array"=w1853) -> ("Intensity Graph"=w1854:i32[][], "Cluster with Scaling Information"=w1851:T71)  [unwired: 1 out]
                      n1397 = for {
                        N: 2 -> [_]
                        tunnel: w1851 -> [w1860]
                        tunnel: w1854 -> [w1859]
                        n1398 = flat-sequence {
                          tunnel: w1860 -> [w1872]
                          tunnel: w1859 -> [w1873]
                          frame #0 {
                            n1399 = Unbundle(w1872) -> ("Y Scale.Flipped"=w1871:bool, "color table"=w1870:u32[], w1869:dbl, w1868:dbl, w1861:dbl, w1862:dbl, w1863:sgl, w1864:sgl, w1865:sgl, w1866:dbl, "new picture"=w1867:picture)
                            n1400 = property on="PLE-Map" class="IntGraph (strict)"("YScale.Flipped"=w1871, "Color Table"=w1870, "YScale.Maximum"=w1869, "YScale.Minimum"=w1868, "YScale.Multiplier"=w1861, "YScale.Offset"=w1862, "XScale.Maximum"=w1863, "XScale.Minimum"=w1864, "XScale.Multiplier"=w1865, "XScale.Offset"=w1866, "PlotImages.Front"=w1867) -> ()  [unwired: 2 in, 2 out]
                          }
                          frame #1 {
                            "PLE-Map" <- w1873
                          }
                        }
                      }
                      n1401 = call "powermeter-main.vi"("Perform Powermeter Auto Zero?"=w1849, "input-wavelength"=w1846, "Set Wavelength?"=w1849, "VISA in"=w1847) -> ("power (µW)"=w1850:dbl)  [unwired: 1 in, 2 out]
                      n1402 = local write "Data Plot"(w1848) -> ()
                      n1403 = local write "Power (µW)"(w1850) -> ()
                    }
                  }
                }
                frame #2 {
                  (unwired) TRUE ("Save?")
                  n1404 = local read "switch U/D"() -> (w2032:bool)
                  n1405 = local read "switch L/R"() -> (w2031:bool)
                  n1406 = local read "BG shutter"() -> (w2041:T2)
                  n1407 = local read "y-axis"() -> (w2033:dbl)
                  n1408 = local read "z-axis"() -> (w2035:dbl)
                  n1409 = local read "x-axis"() -> (w2034:dbl)
                  n1410 = local read "spectrograph-output"() -> (w2037:T10)
                  n1411 = local read "NKT Output"() -> (w2036:T6)
                  n1412 = Bundle By Name(cluster=T55 {"x-axis"=150.0, "y-axis"=150.0, "z-axis"=150.0, "switch U/D"=TRUE, "switch L/R"=TRUE} ("Nanostage"), "z-axis"=w2035, "x-axis"=w2034, "y-axis"=w2033, "switch U/D"=w2032, "switch L/R"=w2031) -> (w2013:T55)
                  n1413 = Bundle By Name(cluster=T57 {"BG shutter"=enum."with Open Shutter", "select background"=enum."skip"} ("background"), "BG shutter"=w2041, "select background"="select background") -> (w2048:T57)
                  n1414 = local read "Exposure Time Read"() -> (w2042:sgl)
                  n1415 = local read "Current Detector"() -> (w2046:string)
                  n1416 = local read "Pixel Scaling"() -> (w2038:T16)
                  n1417 = local read "readout mode 2"() -> (w2045:u16)
                  n1418 = local read "pre-amp"() -> (w2029:dbl)
                  n1419 = local read "HSSpeed"() -> (w2028:dbl)
                  n1420 = local read "Cooling Read"() -> (w2043:cluster{"iDus":i32, "Newton":i32, "Clara":i32})
                  n1421 = local read "HBinning"() -> (w2044:u16)
                  n1422 = Bundle By Name(cluster=T56 {"Current Detector"="no detector", "readout mode"=0, "Hbinning"=1, "Exposure Time"=0.0, "Cooling Read"={"iDus"=99, "Newton"=99, "Clara"=99}, "pre-amp"=9.0, "HSSpeed"=9.0} ("Detector"), "HSSpeed"=w2028, "pre-amp"=w2029, "Current Detector"=w2046, "readout mode"=w2045, "Hbinning"=w2044, "Exposure Time"=w2042, "Cooling Read"=w2043) -> (w2027:T56)
                  n1423 = local read "x-scale array"() -> (w2025:sgl[])
                  n1424 = local write "Background Array"(w2022) -> ()
                  n1425 = local write "Raw Signal Array"(w2023) -> ()
                  n1426 = Bundle By Name(cluster=T59 {"Calibration Mode"=FALSE, "File Name"="File Name:", "User Name"="unknown", "Aborted?"=FALSE, "NKT System"=enum."SuperK Varia (VIS)"} ("general"), "File Name"="PLE File Name", "Aborted?"=w2026) -> (w2039:T59)
                  n1427 = call "output-save-header.vi"("Spectrograph"=w2037, "PLE Excitation Input"=w2016, "Detector"=w2027, "background"=w2048, "Lightsource"=w2036, "Nanostage"=w2013, "Pixel Scaling"=w2038, "general"=w2039) -> ("Header for .txt"=w2021:string, "Header for .ibw"=w2020:string)  [unwired: 2 in]
                  n1428 = call "output-save-ple.vi"("Wavelength Array"=w2025, "Measurement Aborted?"=w2026, ".txt Header"=w2021, ".ibw Header"=w2020, "NAS Server ok?"=FALSE, "File Name"="PLE File Name", "Raw Signal Array"=w2023, "Power (µW)"=w2019, "Background Array"=w2022, "Excitation Input"=w2016, "select background"="select background", "User Name"="the master") -> ()  [unwired: 4 in]
                }
              }
            }
            frame #2 {
              n1429 = Build Array (concatenate)(w2053, w2049) -> (w2052:bool[])
              n1430 = Or Array Elements(Boolean array=w2052) -> (logical OR=w2051:bool)
              n1431 = case shown="True" w2051 {
                selector: w2051 -> [w2054 w2060]
                tunnel: [w2054 w2060] -> w2050
                tunnel: w2049 -> [_ w2056]
                frame False {
                }
                frame True {
                  n1432 = local read "NKT Input"() -> (w2058:T7)
                  n1433 = Not(x=w2056) -> (.not. x?=w2055:bool)
                  n1434 = local write "PLE Acquisition\nfinished?"(w2056) -> ()
                  n1435 = local write "velleman-power"(FALSE ("velleman-power")) -> ()
                  n1436 = Bundle By Name(cluster=w2058, "Emission"=w2055) -> (w2057:T7)
                  n1437 = local write "NKT Input"(w2057) -> ()
                }
              }
            }
          }
        }
        n1438 = local write "Start PLE Scan"(FALSE ("Start PLE Scan")) -> ()
      }
    }
    n1439 = property on="STOP PLE" class="Bool (strict)"("DisabledEnum"=T31."Disabled and Grayed Out" ("Disabled")) -> ()  [unwired: 2 in, 2 out]
    n1440 = local read "shutdown-active"() -> (w1691:bool)
    n1441 = node-c288() -> ()  [unwired: 1 in, 1 out]
  }
  n1442 = node-c288(w19) -> ()  [unwired: 1 out]
  n1443 = node-c288(w3) -> ()  [unwired: 1 out]
